vi "SubMatrixB.vi"(0 "Target Field, T":dbl=1.0 min=-4.0 max=4.0 step=0.1 format="%.4f", 2 "Sweep rate, T/min":dbl=0.1 min=0.0 max=1.0 step=0.01 format="%.4f", 3 "Custom Folder":string, 4 "Time Stamp":timestamp) -> ()   [LabVIEW 2015]
uses:
  <vilib>/Utility/file.llb/Write To Spreadsheet File (DBL).vi
panel:
  out "IndexB":i32
  out "PrevB":dbl
  out "Communication":string
  out "Comments":string[](array[string])
  out "ArrayBoolian":bool[][](array[boolean])
  out "Numeric 4":i32
  in  "Commutator":bool
  in  "Commute SorceMeter":enum32{"Radio Selection 1", "Radio Selection 2"}(radio)
  out "Numeric 3":i32
  in  "Channel 2 (Vnano3b)":bool
  in  "Channel 1 (Vnano3)":bool
  out "Numeric":i32
  in  "Capacitance (C) and Loss (L)":bool
  in  "Magnetic Field (B)":bool=TRUE
  in  "Current (Ik3)":bool
  in  "Voltage (Vk3)":bool
  in  "Current (Ik2)":bool
  in  "Voltage (Vk2)":bool
  in  "Channel 2 (Vnano2b)":bool
  in  "Channel 1 (Vnano2)":bool
  in  "Thermometer 1 (T1)":bool=TRUE
  in  "Channel 2 (Vnano1b)":bool
  in  "Channel 1 (Vnano1)":bool
  in  "Current (Ik1)":bool=TRUE
  in  "Voltage (Vk1)":bool=TRUE
  out "Numeric Current":dbl
  out "Delib Time delay":i32=500
  in  "points at each Vg":i32=1
  out "XY Graph":cluster{dbl[], dbl[]}(graph)={[1.0, 0.8, 0.6000000000000001, 0.4000000000000001, 0.20000000000000007, 5.551115123125783e-17, -0.19999999999999996, -0.39999999999999997, -0.6, -0.8, -1.0], [0.03352775, 0.056811, 0.03911575, 0.04330675, -0.02468015, 0.011641600000000002, 0.10151450000000001, 0.12386675000000001, 0.08288825000000001, -0.00186266, -0.038650000000000004]}
  in  "Time btw \npoints, sec":dbl=1.0 format="%.2f"
  out "Array 2":dbl[][](array[numeric])
  out "array for data":dbl[](array[numeric])
  out "Array":string[](array[string])
  in  "Addr 1 lock-in oop":bool=TRUE
  in  "Ring":u16(ring) caption="Y-axis:" items=["B0", "I", "R1", "R1oop", "Vk1", "Ik1", "T1", "B"]
  out "String":string
  out "Data file:":path
  in  "error in (no error)":errorcluster
  in  "Ring 3":u16(ring)=1 items=["1 kOhm", "10 kOhm", "100 kOhm", "1 Mohm", "10 mOhm"]
  in  "Ring 2":u16(ring)=4 items=["1 kOhm", "10 kOhm", "100 kOhm", "1 Mohm", "10 mOhm"]
  in  "Fixed Current mkA":dbl=1.0
  in  "Current is:":T1(radio)
  in  "Ressitance measurements?":bool=TRUE
  in  "Addr 5 lock-in oop":bool
  in  "Addr 4 lock-in oop":bool
  in  "Addr 3 lock-in oop":bool
  in  "Addr 2 lock-in oop":bool
  in  "Addr 5 lock-in":bool
  in  "Addr 4 lock-in":bool
  in  "Addr 3 lock-in":bool
  in  "Addr 2 lock-in":bool
  in  "Addr 1 lock-in":bool=TRUE
  # "Keithley 2400: address 12"
  # "0"
  # "SourceMeters"
  # "Nanovoltmeters"
  # "Temperature"
  # "Main"
  # "Magnetic Field"
  # "(not recommended, too slow)"
  # "Capacitance & Loss"
  # "(not recommended, too slow)"
  # "(not recommended, too slow)"
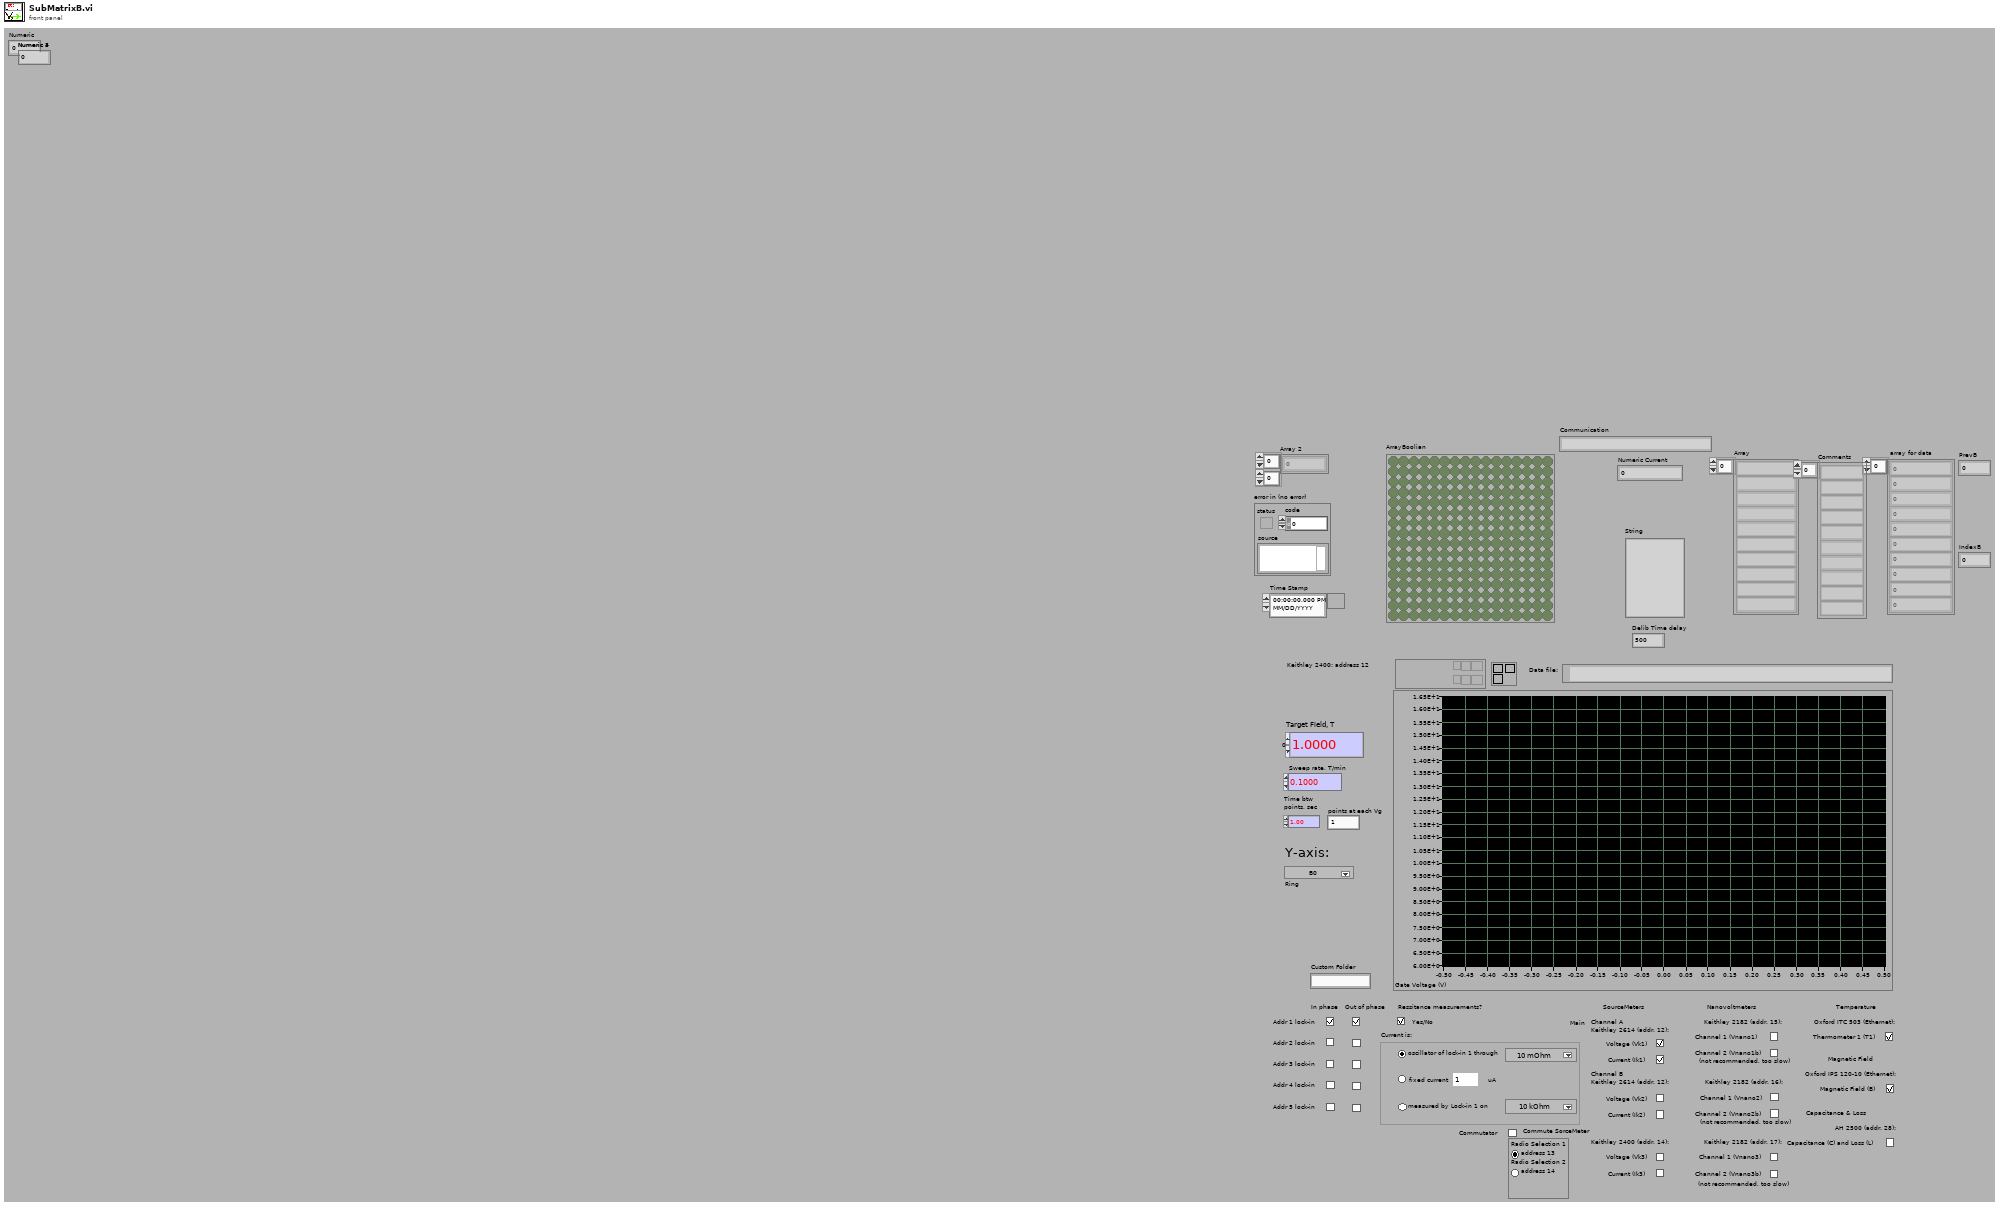
[diagram p1: front panel]
types:
  T1 = enum32{"Radio Selection 1", "Radio Selection 2", "Radio Selection 3"}
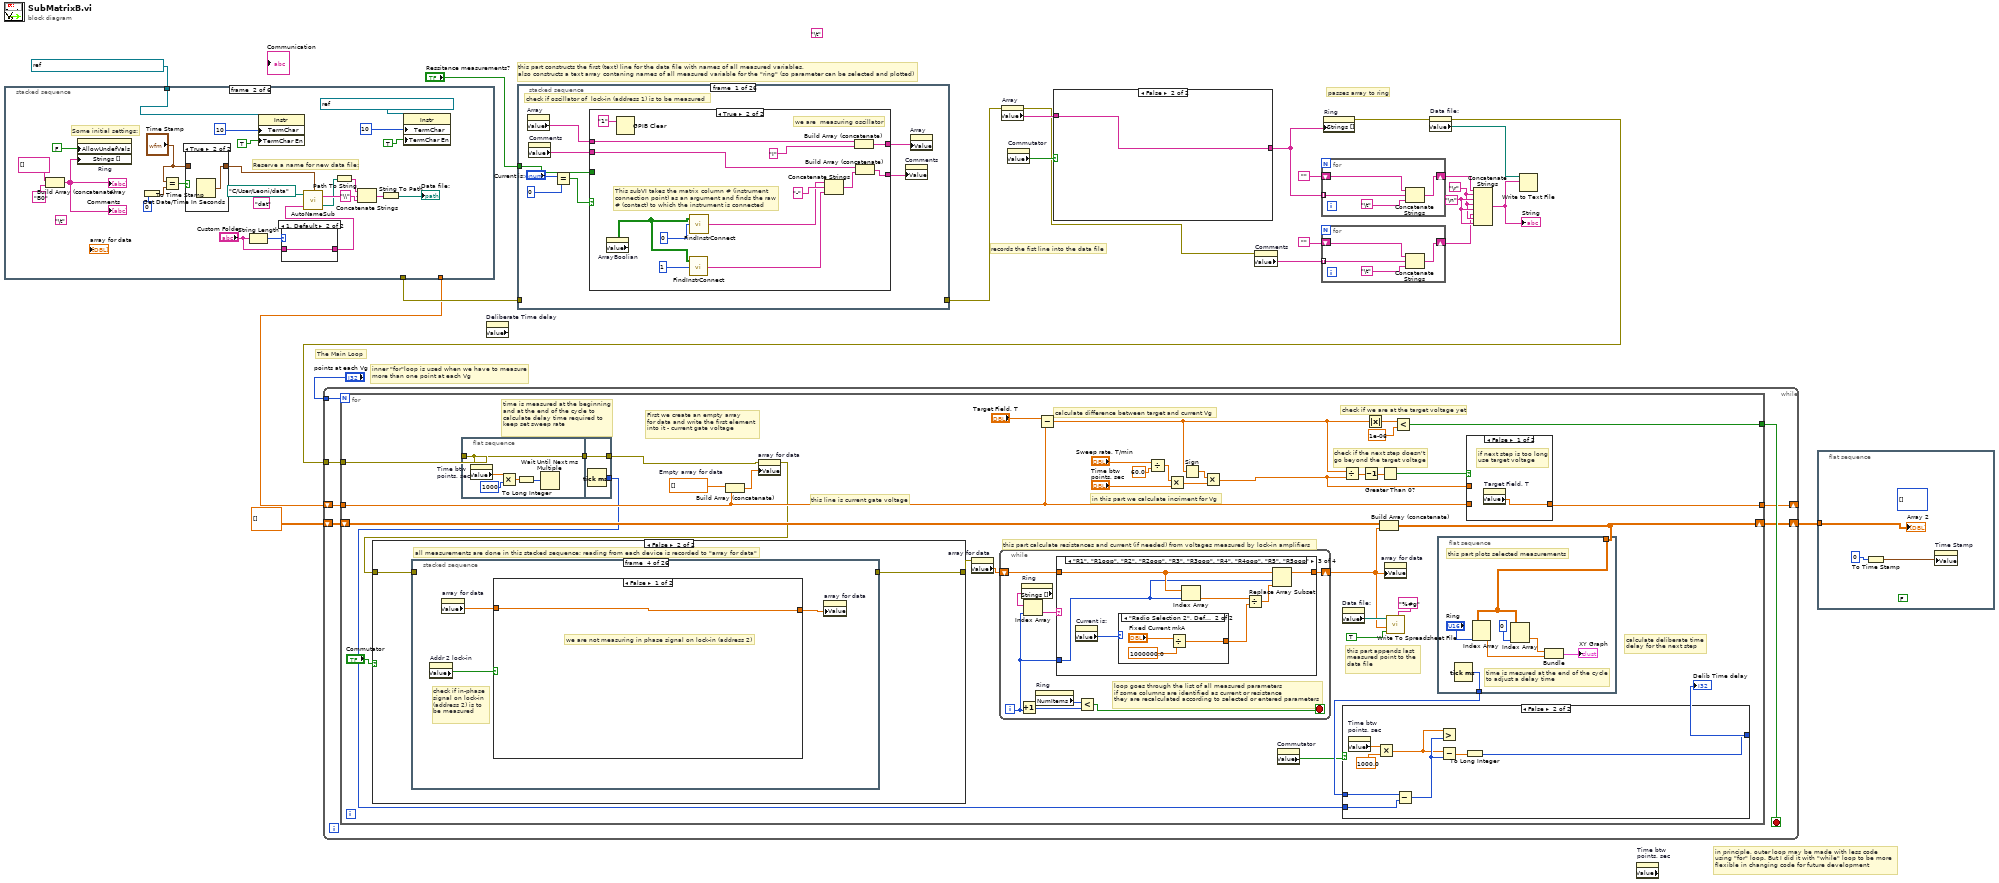
[diagram p0: block diagram]
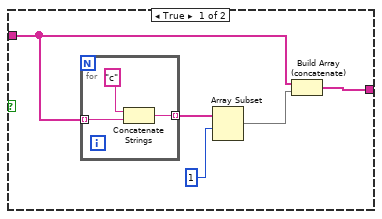
[diagram p2: hidden frame]
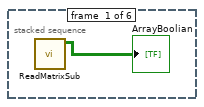
[diagram p3: hidden frame]
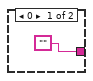
[diagram p5: hidden frame]
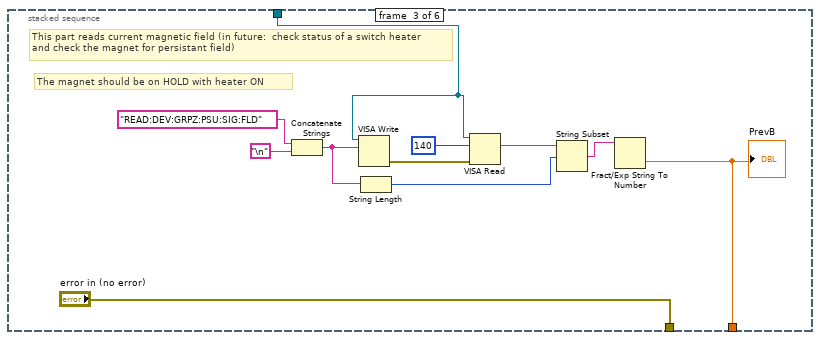
[diagram p6: hidden frame]
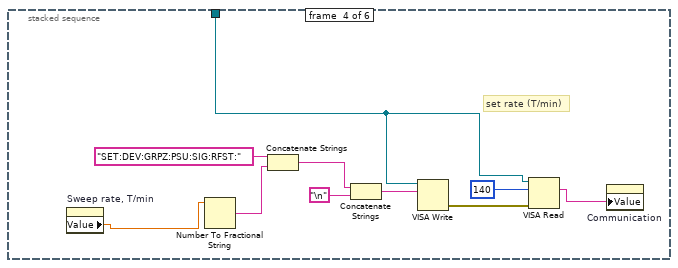
[diagram p7: hidden frame]
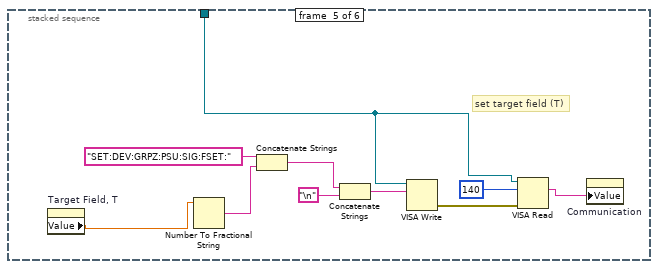
[diagram p8: hidden frame]
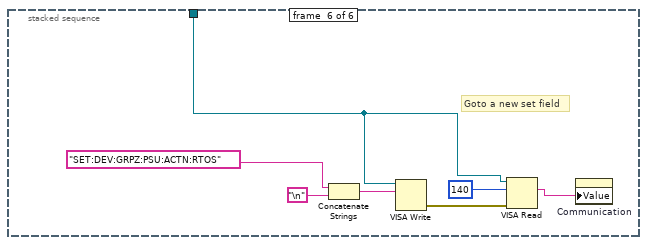
[diagram p9: hidden frame]
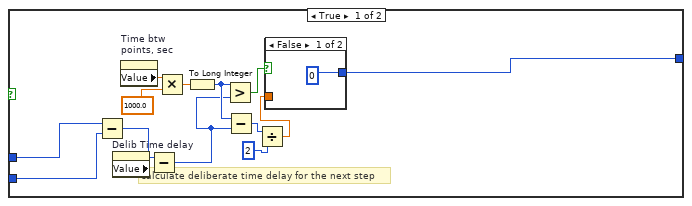
[diagram p10: hidden frame]
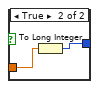
[diagram p11: hidden frame]
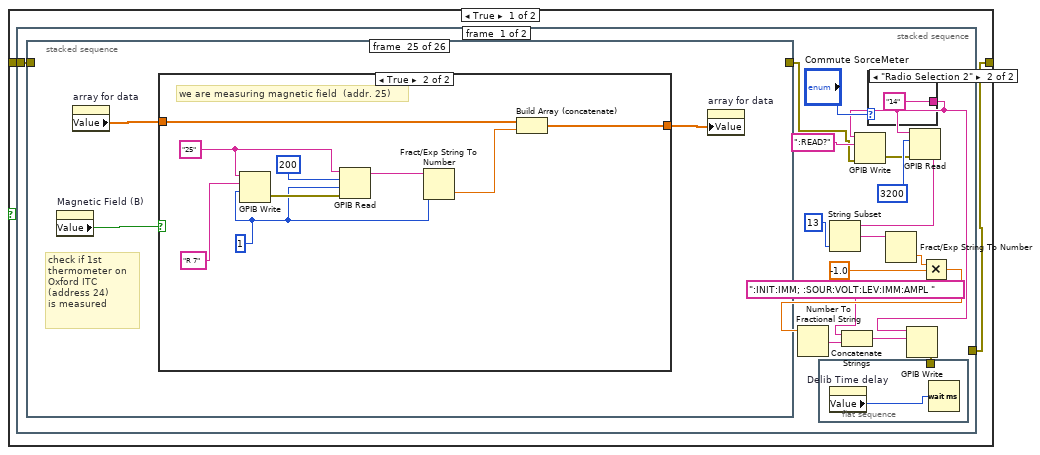
[diagram p12: hidden frame]
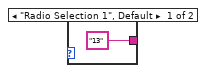
[diagram p13: hidden frame]
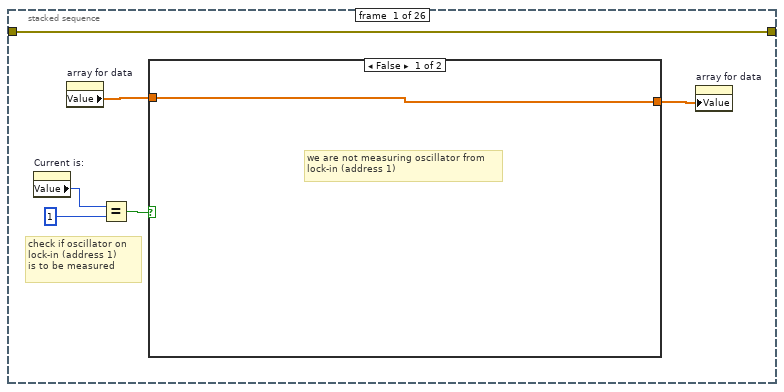
[diagram p14: hidden frame]
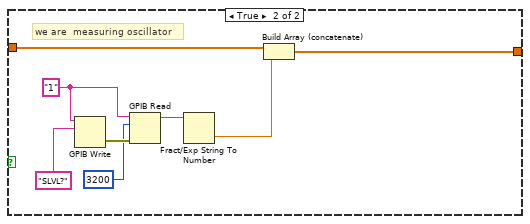
[diagram p15: hidden frame]
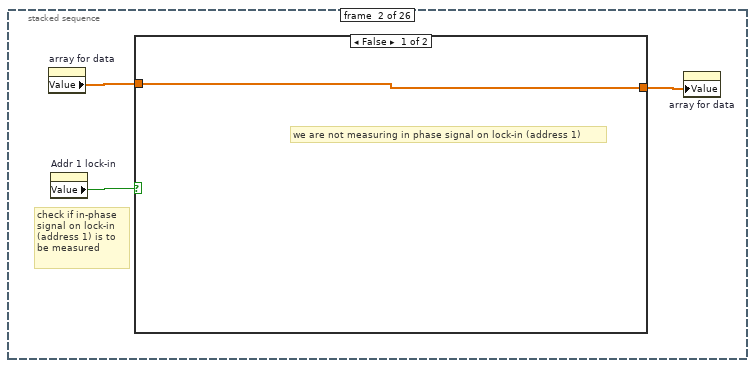
[diagram p16: hidden frame]
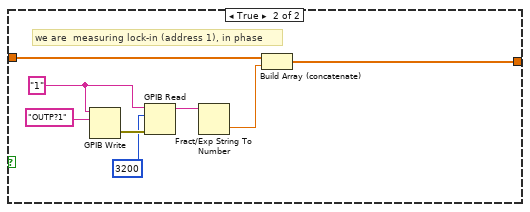
[diagram p17: hidden frame]
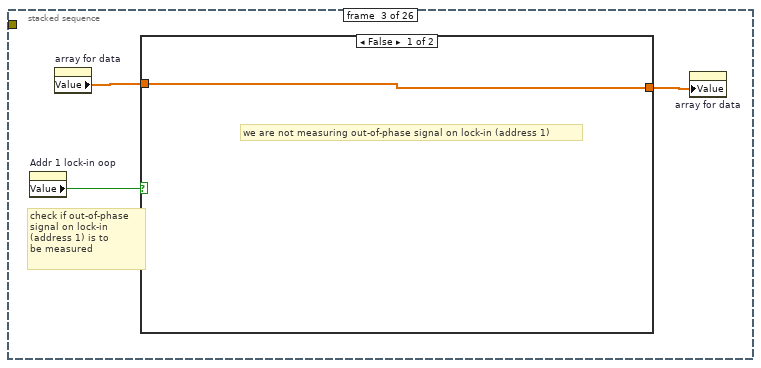
[diagram p18: hidden frame]
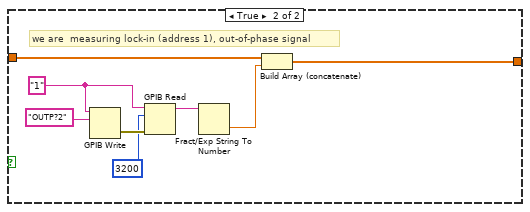
[diagram p19: hidden frame]
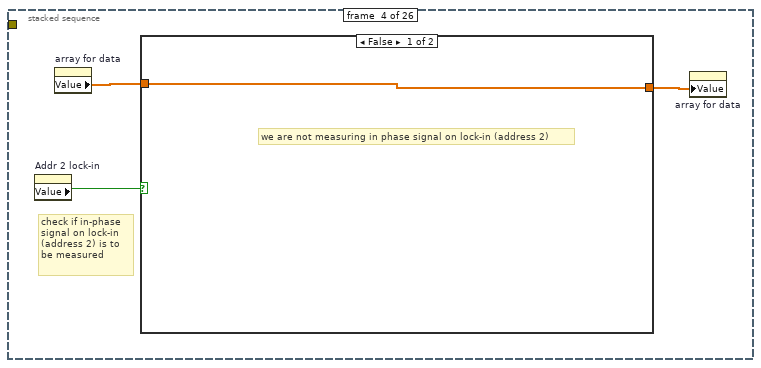
[diagram p20: hidden frame]
diagram:
  (unwired) "\t"
  w5 = "\r"
  w6 = "\n"
  # "passes array to ring"
  # "in principle, outer loop may be made with less code\nusing \"for\" loop. But I did it with \"while\" loop to be more \nflexible in changing code for future development"
  # "inner \"for\"loop is used when we have to measure\nmore than one point at each Vg"
  # "The Main Loop"
  # "records the fist line into the data file"
  # "this part constructs the first (text) line for the data file with names of all measured variables,\nalso constructs a text array contaning names of all measured variable for the \"ring\" (so parameter can be selected and plotted)"
  n1 = stacked-sequence {
    tunnel: [_ _ "error in (no error)" _ _ _] -> w23
    tunnel: refnum<visa-resource-name> "TCPIP0::192.168.128.3::7020::SOCKET" ("VISA resource name") -> [_ w30 w55 w66 w77 w87]
    tunnel: [_ _ w54 _ _ _] -> w1
    frame #0 {
      n2 = call "ReadMatrixSub.vi"() -> ("Array"=→"ArrayBoolian":bool[][])  [unwired: 9 in, 2 out]
    }
    frame #1 {
      (unwired) "dat"
      (unwired) "\t"
      # "Some initial settings:"
      # "Reserve a name for new data file:"
      n3 = Build Array (concatenate)(string[] [], "B0") -> (w31:string[])
      "Array" <- w31
      "Comments" <- w31
      n4 = property on="Ring" class="Ring (strict)"("AllowUndefVals"=FALSE, "Strings []"=w31) -> ()  [unwired: 2 in, 2 out]
      n5 = To Time Stamp(1:0) -> (0:w28:timestamp)
      n6 = Equal?(x="Time Stamp", y=w28) -> (x = y?=w29:bool)
      n7 = case shown="True" w29 {
        tunnel: "Time Stamp" -> [w50 _]
        tunnel: [w50 w51] -> w25
        frame False {
        }
        frame True {
          n8 = Get Date/Time In Seconds() -> (seconds since 1Jan1904=w51:timestamp)
        }
      }
      n9 = String Length(string="Custom Folder") -> (length=w40:i32)
      n10 = property class="Instr"(reference=w30, "TermChar"=10, "TermChar En"=TRUE) -> ()  [unwired: 1 in, 2 out]
      n11 = case shown="1, Default" w40 {
        tunnel: "Custom Folder" -> [_ w53]
        tunnel: ["" w53] -> w38
        frame 0 {
        }
        frame 1, Default {
        }
      }
      n12 = call "AutoNameSub.vi"("Time Stamp"=w25, "Custom Folder"=w38, "User Data Folder"=path "C:/User/Leoni/data") -> ("created path"=w48:path, "String"=w49:string)  [unwired: 1 in]
      n13 = Path To String(path=w48) -> (string=w43:string)
      n14 = Concatenate Strings(w43, "\\", w49) -> (w45:string)
      n15 = String To Path(string=w45) -> (path=→"Data file:":path)
      n16 = property class="Instr"(reference=refnum<visa-resource-name> "TCPIP0::192.168.128.2::7020::SOCKET" ("VISA resource name"), "TermChar"=10, "TermChar En"=TRUE) -> ()  [unwired: 1 in, 2 out]
    }
    frame #2 {
      # "The magnet should be on HOLD with heater ON"
      # "This part reads current magnetic field (in future:  check status of a switch heater\nand check the magnet for persistant field)"
      n17 = Concatenate Strings("READ:DEV:GRPZ:PSU:SIG:FLD" ("string"), "\n") -> (w59:string)
      n18 = VISA Write(VISA resource name=w55, write buffer=w59) -> (error out=w63:errorcluster)  [unwired: 1 in, 2 out]
      n19 = String Length(string=w59) -> (length=w57:i32)
      n20 = VISA Read(VISA resource name=w55, byte count=140, error in (no error)=w63) -> (read buffer=w58:string)  [unwired: 3 out]
      n21 = String Subset(string=w58, offset (0)=w57) -> (substring=w56:string)  [unwired: 1 in]
      n22 = Fract/Exp String To Number(string=w56) -> (number=w54:dbl)  [unwired: 3 in, 1 out]
      "PrevB" <- w54
    }
    frame #3 {
      # "set rate (T/min)"
      n23 = property on="Sweep rate, T/min" class="DigNum (strict)"() -> ("Value"=w67:dbl)  [unwired: 2 in, 2 out]
      n24 = Number To Fractional String(number=w67) -> (F-format string=w73:string)  [unwired: 3 in]
      n25 = Concatenate Strings("SET:DEV:GRPZ:PSU:SIG:RFST:" ("string"), w73) -> (w68:string)
      n26 = Concatenate Strings(w68, "\n") -> (w69:string)
      n27 = VISA Write(VISA resource name=w66, write buffer=w69) -> (error out=w72:errorcluster)  [unwired: 1 in, 2 out]
      n28 = VISA Read(VISA resource name=w66, byte count=140, error in (no error)=w72) -> (read buffer=w65:string)  [unwired: 3 out]
      n29 = property on="Communication" class="Str"("Value"=w65) -> ()  [unwired: 2 in, 2 out]
    }
    frame #4 {
      # "set target field (T)"
      n30 = property on="Target Field, T" class="DigNum (strict)"() -> ("Value"=w76:dbl)  [unwired: 2 in, 2 out]
      n31 = Number To Fractional String(number=w76) -> (F-format string=w83:string)  [unwired: 3 in]
      n32 = Concatenate Strings("SET:DEV:GRPZ:PSU:SIG:FSET:" ("string"), w83) -> (w78:string)
      n33 = Concatenate Strings(w78, "\n") -> (w79:string)
      n34 = VISA Write(VISA resource name=w77, write buffer=w79) -> (error out=w82:errorcluster)  [unwired: 1 in, 2 out]
      n35 = VISA Read(VISA resource name=w77, byte count=140, error in (no error)=w82) -> (read buffer=w75:string)  [unwired: 3 out]
      n36 = property on="Communication" class="Str"("Value"=w75) -> ()  [unwired: 2 in, 2 out]
    }
    frame #5 {
      # "Goto a new set field"
      n37 = Concatenate Strings("SET:DEV:GRPZ:PSU:ACTN:RTOS" ("string"), "\n") -> (w88:string)
      n38 = VISA Write(VISA resource name=w87, write buffer=w88) -> (error out=w91:errorcluster)  [unwired: 1 in, 2 out]
      n39 = VISA Read(VISA resource name=w87, byte count=140, error in (no error)=w91) -> (read buffer=w86:string)  [unwired: 3 out]
      n40 = property on="Communication" class="Str"("Value"=w86) -> ()  [unwired: 2 in, 2 out]
    }
  }
  n41 = property on="Deliberate Time delay" class="DigNum (strict)" props=["Value"]() -> ()  [unwired: 2 in, 3 out]
  n42 = stacked-sequence {
    tunnel: "Ressitance measurements?" -> [w99 w120 w147 w164 w184 w196 w208 w220 w232 w244 w256 _ _ _ _ _ _ _ _ _ _ _ _ _ _ _]
    tunnel: w23 -> [_ w119 _ _ _ _ _ _ _ _ _ _ _ _ _ _ _ _ _ _ _ _ _ _ _ _]
    tunnel: [_ w119 _ _ _ _ _ _ _ _ _ _ _ _ _ _ _ _ _ _ _ _ _ _ _ _] -> w20
    frame #0 {
      # "check if oscillator of  lock-in (address 1) is to be measured"
      n43 = property on="Array" class="Arr (strict)"() -> ("Value"=w95:string[])  [unwired: 2 in, 2 out]
      n44 = property on="Comments" class="Arr (strict)"() -> ("Value"=w92:string[])  [unwired: 2 in, 2 out]
      n45 = Equal?(x="Current is:", y=0) -> (x = y?=w97:bool)
      n46 = case shown="True" w97 {
        tunnel: w99 -> [_ _]
        tunnel: w95 -> [w101 w112]
        tunnel: [w101 w111] -> w94
        tunnel: [w100 w104] -> w93
        tunnel: w92 -> [w100 w103]
        frame False {
          # "we are not measuring oscillator from\nlock-in (address 1)"
        }
        frame True {
          # "This subVI takes the matrix column # (instrument\nconnection point) as an argument and finds the raw\n# (contact) to which the instrument is connected"
          # "we are  measuring oscillator"
          n47 = property on="ArrayBoolian" class="Arr (strict)"() -> ("Value"=w108:bool[][])  [unwired: 2 in, 2 out]
          n48 = GPIB Clear(3:"1") -> ()  [unwired: 1 in, 2 out]
          n49 = call "FindInstrConnect.vi"("Column #"=1, "ArrayBoolian"=w108) -> ("String"=w109:string)  [unwired: 1 in, 2 out]
          n50 = call "FindInstrConnect.vi"("Column #"=0, "ArrayBoolian"=w108) -> ("String"=w106:string)  [unwired: 1 in, 2 out]
          n51 = Concatenate Strings(w106, "-", w109) -> (w102:string)
          n52 = Build Array (concatenate)(w112, "I") -> (w111:string[])
          n53 = Build Array (concatenate)(w103, w102) -> (w104:string[])
        }
      }
      n54 = property on="Comments" class="Arr (strict)"("Value"=w93) -> ()  [unwired: 2 in, 2 out]
      n55 = property on="Array" class="Arr (strict)"("Value"=w94) -> ()  [unwired: 2 in, 2 out]
    }
    frame #1 {
      # "check if lock-in (address 1) is to be measured"
      n56 = property on="Array" class="Arr (strict)"() -> ("Value"=w118:string[])  [unwired: 2 in, 2 out]
      n57 = property on="Comments" class="Arr (strict)"() -> ("Value"=w116:string[])  [unwired: 2 in, 2 out]
      n58 = case shown="True" "Addr 1 lock-in" {
        tunnel: w120 -> [_ w136]
        tunnel: w118 -> [w123 w134]
        tunnel: [w123 w135] -> w117
        tunnel: w116 -> [w122 w125]
        tunnel: [w122 w126] -> w115
        frame False {
          # "we are not measuring in phase signal from\nlock-in (address 1)"
        }
        frame True {
          # "are we measuring resistance?"
          n59 = case shown="True" w136 {
            tunnel: ["V1" w138] -> w127
            frame False {
              # "no, we are not measuring resistanse;\nall lock-ins are measuring voltage"
            }
            frame True {
              # "are we measuring current as well?"
              n60 = property on="Current is:" class="RadioBtnsControl (strict)"() -> ("Value"=w140:T1)  [unwired: 2 in, 2 out]
              n61 = Equal?(x=w140, y=2) -> (x = y?=w141:bool)
              n62 = case shown="True" w141 {
                tunnel: ["R1" "I"] -> w138
                frame False {
                  # "no, we are not \nmeasuring current\nby lock-in \n(address 1); \nso this lock-in is \nmeasuring resistance"
                }
                frame True {
                  # "yes, we are measuring \ncurrent by lock-in \n(address 1) as \nvoltage drop on \nknown resistance"
                }
              }
            }
          }
          n63 = property on="ArrayBoolian" class="Arr (strict)"() -> ("Value"=w128:bool[][])  [unwired: 2 in, 2 out]
          n64 = call "FindInstrConnect.vi"("Column #"=3, "ArrayBoolian"=w128) -> ("String"=w131:string)  [unwired: 1 in, 2 out]
          n65 = call "FindInstrConnect.vi"("Column #"=2, "ArrayBoolian"=w128) -> ("String"=w129:string)  [unwired: 1 in, 2 out]
          n66 = Concatenate Strings(w129, "-", w131) -> (w124:string)
          n67 = Build Array (concatenate)(w134, w127) -> (w135:string[])
          n68 = Build Array (concatenate)(w125, w124) -> (w126:string[])
        }
      }
      n69 = property on="Array" class="Arr (strict)"("Value"=w117) -> ()  [unwired: 2 in, 2 out]
      n70 = property on="Comments" class="Arr (strict)"("Value"=w115) -> ()  [unwired: 2 in, 2 out]
    }
    frame #2 {
      # "check if out-of-phase signal on  lock-in (address 1) is to be measured"
      n71 = property on="Array" class="Arr (strict)"() -> ("Value"=w146:string[])  [unwired: 2 in, 2 out]
      n72 = case shown="True" "Addr 1 lock-in oop" {
        tunnel: w147 -> [_ w153]
        tunnel: w146 -> [w148 w150]
        tunnel: [w148 w151] -> w145
        frame False {
          # "we are not measuring iout-of-phase signal from\nlock-in (address 1)"
        }
        frame True {
          # "are we measuring resistance?"
          n73 = GPIB Clear(3:"1") -> ()  [unwired: 1 in, 2 out]
          n74 = case shown="True" w153 {
            tunnel: ["V1oop" w155] -> w149
            frame False {
              # "no, we are not measuring resistance;\nall lock-ins are measuring voltage"
            }
            frame True {
              # "are we measuring out-of-phase current as well?"
              n75 = property on="Current is:" class="RadioBtnsControl (strict)"() -> ("Value"=w157:T1)  [unwired: 2 in, 2 out]
              n76 = Equal?(x=w157, y=2) -> (x = y?=w158:bool)
              n77 = case shown="False" w158 {
                tunnel: ["R1oop" "Ioop"] -> w155
                frame False {
                  # "no, we are not \nmeasuring current\nby lock-in \n(address 1); so this \nlock-in is measuring\nout-of-phase resistance"
                }
                frame True {
                  # "yes, we are measuring \nout-of phase current \nby lock-in (address 1) \nas voltage drop on \nknown resistance"
                }
              }
            }
          }
          n78 = Build Array (concatenate)(w150, w149) -> (w151:string[])
        }
      }
      n79 = property on="Array" class="Arr (strict)"("Value"=w145) -> ()  [unwired: 2 in, 2 out]
    }
    frame #3 {
      # "check if in-phase signal on  lock-in (address 2) is to be measured"
      n80 = property on="Array" class="Arr (strict)"() -> ("Value"=w163:string[])  [unwired: 2 in, 2 out]
      n81 = case shown="False" "Addr 2 lock-in" {
        tunnel: w164 -> [_ w178]
        tunnel: w163 -> [w165 w175]
        tunnel: [w165 w176] -> w162
        frame False {
          # "we are not measuring in-phase signal from\nlock-in (address 2)"
        }
        frame True {
          (unwired) "\t"
          # "are we measuring resistance?"
          n82 = GPIB Clear(3:"2") -> ()  [unwired: 1 in, 2 out]
          n83 = case shown="False" w178 {
            tunnel: ["R2 (" "V2 ("] -> w167
            frame True {
              # "we are measuring \nresistance by lock-in \n(address 2)"
            }
            frame False, Default {
              # "no, we are not \nmeasuring resistance;\nall lock-ins are \nmeasuring voltage"
            }
          }
          n84 = property on="ArrayBoolian" class="Arr (strict)"() -> ("Value"=w166:bool[][])  [unwired: 2 in, 2 out]
          n85 = call "FindInstrConnect.vi"("Column #"=5, "ArrayBoolian"=w166) -> ("String"=w171:string)  [unwired: 1 in, 2 out]
          n86 = call "FindInstrConnect.vi"("Column #"=4, "ArrayBoolian"=w166) -> ("String"=w169:string)  [unwired: 1 in, 2 out]
          n87 = Concatenate Strings(w167, w169, "-", w171, ")") -> (w168:string)
          n88 = Build Array (concatenate)(w175, w168) -> (w176:string[])
        }
      }
      n89 = property on="Array" class="Arr (strict)"("Value"=w162) -> ()  [unwired: 2 in, 2 out]
    }
    frame #4 {
      # "check if out-of-phase signal on  lock-in (address 2) is to be measured"
      n90 = property on="Array" class="Arr (strict)"() -> ("Value"=w183:string[])  [unwired: 2 in, 2 out]
      n91 = case shown="False" "Addr 2 lock-in oop" {
        tunnel: w184 -> [_ w190]
        tunnel: w183 -> [w185 w187]
        tunnel: [w185 w188] -> w182
        frame False {
          # "we are not measuring out-of-phase signal from\nlock-in (address 2)"
        }
        frame True {
          (unwired) "\t"
          # "are we measuring resistance?"
          n92 = GPIB Clear(3:"2") -> ()  [unwired: 1 in, 2 out]
          n93 = case shown="True" w190 {
            tunnel: ["R2oop" "V2oop"] -> w186
            frame True {
              # "we are measuring out-of-phase resistance by lock-in (address 2)\n(address 2)"
            }
            frame False, Default {
              # "no, we are not measuring resistance;\nall lock-ins are measuring voltage"
            }
          }
          n94 = Build Array (concatenate)(w187, w186) -> (w188:string[])
        }
      }
      n95 = property on="Array" class="Arr (strict)"("Value"=w182) -> ()  [unwired: 2 in, 2 out]
    }
    frame #5 {
      # "check if in-phase signal on  lock-in (address 3) is to be measured"
      n96 = property on="Array" class="Arr (strict)"() -> ("Value"=w195:string[])  [unwired: 2 in, 2 out]
      n97 = case shown="False" "Addr 3 lock-in" {
        tunnel: w196 -> [_ w202]
        tunnel: w195 -> [w197 w199]
        tunnel: [w197 w200] -> w194
        frame False {
          # "we are not measuring in-phase signal from\nlock-in (address 3)"
        }
        frame True {
          (unwired) "\t"
          # "are we measuring resistance?"
          n98 = GPIB Clear(3:"3") -> ()  [unwired: 1 in, 2 out]
          n99 = case shown="True" w202 {
            tunnel: ["R3" "V3"] -> w198
            frame True {
              # "we are measuring \nresistance by lock-in \n(address 3)"
            }
            frame False, Default {
              # "no, we are not measuring resistance;\nall lock-ins are measuring voltage"
            }
          }
          n100 = Build Array (concatenate)(w199, w198) -> (w200:string[])
        }
      }
      n101 = property on="Array" class="Arr (strict)"("Value"=w194) -> ()  [unwired: 2 in, 2 out]
    }
    frame #6 {
      # "check if out-of-phase signal on  lock-in (address 3) is to be measured"
      n102 = property on="Array" class="Arr (strict)"() -> ("Value"=w207:string[])  [unwired: 2 in, 2 out]
      n103 = case shown="False" "Addr 3 lock-in oop" {
        tunnel: w208 -> [_ w214]
        tunnel: w207 -> [w209 w211]
        tunnel: [w209 w212] -> w206
        frame False {
          # "we are not measuring out-of-phase signal from\nlock-in (address 3)"
        }
        frame True {
          (unwired) "\t"
          # "are we measuring resistance?"
          n104 = GPIB Clear(3:"3") -> ()  [unwired: 1 in, 2 out]
          n105 = case shown="True" w214 {
            tunnel: ["R3oop" "V3oop"] -> w210
            frame True {
              # "we are measuring out-of-phase resistance by lock-in (address 3)\n(address 2)"
            }
            frame False, Default {
              # "no, we are not measuring resistance;\nall lock-ins are measuring voltage"
            }
          }
          n106 = Build Array (concatenate)(w211, w210) -> (w212:string[])
        }
      }
      n107 = property on="Array" class="Arr (strict)"("Value"=w206) -> ()  [unwired: 2 in, 2 out]
    }
    frame #7 {
      # "check if in-phase signal on  lock-in (address 4) is to be measured"
      n108 = property on="Array" class="Arr (strict)"() -> ("Value"=w219:string[])  [unwired: 2 in, 2 out]
      n109 = case shown="False" "Addr 4 lock-in" {
        tunnel: w220 -> [_ w226]
        tunnel: w219 -> [w221 w223]
        tunnel: [w221 w224] -> w218
        frame False {
          # "we are not measuring in-phase signal from\nlock-in (address 4)"
        }
        frame True {
          (unwired) "\t"
          # "are we measuring resistance?"
          n110 = GPIB Clear(3:"4") -> ()  [unwired: 1 in, 2 out]
          n111 = case shown="True" w226 {
            tunnel: ["R4" "V4"] -> w222
            frame True {
              # "we are measuring \nresistance by lock-in \n(address 4)"
            }
            frame False, Default {
              # "no, we are not measuring resistance;\nall lock-ins are measuring voltage"
            }
          }
          n112 = Build Array (concatenate)(w223, w222) -> (w224:string[])
        }
      }
      n113 = property on="Array" class="Arr (strict)"("Value"=w218) -> ()  [unwired: 2 in, 2 out]
    }
    frame #8 {
      # "check if out-of-phase signal on  lock-in (address 4) is to be measured"
      n114 = property on="Array" class="Arr (strict)"() -> ("Value"=w231:string[])  [unwired: 2 in, 2 out]
      n115 = case shown="False" "Addr 4 lock-in oop" {
        tunnel: w232 -> [_ w238]
        tunnel: w231 -> [w233 w235]
        tunnel: [w233 w236] -> w230
        frame False {
          # "we are not measuring out-of-phase signal from\nlock-in (address 4)"
        }
        frame True {
          (unwired) "\t"
          # "are we measuring resistance?"
          n116 = GPIB Clear(3:"4") -> ()  [unwired: 1 in, 2 out]
          n117 = case shown="True" w238 {
            tunnel: ["R4oop" "V4oop"] -> w234
            frame True {
              # "we are measuring out-of-phase resistance by lock-in (address 4)\n(address 2)"
            }
            frame False, Default {
              # "no, we are not measuring resistance;\nall lock-ins are measuring voltage"
            }
          }
          n118 = Build Array (concatenate)(w235, w234) -> (w236:string[])
        }
      }
      n119 = property on="Array" class="Arr (strict)"("Value"=w230) -> ()  [unwired: 2 in, 2 out]
    }
    frame #9 {
      # "check if in-phase signal on  lock-in (address 5) is to be measured"
      n120 = property on="Array" class="Arr (strict)"() -> ("Value"=w243:string[])  [unwired: 2 in, 2 out]
      n121 = case shown="False" "Addr 5 lock-in" {
        tunnel: w244 -> [_ w250]
        tunnel: w243 -> [w245 w247]
        tunnel: [w245 w248] -> w242
        frame False {
          # "we are not measuring in-phase signal from\nlock-in (address 5)"
        }
        frame True {
          (unwired) "\t"
          # "are we measuring resistance?"
          n122 = GPIB Clear(3:"5") -> ()  [unwired: 1 in, 2 out]
          n123 = case shown="True" w250 {
            tunnel: ["R5" "V5"] -> w246
            frame True {
              # "we are measuring \nresistance by lock-in \n(address 5)"
            }
            frame False, Default {
              # "no, we are not measuring resistance;\nall lock-ins are measuring voltage"
            }
          }
          n124 = Build Array (concatenate)(w247, w246) -> (w248:string[])
        }
      }
      n125 = property on="Array" class="Arr (strict)"("Value"=w242) -> ()  [unwired: 2 in, 2 out]
    }
    frame #10 {
      # "check if out-of-phase signal on  lock-in (address 5) is to be measured"
      n126 = property on="Array" class="Arr (strict)"() -> ("Value"=w255:string[])  [unwired: 2 in, 2 out]
      n127 = case shown="False" "Addr 5 lock-in oop" {
        tunnel: w256 -> [_ w262]
        tunnel: w255 -> [w257 w259]
        tunnel: [w257 w260] -> w254
        frame False {
          # "we are not measuring out-of-phase signal from\nlock-in (address 5)"
        }
        frame True {
          (unwired) "\t"
          # "are we measuring resistance?"
          n128 = GPIB Clear(3:"5") -> ()  [unwired: 1 in, 2 out]
          n129 = case shown="True" w262 {
            tunnel: ["R5oop" "V5oop"] -> w258
            frame True {
              # "we are measuring out-of-phase resistance by lock-in (address 5)\n(address 2)"
            }
            frame False, Default {
              # "no, we are not measuring resistance;\nall lock-ins are measuring voltage"
            }
          }
          n130 = Build Array (concatenate)(w259, w258) -> (w260:string[])
        }
      }
      n131 = property on="Array" class="Arr (strict)"("Value"=w254) -> ()  [unwired: 2 in, 2 out]
    }
    frame #11 {
      # "check if voltage on main Keithley 2400 (addr. 12) is measured"
      n132 = property on="Array" class="Arr (strict)"() -> ("Value"=w267:string[])  [unwired: 2 in, 2 out]
      n133 = case shown="False" "Voltage (Vk1)" {
        tunnel: w267 -> [w268 w270]
        tunnel: [w268 w271] -> w266
        frame False {
          # "no , we aren't measuring voltage \non main Keithley 2400 (addr. 12)"
        }
        frame True {
          (unwired) "\t"
          # "yes , we are measuring voltage \non main Keithley 2400 (addr. 12)"
          n134 = GPIB Clear(3:"12") -> ()  [unwired: 1 in, 2 out]
          n135 = Build Array (concatenate)(w270, "Vk1") -> (w271:string[])
        }
      }
      n136 = property on="Array" class="Arr (strict)"("Value"=w266) -> ()  [unwired: 2 in, 2 out]
    }
    frame #12 {
      # "check if current on main Keithley 2400 (addr. 12) is measured"
      n137 = property on="Array" class="Arr (strict)"() -> ("Value"=w275:string[])  [unwired: 2 in, 2 out]
      n138 = case shown="True" "Current (Ik1)" {
        tunnel: w275 -> [w276 w278]
        tunnel: [w276 w279] -> w274
        frame False {
          # "no , we aren't measuring current\non main Keithley 2400 (addr. 12)"
        }
        frame True {
          (unwired) "\t"
          # "yes , we are measuring current \non main Keithley 2400 (addr. 12)"
          n139 = GPIB Clear(3:"12") -> ()  [unwired: 1 in, 2 out]
          n140 = Build Array (concatenate)(w278, "Ik1") -> (w279:string[])
        }
      }
      n141 = property on="Array" class="Arr (strict)"("Value"=w274) -> ()  [unwired: 2 in, 2 out]
    }
    frame #13 {
      # "check if voltage on additional Keithley 2400 (addr. 13) is measured"
      n142 = property on="Array" class="Arr (strict)"() -> ("Value"=w283:string[])  [unwired: 2 in, 2 out]
      n143 = case shown="False" "Voltage (Vk2)" {
        tunnel: w283 -> [w284 w286]
        tunnel: [w284 w287] -> w282
        frame False {
          # "no , we aren't measuring voltage \non Keithley 2400 (addr. 13)"
        }
        frame True {
          (unwired) "\t"
          # "yes , we are measuring voltage \non Keithley 2400 (addr. 13)"
          n144 = GPIB Clear(3:"13") -> ()  [unwired: 1 in, 2 out]
          n145 = Build Array (concatenate)(w286, "Vk2") -> (w287:string[])
        }
      }
      n146 = property on="Array" class="Arr (strict)"("Value"=w282) -> ()  [unwired: 2 in, 2 out]
    }
    frame #14 {
      # "check if current on additional Keithley 2400 (addr. 13) is measured"
      n147 = property on="Array" class="Arr (strict)"() -> ("Value"=w291:string[])  [unwired: 2 in, 2 out]
      n148 = case shown="False" "Current (Ik2)" {
        tunnel: w291 -> [w292 w294]
        tunnel: [w292 w295] -> w290
        frame False {
          # "no , we aren't measuring current\non Keithley 2400 (addr. 13)"
        }
        frame True {
          (unwired) "\t"
          # "yes , we are measuring current \non Keithley 2400 (addr. 13)"
          n149 = GPIB Clear(3:"13") -> ()  [unwired: 1 in, 2 out]
          n150 = Build Array (concatenate)(w294, "Ik2") -> (w295:string[])
        }
      }
      n151 = property on="Array" class="Arr (strict)"("Value"=w290) -> ()  [unwired: 2 in, 2 out]
    }
    frame #15 {
      # "check if voltage on additional Keithley 2400 (addr. 14) is measured"
      n152 = property on="Array" class="Arr (strict)"() -> ("Value"=w299:string[])  [unwired: 2 in, 2 out]
      n153 = case shown="False" "Voltage (Vk3)" {
        tunnel: w299 -> [w300 w302]
        tunnel: [w300 w303] -> w298
        frame False {
          # "no , we aren't measuring voltage \non Keithley 2400 (addr. 14)"
        }
        frame True {
          (unwired) "\t"
          # "yes , we are measuring voltage \non Keithley 2400 (addr. 14)"
          n154 = GPIB Clear(3:"14") -> ()  [unwired: 1 in, 2 out]
          n155 = Build Array (concatenate)(w302, "Vk3") -> (w303:string[])
        }
      }
      n156 = property on="Array" class="Arr (strict)"("Value"=w298) -> ()  [unwired: 2 in, 2 out]
    }
    frame #16 {
      # "check if current on additional Keithley 2400 (addr. 14) is measured"
      n157 = property on="Array" class="Arr (strict)"() -> ("Value"=w307:string[])  [unwired: 2 in, 2 out]
      n158 = case shown="False" "Current (Ik3)" {
        tunnel: w307 -> [w308 w310]
        tunnel: [w308 w311] -> w306
        frame False {
          # "no , we aren't measuring current\non Keithley 2400 (addr. 14)"
        }
        frame True {
          (unwired) "\t"
          # "yes , we are measuring current \non Keithley 2400 (addr. 14)"
          n159 = GPIB Clear(3:"14") -> ()  [unwired: 1 in, 2 out]
          n160 = Build Array (concatenate)(w310, "Ik3") -> (w311:string[])
        }
      }
      n161 = property on="Array" class="Arr (strict)"("Value"=w306) -> ()  [unwired: 2 in, 2 out]
    }
    frame #17 {
      # "check if 1st channel of nanovoltmeter Keithley 2182 (addr. 15) is measured"
      n162 = property on="Array" class="Arr (strict)"() -> ("Value"=w315:string[])  [unwired: 2 in, 2 out]
      n163 = case shown="False" "Channel 1 (Vnano1)" {
        tunnel: w315 -> [w316 w319]
        tunnel: [w316 w320] -> w314
        frame False {
          # "no , we are not measuring 1st channel\non Keithley 2182 (addr. 15)"
        }
        frame True {
          (unwired) "\t"
          # "yes , we are measuring 1st channel\non Keithley 2182 (addr. 15)"
          n164 = GPIB Clear(3:"15") -> ()  [unwired: 1 in, 2 out]
          n165 = Build Array (concatenate)(w319, "Vnano1") -> (w320:string[])
        }
      }
      n166 = property on="Array" class="Arr (strict)"("Value"=w314) -> ()  [unwired: 2 in, 2 out]
    }
    frame #18 {
      # "check if 2nd channel of nanovoltmeter Keithley 2182 (addr. 15) is measured"
      n167 = property on="Array" class="Arr (strict)"() -> ("Value"=w323:string[])  [unwired: 2 in, 2 out]
      n168 = case shown="False" "Channel 2 (Vnano1b)" {
        tunnel: w323 -> [w324 w326]
        tunnel: [w324 w327] -> w322
        frame False {
          # "no , we are not measuring 2nd channel\non Keithley 2182 (addr. 15)"
        }
        frame True {
          (unwired) "\t"
          # "yes , we are measuring 2nd channel\non Keithley 2182 (addr. 15)"
          n169 = GPIB Clear(3:"15") -> ()  [unwired: 1 in, 2 out]
          n170 = Build Array (concatenate)(w326, "Vnano1b") -> (w327:string[])
        }
      }
      n171 = property on="Array" class="Arr (strict)"("Value"=w322) -> ()  [unwired: 2 in, 2 out]
    }
    frame #19 {
      # "check if 1st channel of nanovoltmeter Keithley 2182 (addr. 16) is measured"
      n172 = property on="Array" class="Arr (strict)"() -> ("Value"=w331:string[])  [unwired: 2 in, 2 out]
      n173 = case shown="False" "Channel 1 (Vnano2)" {
        tunnel: w331 -> [w332 w335]
        tunnel: [w332 w336] -> w330
        frame False {
          # "no , we are not measuring 1st channel\non Keithley 2182 (addr. 16)"
        }
        frame True {
          (unwired) "\t"
          # "yes , we are measuring 1st channel\non Keithley 2182 (addr. 16)"
          n174 = GPIB Clear(3:"16") -> ()  [unwired: 1 in, 2 out]
          n175 = Build Array (concatenate)(w335, "Vnano2") -> (w336:string[])
        }
      }
      n176 = property on="Array" class="Arr (strict)"("Value"=w330) -> ()  [unwired: 2 in, 2 out]
    }
    frame #20 {
      # "check if 2nd channel of nanovoltmeter Keithley 2182 (addr. 16) is measured"
      n177 = property on="Array" class="Arr (strict)"() -> ("Value"=w339:string[])  [unwired: 2 in, 2 out]
      n178 = case shown="False" "Channel 2 (Vnano2b)" {
        tunnel: w339 -> [w340 w342]
        tunnel: [w340 w343] -> w338
        frame False {
          # "no , we are not measuring 2nd channel\non Keithley 2182 (addr. 16)"
        }
        frame True {
          (unwired) "\t"
          # "yes , we are measuring 2nd channel\non Keithley 2182 (addr. 16)"
          n179 = GPIB Clear(3:"16") -> ()  [unwired: 1 in, 2 out]
          n180 = Build Array (concatenate)(w342, "Vnano2b") -> (w343:string[])
        }
      }
      n181 = property on="Array" class="Arr (strict)"("Value"=w338) -> ()  [unwired: 2 in, 2 out]
    }
    frame #21 {
      # "check if 1st channel of nanovoltmeter Keithley 2182 (addr. 17) is measured"
      n182 = property on="Array" class="Arr (strict)"() -> ("Value"=w347:string[])  [unwired: 2 in, 2 out]
      n183 = case shown="False" "Channel 1 (Vnano3)" {
        tunnel: w347 -> [w348 w350]
        tunnel: [w348 w351] -> w346
        frame False {
          # "no , we are not measuring 1st channel\non Keithley 2182 (addr. 17)"
        }
        frame True {
          (unwired) "\t"
          # "yes , we are measuring 1st channel\non Keithley 2182 (addr. 17)"
          n184 = GPIB Clear(3:"17") -> ()  [unwired: 1 in, 2 out]
          n185 = Build Array (concatenate)(w350, "Vnano3") -> (w351:string[])
        }
      }
      n186 = property on="Array" class="Arr (strict)"("Value"=w346) -> ()  [unwired: 2 in, 2 out]
    }
    frame #22 {
      # "check if 2nd channel of nanovoltmeter Keithley 2182 (addr. 16) is measured"
      n187 = property on="Array" class="Arr (strict)"() -> ("Value"=w355:string[])  [unwired: 2 in, 2 out]
      n188 = case shown="False" "Channel 2 (Vnano3b)" {
        tunnel: w355 -> [w356 w358]
        tunnel: [w356 w359] -> w354
        frame False {
          # "no , we are not measuring 2nd channel\non Keithley 2182 (addr. 17)"
        }
        frame True {
          (unwired) "\t"
          # "yes , we are measuring 2nd channel\non Keithley 2182 (addr. 17)"
          n189 = GPIB Clear(3:"17") -> ()  [unwired: 1 in, 2 out]
          n190 = Build Array (concatenate)(w358, "Vnano3b") -> (w359:string[])
        }
      }
      n191 = property on="Array" class="Arr (strict)"("Value"=w354) -> ()  [unwired: 2 in, 2 out]
    }
    frame #23 {
      # "check if 1st thermometer on Oxford ITC (address 24) is measured"
      n192 = property on="Array" class="Arr (strict)"() -> ("Value"=w363:string[])  [unwired: 2 in, 2 out]
      n193 = case shown="True" "Thermometer 1 (T1)" {
        tunnel: w363 -> [w364 w366]
        tunnel: [w364 w367] -> w362
        frame False {
          # "no, we are not measuring temperature\non thermometer 1 (addr. 24)"
        }
        frame True {
          (unwired) "\t"
          # "yes, we are measuring temperature,\nthermometer 1 (addr. 24)"
          n194 = GPIB Clear(3:"24") -> ()  [unwired: 1 in, 2 out]
          n195 = Build Array (concatenate)(w366, "T1") -> (w367:string[])
        }
      }
      n196 = property on="Array" class="Arr (strict)"("Value"=w362) -> ()  [unwired: 2 in, 2 out]
    }
    frame #24 {
      # "check if magnetic field from Oxford IPS 120 (address 25) is measured"
      n197 = property on="Array" class="Arr (strict)"() -> ("Value"=w371:string[])  [unwired: 2 in, 2 out]
      n198 = case shown="True" "Magnetic Field (B)" {
        tunnel: w371 -> [w372 w373]
        tunnel: [w372 w376] -> w370
        frame False {
          # "no, we are not measuring magnetic field  (addr. 25)"
        }
        frame True {
          (unwired) "\t"
          # "yes, we are measuring magnetic field  (addr. 25)"
          n199 = GPIB Clear(3:"25") -> ()  [unwired: 1 in, 2 out]
          n200 = Array Size(array=w373) -> (size(s)=→"IndexB":i32)
          n201 = Build Array (concatenate)(w373, "B") -> (w376:string[])
        }
      }
      n202 = property on="Array" class="Arr (strict)"("Value"=w370) -> ()  [unwired: 2 in, 2 out]
    }
    frame #25 {
      # "check if capacitance and loss from AH 2500 (address 28) are measured"
      n203 = property on="Array" class="Arr (strict)"() -> ("Value"=w380:string[])  [unwired: 2 in, 2 out]
      n204 = case shown="False" "Capacitance (C) and Loss (L)" {
        tunnel: w380 -> [w381 w383]
        tunnel: [w381 w386] -> w379
        frame False {
          # "no, we are not measuring capacitance  (addr. 28)"
        }
        frame True {
          (unwired) "\t"
          (unwired) "\t"
          # "yes, we are measuring capacitance and loss  (addr. 28)"
          n205 = GPIB Clear(3:"28") -> ()  [unwired: 1 in, 2 out]
          n206 = Build Array (concatenate)(w383, "C") -> (w382:string[])
          n207 = Build Array (concatenate)(w382, "L") -> (w386:string[])
        }
      }
      n208 = property on="Array" class="Arr (strict)"("Value"=w379) -> ()  [unwired: 2 in, 2 out]
    }
  }
  n209 = property on="Array" class="Arr (strict)"(error in=w20) -> (error out=w3:errorcluster, "Value"=w14:string[])  [unwired: 1 in, 1 out]
  n210 = property on="Commutator" class="Bool (strict)"() -> ("Value"=w13:bool)  [unwired: 2 in, 2 out]
  n211 = case shown="False" w13 {
    tunnel: w14 -> [w389 w396]
    tunnel: [w388 w396] -> w11
    frame True {
      n212 = for {
        tunnel: [w395] -> w392 mode=indexing
        tunnel: w389 -> [w393] mode=indexing
        n213 = Concatenate Strings("c", w393) -> (w395:string)
      }
      n214 = Array Subset(array=w392, index=1) -> (w390:string[])  [unwired: 1 in]
      n215 = Build Array (concatenate)(w389, w390) -> (w388:string[])
    }
    frame False {
    }
  }
  n216 = property on="Comments" class="Arr (strict)"(error in=w3) -> ("Value"=w7:string[])  [unwired: 1 in, 2 out]
  n217 = for {
    tunnel: w11 -> [w399] mode=indexing
    shift-right: [w397] -> w9
    shift-left: "" -> [w398]
    n218 = Concatenate Strings(w398, w399, "\t") -> (w397:string)
  }
  n219 = for {
    tunnel: w7 -> [w403] mode=indexing
    shift-right: [w401] -> w4
    shift-left: "" -> [w402]
    n220 = Concatenate Strings(w402, w403, "\t") -> (w401:string)
  }
  n221 = property on="Ring" class="Ring (strict)"("Strings []"=w11) -> (error out=w12:errorcluster)  [unwired: 2 in, 1 out]
  n222 = property on="Data file:" class="Path"(error in=w12) -> (error out=w17:errorcluster, "Value"=w19:path)  [unwired: 1 in, 1 out]
  n223 = while {
    tunnel: w17 -> [w411]
    shift-right: [w408] -> w16
    shift-left: dbl[][] [] -> [w410]
    shift-right: [w405] -> _
    shift-left: w1 -> [w407]
    tunnel: "points at each Vg" -> [w406]
    stop <- w409 stop-if-true
    n224 = for {
      N: w406 -> [_]
      tunnel: w411 -> [w419]
      tunnel: [w433] -> w409
      shift-right: [w420] -> w408
      shift-left: w410 -> [w446]
      tunnel: w407 -> [w431]
      tunnel: [w438] -> w405
      w432 = dbl[] []  # Empty array for data
      # "calculate deliberate time \ndelay for the next step"
      # "this part appends last\nmeasured point to the \ndata file"
      # "this line is current gate voltage"
      # "First we create an empty array \nfor data and write the first element \ninto it - current gate voltage"
      # "time is measured at the beginning\nand at the end of the cycle to\ncalculate delay time required to\nkeep set sweep rate"
      # "this part calculate resistances and current (if needed) from voltages measured by lock-in amplifiers"
      # "check if the next step doesn't\ngo beyond the target voltage"
      # "calculate difference between target and current Vg"
      # "check if we are at the target voltage yet"
      # "in this part we calculate incriment for Vg"
      n225 = flat-sequence {
        tunnel: w419 -> [w1623]
        tunnel: [w1623] -> w417
        tunnel: [w1625] -> w418
        tunnel: w417 -> [w1625]
        tunnel: [w1624] -> w416
        frame #0 {
          n226 = property on="Time btw \npoints, sec" class="DigNum (strict)"(error in=w1623) -> ("Value"=w1622:dbl)  [unwired: 1 in, 2 out]
          n227 = Multiply(x=w1622, y=1000) -> (x*y=w1620:dbl)
          n228 = To Long Integer(number=w1620) -> (32bit integer=w1619:i32)
          n229 = Wait Until Next ms Multiple(millisecond multiple=w1619) -> ()  [unwired: 1 out]
        }
        frame #1 {
          n230 = Tick Count (ms)() -> (millisecond timer value=w1624:u32)
        }
      }
      n231 = Build Array (concatenate)(w432, w431) -> (w430:dbl[])
      n232 = property on="array for data" class="Arr (strict)"(error in=w418, "Value"=w430) -> (error out=w429:errorcluster)  [unwired: 1 in, 1 out]
      n233 = case shown="False" "Commutator" {
        tunnel: [w473 w1253] -> w447
        tunnel: w429 -> [w474 w1252]
        frame True {
          n234 = stacked-sequence {
            tunnel: w474 -> [w491 w880]
            tunnel: [_ w865] -> w473
            frame #0 {
              n235 = stacked-sequence {
                tunnel: w491 -> [w495 _ _ _ _ _ _ _ _ _ _ _ _ _ _ _ _ _ _ _ _ _ _ _ _ _]
                tunnel: [w495 _ _ _ _ _ _ _ _ _ _ _ _ _ _ _ _ _ _ _ _ _ _ _ _ _] -> w475
                frame #0 {
                  # "check if oscillator on \nlock-in (address 1)\nis to be measured"
                  n236 = property on="Current is:" class="RadioBtnsControl (strict)"() -> ("Value"=w498:T1)  [unwired: 2 in, 2 out]
                  n237 = property on="array for data" class="Arr (strict)"() -> ("Value"=w497:dbl[])  [unwired: 2 in, 2 out]
                  n238 = Equal?(x=w498, y=1) -> (x = y?=w499:bool)
                  n239 = case shown="False" w499 {
                    tunnel: w497 -> [w501 w509]
                    tunnel: [w501 w508] -> w496
                    frame False {
                      # "we are not measuring oscillator from\nlock-in (address 1)"
                    }
                    frame True {
                      w505 = "1"
                      # "we are  measuring oscillator"
                      n240 = GPIB Write(0:w505, 1:"SLVL?") -> (6:w506:errorcluster)  [unwired: 3 in, 1 out]
                      n241 = GPIB Read(0:w505, 1:3200, 3:w506) -> (5:w503:string)  [unwired: 2 in, 2 out]
                      n242 = Fract/Exp String To Number(string=w503) -> (number=w502:dbl)  [unwired: 3 in, 1 out]
                      n243 = Build Array (concatenate)(w509, w502) -> (w508:dbl[])
                    }
                  }
                  n244 = property on="array for data" class="Arr (strict)"("Value"=w496) -> ()  [unwired: 2 in, 2 out]
                }
                frame #1 {
                  # "check if in-phase\nsignal on lock-in \n(address 1) is to\nbe measured"
                  n245 = property on="array for data" class="Arr (strict)"() -> ("Value"=w512:dbl[])  [unwired: 2 in, 2 out]
                  n246 = property on="Addr 1 lock-in" class="Bool (strict)"() -> ("Value"=w510:bool)  [unwired: 2 in, 2 out]
                  n247 = case shown="False" w510 {
                    tunnel: w512 -> [w513 w521]
                    tunnel: [w513 w520] -> w511
                    frame False {
                      # "we are not measuring in phase signal on lock-in (address 1)"
                    }
                    frame True {
                      w518 = "1"
                      # "we are  measuring lock-in (address 1), in phase"
                      n248 = GPIB Write(0:w518, 1:"OUTP?1") -> (6:w519:errorcluster)  [unwired: 3 in, 1 out]
                      n249 = GPIB Read(0:w518, 1:3200, 3:w519) -> (5:w516:string)  [unwired: 2 in, 2 out]
                      n250 = Fract/Exp String To Number(string=w516) -> (number=w515:dbl)  [unwired: 3 in, 1 out]
                      n251 = Build Array (concatenate)(w521, w515) -> (w520:dbl[])
                    }
                  }
                  n252 = property on="array for data" class="Arr (strict)"("Value"=w511) -> ()  [unwired: 2 in, 2 out]
                }
                frame #2 {
                  # "check if out-of-phase\nsignal on lock-in \n(address 1) is to\nbe measured"
                  n253 = property on="Addr 1 lock-in oop" class="Bool (strict)"() -> ("Value"=w522:bool)  [unwired: 2 in, 2 out]
                  n254 = property on="array for data" class="Arr (strict)"() -> ("Value"=w524:dbl[])  [unwired: 2 in, 2 out]
                  n255 = case shown="False" w522 {
                    tunnel: w524 -> [w525 w533]
                    tunnel: [w525 w532] -> w523
                    frame False {
                      # "we are not measuring out-of-phase signal on lock-in (address 1)"
                    }
                    frame True {
                      w530 = "1"
                      # "we are  measuring lock-in (address 1), out-of-phase signal"
                      n256 = GPIB Write(0:w530, 1:"OUTP?2") -> (6:w531:errorcluster)  [unwired: 3 in, 1 out]
                      n257 = GPIB Read(0:w530, 1:3200, 3:w531) -> (5:w528:string)  [unwired: 2 in, 2 out]
                      n258 = Fract/Exp String To Number(string=w528) -> (number=w527:dbl)  [unwired: 3 in, 1 out]
                      n259 = Build Array (concatenate)(w533, w527) -> (w532:dbl[])
                    }
                  }
                  n260 = property on="array for data" class="Arr (strict)"("Value"=w523) -> ()  [unwired: 2 in, 2 out]
                }
                frame #3 {
                  # "check if in-phase\nsignal on lock-in \n(address 2) is to\nbe measured"
                  n261 = property on="Addr 2 lock-in" class="Bool (strict)"() -> ("Value"=w534:bool)  [unwired: 2 in, 2 out]
                  n262 = property on="array for data" class="Arr (strict)"() -> ("Value"=w536:dbl[])  [unwired: 2 in, 2 out]
                  n263 = case shown="False" w534 {
                    tunnel: w536 -> [w537 w545]
                    tunnel: [w537 w544] -> w535
                    frame False {
                      # "we are not measuring in phase signal on lock-in (address 2)"
                    }
                    frame True {
                      w542 = "2"
                      # "we are  measuring lock-in (address 2), in phase"
                      n264 = GPIB Write(0:w542, 1:"OUTP?1") -> (6:w543:errorcluster)  [unwired: 3 in, 1 out]
                      n265 = GPIB Read(0:w542, 1:3200, 3:w543) -> (5:w540:string)  [unwired: 2 in, 2 out]
                      n266 = Fract/Exp String To Number(string=w540) -> (number=w539:dbl)  [unwired: 3 in, 1 out]
                      n267 = Build Array (concatenate)(w545, w539) -> (w544:dbl[])
                    }
                  }
                  n268 = property on="array for data" class="Arr (strict)"("Value"=w535) -> ()  [unwired: 2 in, 2 out]
                }
                frame #4 {
                  # "check if out-of-phase\nsignal on lock-in \n(address 2) is to\nbe measured"
                  n269 = property on="Addr 2 lock-in oop" class="Bool (strict)"() -> ("Value"=w546:bool)  [unwired: 2 in, 2 out]
                  n270 = property on="array for data" class="Arr (strict)"() -> ("Value"=w548:dbl[])  [unwired: 2 in, 2 out]
                  n271 = case shown="False" w546 {
                    tunnel: w548 -> [w549 w557]
                    tunnel: [w549 w556] -> w547
                    tunnel: w546 -> [_ _]
                    frame False {
                      # "we are not measuring out-of-phase signal on lock-in (address 2)"
                    }
                    frame True {
                      w554 = "2"
                      # "we are  measuring lock-in (address 2), out-of-phase"
                      n272 = GPIB Write(0:w554, 1:"OUTP?2") -> (6:w555:errorcluster)  [unwired: 3 in, 1 out]
                      n273 = GPIB Read(0:w554, 1:3200, 3:w555) -> (5:w552:string)  [unwired: 2 in, 2 out]
                      n274 = Fract/Exp String To Number(string=w552) -> (number=w551:dbl)  [unwired: 3 in, 1 out]
                      n275 = Build Array (concatenate)(w557, w551) -> (w556:dbl[])
                    }
                  }
                  n276 = property on="array for data" class="Arr (strict)"("Value"=w547) -> ()  [unwired: 2 in, 2 out]
                }
                frame #5 {
                  # "check if in-phase\nsignal on lock-in \n(address 3) is to\nbe measured"
                  n277 = property on="Addr 3 lock-in" class="Bool (strict)"() -> ("Value"=w558:bool)  [unwired: 2 in, 2 out]
                  n278 = property on="array for data" class="Arr (strict)"() -> ("Value"=w560:dbl[])  [unwired: 2 in, 2 out]
                  n279 = case shown="False" w558 {
                    tunnel: w560 -> [w561 w569]
                    tunnel: [w561 w568] -> w559
                    frame False {
                      # "we are not measuring in phase signal on lock-in (address 3)"
                    }
                    frame True {
                      w566 = "3"
                      # "we are  measuring lock-in (address 3), in phase"
                      n280 = GPIB Write(0:w566, 1:"OUTP?1") -> (6:w567:errorcluster)  [unwired: 3 in, 1 out]
                      n281 = GPIB Read(0:w566, 1:3200, 3:w567) -> (5:w564:string)  [unwired: 2 in, 2 out]
                      n282 = Fract/Exp String To Number(string=w564) -> (number=w563:dbl)  [unwired: 3 in, 1 out]
                      n283 = Build Array (concatenate)(w569, w563) -> (w568:dbl[])
                    }
                  }
                  n284 = property on="array for data" class="Arr (strict)"("Value"=w559) -> ()  [unwired: 2 in, 2 out]
                }
                frame #6 {
                  # "check if out-of-phase\nsignal on lock-in \n(address 3) is to\nbe measured"
                  n285 = property on="Addr 3 lock-in oop" class="Bool (strict)"() -> ("Value"=w570:bool)  [unwired: 2 in, 2 out]
                  n286 = property on="array for data" class="Arr (strict)"() -> ("Value"=w572:dbl[])  [unwired: 2 in, 2 out]
                  n287 = case shown="False" w570 {
                    tunnel: w572 -> [w573 w581]
                    tunnel: [w573 w580] -> w571
                    frame False {
                      # "we are not measuring out-of-phase signal on lock-in (address 3)"
                    }
                    frame True {
                      w578 = "3"
                      # "we are  measuring lock-in (address 3), out-of-phase"
                      n288 = GPIB Write(0:w578, 1:"OUTP?2") -> (6:w579:errorcluster)  [unwired: 3 in, 1 out]
                      n289 = GPIB Read(0:w578, 1:3200, 3:w579) -> (5:w576:string)  [unwired: 2 in, 2 out]
                      n290 = Fract/Exp String To Number(string=w576) -> (number=w575:dbl)  [unwired: 3 in, 1 out]
                      n291 = Build Array (concatenate)(w581, w575) -> (w580:dbl[])
                    }
                  }
                  n292 = property on="array for data" class="Arr (strict)"("Value"=w571) -> ()  [unwired: 2 in, 2 out]
                }
                frame #7 {
                  # "check if in-phase\nsignal on lock-in \n(address 4) is to\nbe measured"
                  n293 = property on="Addr 4 lock-in" class="Bool (strict)"() -> ("Value"=w582:bool)  [unwired: 2 in, 2 out]
                  n294 = property on="array for data" class="Arr (strict)"() -> ("Value"=w584:dbl[])  [unwired: 2 in, 2 out]
                  n295 = case shown="False" w582 {
                    tunnel: w584 -> [w585 w593]
                    tunnel: [w585 w592] -> w583
                    frame False {
                      # "we are not measuring in phase signal on lock-in (address 4)"
                    }
                    frame True {
                      w590 = "4"
                      # "we are  measuring lock-in (address 4), in phase"
                      n296 = GPIB Write(0:w590, 1:"OUTP?1") -> (6:w591:errorcluster)  [unwired: 3 in, 1 out]
                      n297 = GPIB Read(0:w590, 1:3200, 3:w591) -> (5:w588:string)  [unwired: 2 in, 2 out]
                      n298 = Fract/Exp String To Number(string=w588) -> (number=w587:dbl)  [unwired: 3 in, 1 out]
                      n299 = Build Array (concatenate)(w593, w587) -> (w592:dbl[])
                    }
                  }
                  n300 = property on="array for data" class="Arr (strict)"("Value"=w583) -> ()  [unwired: 2 in, 2 out]
                }
                frame #8 {
                  # "check if out-of-phase\nsignal on lock-in \n(address 4) is to\nbe measured"
                  n301 = property on="Addr 4 lock-in oop" class="Bool (strict)"() -> ("Value"=w594:bool)  [unwired: 2 in, 2 out]
                  n302 = property on="array for data" class="Arr (strict)"() -> ("Value"=w596:dbl[])  [unwired: 2 in, 2 out]
                  n303 = case shown="False" w594 {
                    tunnel: w596 -> [w597 w605]
                    tunnel: [w597 w604] -> w595
                    frame False {
                      # "we are not measuring out-of-phase signal on lock-in (address 4)"
                    }
                    frame True {
                      w602 = "4"
                      # "we are  measuring lock-in (address 4), out-of-phase"
                      n304 = GPIB Write(0:w602, 1:"OUTP?2") -> (6:w603:errorcluster)  [unwired: 3 in, 1 out]
                      n305 = GPIB Read(0:w602, 1:3200, 3:w603) -> (5:w600:string)  [unwired: 2 in, 2 out]
                      n306 = Fract/Exp String To Number(string=w600) -> (number=w599:dbl)  [unwired: 3 in, 1 out]
                      n307 = Build Array (concatenate)(w605, w599) -> (w604:dbl[])
                    }
                  }
                  n308 = property on="array for data" class="Arr (strict)"("Value"=w595) -> ()  [unwired: 2 in, 2 out]
                }
                frame #9 {
                  # "check if in-phase\nsignal on lock-in \n(address 5) is to\nbe measured"
                  n309 = property on="Addr 5 lock-in" class="Bool (strict)"() -> ("Value"=w606:bool)  [unwired: 2 in, 2 out]
                  n310 = property on="array for data" class="Arr (strict)"() -> ("Value"=w608:dbl[])  [unwired: 2 in, 2 out]
                  n311 = case shown="False" w606 {
                    tunnel: w608 -> [w609 w617]
                    tunnel: [w609 w616] -> w607
                    frame False {
                      # "we are not measuring in phase signal on lock-in (address 5)"
                    }
                    frame True {
                      w614 = "5"
                      # "we are  measuring lock-in (address 5), in phase"
                      n312 = GPIB Write(0:w614, 1:"OUTP?1") -> (6:w615:errorcluster)  [unwired: 3 in, 1 out]
                      n313 = GPIB Read(0:w614, 1:3200, 3:w615) -> (5:w612:string)  [unwired: 2 in, 2 out]
                      n314 = Fract/Exp String To Number(string=w612) -> (number=w611:dbl)  [unwired: 3 in, 1 out]
                      n315 = Build Array (concatenate)(w617, w611) -> (w616:dbl[])
                    }
                  }
                  n316 = property on="array for data" class="Arr (strict)"("Value"=w607) -> ()  [unwired: 2 in, 2 out]
                }
                frame #10 {
                  # "check if out-of-phase\nsignal on lock-in \n(address 5) is to\nbe measured"
                  n317 = property on="Addr 5 lock-in oop" class="Bool (strict)"() -> ("Value"=w618:bool)  [unwired: 2 in, 2 out]
                  n318 = property on="array for data" class="Arr (strict)"() -> ("Value"=w620:dbl[])  [unwired: 2 in, 2 out]
                  n319 = case shown="False" w618 {
                    tunnel: w620 -> [w621 w629]
                    tunnel: [w621 w628] -> w619
                    frame False {
                      # "we are not measuring out-of-phase signal on lock-in (address 5)"
                    }
                    frame True {
                      w626 = "5"
                      # "we are  measuring lock-in (address 5), out-of-phase"
                      n320 = GPIB Write(0:w626, 1:"OUTP?2") -> (6:w627:errorcluster)  [unwired: 3 in, 1 out]
                      n321 = GPIB Read(0:w626, 1:3200, 3:w627) -> (5:w624:string)  [unwired: 2 in, 2 out]
                      n322 = Fract/Exp String To Number(string=w624) -> (number=w623:dbl)  [unwired: 3 in, 1 out]
                      n323 = Build Array (concatenate)(w629, w623) -> (w628:dbl[])
                    }
                  }
                  n324 = property on="array for data" class="Arr (strict)"("Value"=w619) -> ()  [unwired: 2 in, 2 out]
                }
                frame #11 {
                  # "check if voltage on \nmain Keithley 2400 \n(addr. 12) is to\nbe measured"
                  n325 = property on="Voltage (Vk1)" class="Bool (strict)"() -> ("Value"=w630:bool)  [unwired: 2 in, 2 out]
                  n326 = property on="array for data" class="Arr (strict)"() -> ("Value"=w632:dbl[])  [unwired: 2 in, 2 out]
                  n327 = case shown="False" w630 {
                    tunnel: w632 -> [w633 w643]
                    tunnel: [w633 w642] -> w631
                    frame False {
                      # "we aren't measuring voltage \non main Keithley 2400 (addr. 12)"
                    }
                    frame True {
                      w640 = "12"
                      # "we are measuring voltage \non main Keithley 2400 (addr. 12)"
                      n328 = GPIB Write(0:w640, 1:":READ?") -> (6:w641:errorcluster)  [unwired: 3 in, 1 out]
                      n329 = GPIB Read(0:w640, 1:3200, 3:w641) -> (5:w636:string)  [unwired: 2 in, 2 out]
                      n330 = String Subset(string=w636, length (rest)=13) -> (substring=w635:string)  [unwired: 1 in]
                      n331 = Fract/Exp String To Number(string=w635) -> (number=w638:dbl)  [unwired: 3 in, 1 out]
                      n332 = Build Array (concatenate)(w643, w638) -> (w642:dbl[])
                    }
                  }
                  n333 = property on="array for data" class="Arr (strict)"("Value"=w631) -> ()  [unwired: 2 in, 2 out]
                }
                frame #12 {
                  # "check if  current on \nmain Keithley 2400 \n(addr. 12) is to\nbe measured"
                  n334 = property on="Current (Ik1)" class="Bool (strict)"() -> ("Value"=w644:bool)  [unwired: 2 in, 2 out]
                  n335 = property on="array for data" class="Arr (strict)"() -> ("Value"=w646:dbl[])  [unwired: 2 in, 2 out]
                  n336 = case shown="True" w644 {
                    tunnel: w646 -> [w647 w658]
                    tunnel: [w647 w657] -> w645
                    frame False {
                      # "we aren't measuring current \non main Keithley 2400 (addr. 12)"
                    }
                    frame True {
                      w655 = "12"
                      # "we are measuring current\non main Keithley 2400 (addr. 12)"
                      n337 = GPIB Write(0:w655, 1:":READ?") -> (6:w656:errorcluster)  [unwired: 3 in, 1 out]
                      n338 = GPIB Read(0:w655, 1:3200, 3:w656) -> (5:w651:string)  [unwired: 2 in, 2 out]
                      n339 = String Subset(string=w651, offset (0)=14, length (rest)=13) -> (substring=w650:string)
                      n340 = Fract/Exp String To Number(string=w650) -> (number=w653:dbl)  [unwired: 3 in, 1 out]
                      n341 = Build Array (concatenate)(w658, w653) -> (w657:dbl[])
                    }
                  }
                  n342 = property on="array for data" class="Arr (strict)"("Value"=w645) -> ()  [unwired: 2 in, 2 out]
                }
                frame #13 {
                  # "check if voltage on \nadd. Keithley 2400 \n(addr. 13) is to\nbe measured"
                  n343 = property on="Voltage (Vk2)" class="Bool (strict)"() -> ("Value"=w659:bool)  [unwired: 2 in, 2 out]
                  n344 = property on="array for data" class="Arr (strict)"() -> ("Value"=w661:dbl[])  [unwired: 2 in, 2 out]
                  n345 = case shown="True" w659 {
                    tunnel: w661 -> [w662 w672]
                    tunnel: [w662 w671] -> w660
                    frame False {
                      # "we aren't measuring voltage \non additional Keithley 2400 (addr. 13)"
                    }
                    frame True {
                      w669 = "13"
                      # "we are measuring voltage \non additional Keithley 2400 (addr. 13)"
                      n346 = GPIB Write(0:w669, 1:":READ?") -> (6:w670:errorcluster)  [unwired: 3 in, 1 out]
                      n347 = GPIB Read(0:w669, 1:3200, 3:w670) -> (5:w665:string)  [unwired: 2 in, 2 out]
                      n348 = String Subset(string=w665, length (rest)=13) -> (substring=w664:string)  [unwired: 1 in]
                      n349 = Fract/Exp String To Number(string=w664) -> (number=w667:dbl)  [unwired: 3 in, 1 out]
                      n350 = Build Array (concatenate)(w672, w667) -> (w671:dbl[])
                    }
                  }
                  n351 = property on="array for data" class="Arr (strict)"("Value"=w660) -> ()  [unwired: 2 in, 2 out]
                }
                frame #14 {
                  # "check if  current on \nadd. Keithley 2400 \n(addr. 13) is to\nbe measured"
                  n352 = property on="Current (Ik2)" class="Bool (strict)"() -> ("Value"=w673:bool)  [unwired: 2 in, 2 out]
                  n353 = property on="array for data" class="Arr (strict)"() -> ("Value"=w675:dbl[])  [unwired: 2 in, 2 out]
                  n354 = case shown="True" w673 {
                    tunnel: w675 -> [w676 w687]
                    tunnel: [w676 w686] -> w674
                    frame False {
                      # "we aren't measuring current \non additional Keithley 2400 (addr. 13)"
                    }
                    frame True {
                      w684 = "13"
                      # "we are measuring current\non additional Keithley 2400 (addr. 13)"
                      n355 = GPIB Write(0:w684, 1:":READ?") -> (6:w685:errorcluster)  [unwired: 3 in, 1 out]
                      n356 = GPIB Read(0:w684, 1:3200, 3:w685) -> (5:w680:string)  [unwired: 2 in, 2 out]
                      n357 = String Subset(string=w680, offset (0)=14, length (rest)=13) -> (substring=w679:string)
                      n358 = Fract/Exp String To Number(string=w679) -> (number=w682:dbl)  [unwired: 3 in, 1 out]
                      n359 = Build Array (concatenate)(w687, w682) -> (w686:dbl[])
                    }
                  }
                  n360 = property on="array for data" class="Arr (strict)"("Value"=w674) -> ()  [unwired: 2 in, 2 out]
                }
                frame #15 {
                  # "check if voltage on \nadd. Keithley 2400 \n(addr. 14) is to\nbe measured"
                  n361 = property on="Voltage (Vk3)" class="Bool (strict)"() -> ("Value"=w688:bool)  [unwired: 2 in, 2 out]
                  n362 = property on="array for data" class="Arr (strict)"() -> ("Value"=w690:dbl[])  [unwired: 2 in, 2 out]
                  n363 = case shown="True" w688 {
                    tunnel: w690 -> [w691 w701]
                    tunnel: [w691 w700] -> w689
                    frame False {
                      # "we aren't measuring voltage \non additional Keithley 2400 (addr. 14)"
                    }
                    frame True {
                      w698 = "14"
                      # "we are measuring voltage \non additional Keithley 2400 (addr. 14)"
                      n364 = GPIB Write(0:w698, 1:":READ?") -> (6:w699:errorcluster)  [unwired: 3 in, 1 out]
                      n365 = GPIB Read(0:w698, 1:3200, 3:w699) -> (5:w694:string)  [unwired: 2 in, 2 out]
                      n366 = String Subset(string=w694, length (rest)=13) -> (substring=w693:string)  [unwired: 1 in]
                      n367 = Fract/Exp String To Number(string=w693) -> (number=w696:dbl)  [unwired: 3 in, 1 out]
                      n368 = Build Array (concatenate)(w701, w696) -> (w700:dbl[])
                    }
                  }
                  n369 = property on="array for data" class="Arr (strict)"("Value"=w689) -> ()  [unwired: 2 in, 2 out]
                }
                frame #16 {
                  # "check if  current on \nadd. Keithley 2400 \n(addr. 14) is to\nbe measured"
                  n370 = property on="Current (Ik3)" class="Bool (strict)"() -> ("Value"=w702:bool)  [unwired: 2 in, 2 out]
                  n371 = property on="array for data" class="Arr (strict)"() -> ("Value"=w704:dbl[])  [unwired: 2 in, 2 out]
                  n372 = case shown="True" w702 {
                    tunnel: w704 -> [w705 w716]
                    tunnel: [w705 w715] -> w703
                    frame False {
                      # "we aren't measuring current \non additional Keithley 2400 (addr. 14)"
                    }
                    frame True {
                      w713 = "14"
                      # "we are measuring current\non additional Keithley 2400 (addr. 14)"
                      n373 = GPIB Write(0:w713, 1:":READ?") -> (6:w714:errorcluster)  [unwired: 3 in, 1 out]
                      n374 = GPIB Read(0:w713, 1:3200, 3:w714) -> (5:w709:string)  [unwired: 2 in, 2 out]
                      n375 = String Subset(string=w709, offset (0)=14, length (rest)=13) -> (substring=w708:string)
                      n376 = Fract/Exp String To Number(string=w708) -> (number=w711:dbl)  [unwired: 3 in, 1 out]
                      n377 = Build Array (concatenate)(w716, w711) -> (w715:dbl[])
                    }
                  }
                  n378 = property on="array for data" class="Arr (strict)"("Value"=w703) -> ()  [unwired: 2 in, 2 out]
                }
                frame #17 {
                  # "check if 1st channel\non Keithley 2182 \n(addr. 15) is to\nbe measured"
                  n379 = property on="Channel 1 (Vnano1)" class="Bool (strict)"() -> ("Value"=w717:bool)  [unwired: 2 in, 2 out]
                  n380 = property on="array for data" class="Arr (strict)"() -> ("Value"=w719:dbl[])  [unwired: 2 in, 2 out]
                  n381 = case shown="True" w717 {
                    tunnel: w719 -> [w720 w728]
                    tunnel: [w720 w727] -> w718
                    frame False {
                      # "we are not measuring 1st channel\non Keithley 2182 (addr. 15)"
                    }
                    frame True {
                      w725 = "15"
                      # "we are measuring 1st channel\non Keithley 2182 (addr. 15)"
                      n382 = GPIB Write(0:w725, 1:":SENSe:DATA:FRES?") -> (6:w726:errorcluster)  [unwired: 3 in, 1 out]
                      n383 = GPIB Read(0:w725, 1:200, 3:w726) -> (5:w721:string)  [unwired: 2 in, 2 out]
                      n384 = Fract/Exp String To Number(string=w721) -> (number=w723:dbl)  [unwired: 3 in, 1 out]
                      n385 = Build Array (concatenate)(w728, w723) -> (w727:dbl[])
                    }
                  }
                  n386 = property on="array for data" class="Arr (strict)"("Value"=w718) -> ()  [unwired: 2 in, 2 out]
                }
                frame #18 {
                  # "check if 2nd channel\non Keithley 2182 \n(addr. 15) is to\nbe measured"
                  n387 = property on="Channel 2 (Vnano1b)" class="Bool (strict)"() -> ("Value"=w729:bool)  [unwired: 2 in, 2 out]
                  n388 = property on="array for data" class="Arr (strict)"() -> ("Value"=w731:dbl[])  [unwired: 2 in, 2 out]
                  n389 = case shown="False" w729 {
                    tunnel: w731 -> [w732 w744]
                    tunnel: [w732 w743] -> w730
                    frame False {
                      # "we are not measuring 1st channel\non Keithley 2182 (addr. 15)"
                    }
                    frame True {
                      w735 = "15"
                      # "switching to channel 2 and then\nback to channel 1"
                      # "we are measuring 2nd channel\non Keithley 2182 (addr. 15)"
                      n390 = GPIB Write(0:w735, 1:":SENSe:CHAN 2") -> (6:w736:errorcluster)  [unwired: 3 in, 1 out]
                      n391 = GPIB Write(0:w735, 1:":SENSe:DATA:FRES?", 3:w736) -> (6:w742:errorcluster)  [unwired: 2 in, 1 out]
                      n392 = GPIB Read(0:w735, 1:200, 3:w742) -> (5:w738:string, 7:w734:errorcluster)  [unwired: 2 in, 1 out]
                      n393 = GPIB Write(0:w735, 1:":SENSe:CHAN 1", 3:w734) -> ()  [unwired: 2 in, 2 out]
                      n394 = Fract/Exp String To Number(string=w738) -> (number=w740:dbl)  [unwired: 3 in, 1 out]
                      n395 = Build Array (concatenate)(w744, w740) -> (w743:dbl[])
                    }
                  }
                  n396 = property on="array for data" class="Arr (strict)"("Value"=w730) -> ()  [unwired: 2 in, 2 out]
                }
                frame #19 {
                  # "check if 1st channel\non Keithley 2182 \n(addr. 16) is to\nbe measured"
                  n397 = property on="Channel 1 (Vnano2)" class="Bool (strict)"() -> ("Value"=w745:bool)  [unwired: 2 in, 2 out]
                  n398 = property on="array for data" class="Arr (strict)"() -> ("Value"=w747:dbl[])  [unwired: 2 in, 2 out]
                  n399 = case shown="True" w745 {
                    tunnel: w747 -> [w748 w756]
                    tunnel: [w748 w755] -> w746
                    frame False {
                      # "we are not measuring 1st channel\non Keithley 2182 (addr. 16)"
                    }
                    frame True {
                      w753 = "16"
                      # "we are measuring 1st channel\non Keithley 2182 (addr. 16)"
                      n400 = GPIB Write(0:w753, 1:":SENSe:DATA:FRES?") -> (6:w754:errorcluster)  [unwired: 3 in, 1 out]
                      n401 = GPIB Read(0:w753, 1:200, 3:w754) -> (5:w749:string)  [unwired: 2 in, 2 out]
                      n402 = Fract/Exp String To Number(string=w749) -> (number=w751:dbl)  [unwired: 3 in, 1 out]
                      n403 = Build Array (concatenate)(w756, w751) -> (w755:dbl[])
                    }
                  }
                  n404 = property on="array for data" class="Arr (strict)"("Value"=w746) -> ()  [unwired: 2 in, 2 out]
                }
                frame #20 {
                  # "check if 2nd channel\non Keithley 2182 \n(addr. 16) is to\nbe measured"
                  n405 = property on="Channel 2 (Vnano2b)" class="Bool (strict)"() -> ("Value"=w757:bool)  [unwired: 2 in, 2 out]
                  n406 = property on="array for data" class="Arr (strict)"() -> ("Value"=w759:dbl[])  [unwired: 2 in, 2 out]
                  n407 = case shown="False" w757 {
                    tunnel: w759 -> [w760 w772]
                    tunnel: [w760 w771] -> w758
                    frame False {
                      # "we are not measuring 1st channel\non Keithley 2182 (addr. 16)"
                    }
                    frame True {
                      w763 = "16"
                      # "switching to channel 2 and then\nback to channel 1"
                      # "we are measuring 2nd channel\non Keithley 2182 (addr. 16)"
                      n408 = GPIB Write(0:w763, 1:":SENSe:CHAN 2") -> (6:w764:errorcluster)  [unwired: 3 in, 1 out]
                      n409 = GPIB Write(0:w763, 1:":SENSe:DATA:FRES?", 3:w764) -> (6:w770:errorcluster)  [unwired: 2 in, 1 out]
                      n410 = GPIB Read(0:w763, 1:200, 3:w770) -> (5:w766:string, 7:w762:errorcluster)  [unwired: 2 in, 1 out]
                      n411 = GPIB Write(0:w763, 1:":SENSe:CHAN 1", 3:w762) -> ()  [unwired: 2 in, 2 out]
                      n412 = Fract/Exp String To Number(string=w766) -> (number=w768:dbl)  [unwired: 3 in, 1 out]
                      n413 = Build Array (concatenate)(w772, w768) -> (w771:dbl[])
                    }
                  }
                  n414 = property on="array for data" class="Arr (strict)"("Value"=w758) -> ()  [unwired: 2 in, 2 out]
                }
                frame #21 {
                  # "check if 1st channel\non Keithley 2182 \n(addr. 17) is to\nbe measured"
                  n415 = property on="Channel 1 (Vnano3)" class="Bool (strict)"() -> ("Value"=w773:bool)  [unwired: 2 in, 2 out]
                  n416 = property on="array for data" class="Arr (strict)"() -> ("Value"=w775:dbl[])  [unwired: 2 in, 2 out]
                  n417 = case shown="True" w773 {
                    tunnel: w775 -> [w776 w784]
                    tunnel: [w776 w783] -> w774
                    frame False {
                      # "we are not measuring 1st channel\non Keithley 2182 (addr. 17)"
                    }
                    frame True {
                      w781 = "17"
                      # "we are measuring 1st channel\non Keithley 2182 (addr. 17)"
                      n418 = GPIB Write(0:w781, 1:":SENSe:DATA:FRES?") -> (6:w782:errorcluster)  [unwired: 3 in, 1 out]
                      n419 = GPIB Read(0:w781, 1:200, 3:w782) -> (5:w777:string)  [unwired: 2 in, 2 out]
                      n420 = Fract/Exp String To Number(string=w777) -> (number=w779:dbl)  [unwired: 3 in, 1 out]
                      n421 = Build Array (concatenate)(w784, w779) -> (w783:dbl[])
                    }
                  }
                  n422 = property on="array for data" class="Arr (strict)"("Value"=w774) -> ()  [unwired: 2 in, 2 out]
                }
                frame #22 {
                  # "check if 2nd channel\non Keithley 2182 \n(addr. 17) is to\nbe measured"
                  n423 = property on="Channel 2 (Vnano3b)" class="Bool (strict)"() -> ("Value"=w785:bool)  [unwired: 2 in, 2 out]
                  n424 = property on="array for data" class="Arr (strict)"() -> ("Value"=w787:dbl[])  [unwired: 2 in, 2 out]
                  n425 = case shown="False" w785 {
                    tunnel: w787 -> [w788 w800]
                    tunnel: [w788 w799] -> w786
                    frame False {
                      # "we are not measuring 1st channel\non Keithley 2182 (addr. 17)"
                    }
                    frame True {
                      w791 = "17"
                      # "switching to channel 2 and then\nback to channel 1"
                      # "we are measuring 2nd channel\non Keithley 2182 (addr. 17)"
                      n426 = GPIB Write(0:w791, 1:":SENSe:CHAN 2") -> (6:w792:errorcluster)  [unwired: 3 in, 1 out]
                      n427 = GPIB Write(0:w791, 1:":SENSe:DATA:FRES?", 3:w792) -> (6:w798:errorcluster)  [unwired: 2 in, 1 out]
                      n428 = GPIB Read(0:w791, 1:200, 3:w798) -> (5:w794:string, 7:w790:errorcluster)  [unwired: 2 in, 1 out]
                      n429 = GPIB Write(0:w791, 1:":SENSe:CHAN 1", 3:w790) -> ()  [unwired: 2 in, 2 out]
                      n430 = Fract/Exp String To Number(string=w794) -> (number=w796:dbl)  [unwired: 3 in, 1 out]
                      n431 = Build Array (concatenate)(w800, w796) -> (w799:dbl[])
                    }
                  }
                  n432 = property on="array for data" class="Arr (strict)"("Value"=w786) -> ()  [unwired: 2 in, 2 out]
                }
                frame #23 {
                  # "check if 1st \nthermometer on \nOxford ITC \n(address 24) \nis measured"
                  n433 = property on="Thermometer 1 (T1)" class="Bool (strict)"() -> ("Value"=w801:bool)  [unwired: 2 in, 2 out]
                  n434 = property on="array for data" class="Arr (strict)"() -> ("Value"=w803:dbl[])  [unwired: 2 in, 2 out]
                  n435 = case shown="True" w801 {
                    tunnel: w803 -> [w804 w813]
                    tunnel: [w804 w812] -> w802
                    frame False {
                      # "we are not measuring temperature on\nthermometer 1 (addr. 24)"
                    }
                    frame True {
                      w805 = 1
                      w810 = "24"
                      # "we are measuring temperature,\nthermometer 1 (addr. 24)"
                      n436 = GPIB Write(0:w810, 1:"R 1", 2:w805) -> (6:w811:errorcluster)  [unwired: 2 in, 1 out]
                      n437 = GPIB Read(0:w810, 1:200, 2:w805, 3:w811) -> (5:w806:string)  [unwired: 1 in, 2 out]
                      n438 = Fract/Exp String To Number(string=w806, offset=w805) -> (number=w808:dbl)  [unwired: 2 in, 1 out]
                      n439 = Build Array (concatenate)(w813, w808) -> (w812:dbl[])
                    }
                  }
                  n440 = property on="array for data" class="Arr (strict)"("Value"=w802) -> ()  [unwired: 2 in, 2 out]
                }
                frame #24 {
                  # "check if 1st \nthermometer on \nOxford ITC \n(address 24) \nis measured"
                  n441 = property on="Magnetic Field (B)" class="Bool (strict)"() -> ("Value"=w814:bool)  [unwired: 2 in, 2 out]
                  n442 = property on="array for data" class="Arr (strict)"() -> ("Value"=w816:dbl[])  [unwired: 2 in, 2 out]
                  n443 = case shown="True" w814 {
                    tunnel: w816 -> [w817 w826]
                    tunnel: [w817 w825] -> w815
                    frame False {
                      # "we are not measuringmagnetic field (addr. 25)"
                    }
                    frame True {
                      w818 = 1
                      w823 = "25"
                      # "we are measuring magnetic field  (addr. 25)"
                      n444 = GPIB Write(0:w823, 1:"R 7", 2:w818) -> (6:w824:errorcluster)  [unwired: 2 in, 1 out]
                      n445 = GPIB Read(0:w823, 1:200, 2:w818, 3:w824) -> (5:w819:string)  [unwired: 1 in, 2 out]
                      n446 = Fract/Exp String To Number(string=w819, offset=w818) -> (number=w821:dbl)  [unwired: 2 in, 1 out]
                      n447 = Build Array (concatenate)(w826, w821) -> (w825:dbl[])
                    }
                  }
                  n448 = property on="array for data" class="Arr (strict)"("Value"=w815) -> ()  [unwired: 2 in, 2 out]
                }
                frame #25 {
                  # "check if capacitance\nand loss (address 28)\nare measured"
                  n449 = property on="Capacitance (C) and Loss (L)" class="Bool (strict)"() -> ("Value"=w827:bool)  [unwired: 2 in, 2 out]
                  n450 = property on="array for data" class="Arr (strict)"() -> ("Value"=w829:dbl[])  [unwired: 2 in, 2 out]
                  n451 = case shown="False" w827 {
                    tunnel: w829 -> [w830 w836]
                    tunnel: [w830 w832] -> w828
                    frame False {
                      # "we are not measuringmagnetic capacitance (addr. 28)"
                    }
                    frame True {
                      # "we are measuring capacitance and loss  (addr. 28)"
                      n452 = stacked-sequence {
                        seq-local: [w838 _ _] -> [_ _ w861]
                        tunnel: [_ _ w855] -> w831
                        tunnel: [_ _ w856] -> w834
                        tunnel: "28" ("data") -> [w837 w841 w850]
                        frame #0 {
                          n453 = GPIB Write(0:w837, 1:"SINGLE" ("data"), 2:i16 0 ("mode (0)")) -> (6:w838:errorcluster)  [unwired: 2 in, 1 out]
                        }
                        frame #1 {
                          n454 = while {
                            tunnel: w841 -> [w842]
                            i -> [w843]
                            stop <- w845 continue-if-true
                            n455 = GPIB Serial Poll(0:w842) -> (2:w847:i16)  [unwired: 1 in, 2 out]
                            n456 = Less?(x=w847, y=i16 128) -> (x < y?=w845:bool)
                            n457 = Wait (ms)(milliseconds to wait=u32 50) -> ()  [unwired: 1 out]
                            "Numeric" <- w843
                          }
                        }
                        frame #2 {
                          w848 = i16 2 ("mode (0)")
                          n458 = GPIB Read(0:w850, 1:200 ("byte count"), 2:i16 2 ("mode (0)"), 3:w861) -> (5:w854:string)  [unwired: 1 in, 2 out]
                          n459 = Match Pattern(string=w854, regular expression="C=") -> (after substring=w853:string)  [unwired: 1 in, 3 out]
                          n460 = Match Pattern(string=w853, regular expression="PF L=") -> (after substring=w851:string)  [unwired: 1 in, 3 out]
                          n461 = Search/Split String(string=w853, search string/char (-)=" ", offset (0)=w848) -> (substring before match=w858:string)  [unwired: 2 out]
                          n462 = Search/Split String(string=w851, search string/char (-)=" ", offset (0)=w848) -> (substring before match=w857:string)  [unwired: 2 out]
                          n463 = Fract/Exp String To Number(string=w857) -> (number=w855:dbl)  [unwired: 3 in, 1 out]
                          n464 = Fract/Exp String To Number(string=w858) -> (number=w856:dbl)  [unwired: 3 in, 1 out]
                        }
                      }
                      n465 = Build Array (concatenate)(w836, w834) -> (w833:dbl[])
                      n466 = Build Array (concatenate)(w833, w831) -> (w832:dbl[])
                    }
                  }
                  n467 = property on="array for data" class="Arr (strict)"("Value"=w828) -> ()  [unwired: 2 in, 2 out]
                }
              }
              n468 = flat-sequence {
                tunnel: w476 -> [_]
                frame #0 {
                  n469 = property on="Delib Time delay" class="DigNum (strict)"() -> ("Value"=w492:i32)  [unwired: 2 in, 2 out]
                  n470 = Wait (ms)(milliseconds to wait=w492) -> ()  [unwired: 1 out]
                }
              }
              n471 = case shown="\"Radio Selection 2\"" "Commute SorceMeter" {
                tunnel: ["13" "14"] -> w477
                frame "Radio Selection 1", Default {
                }
                frame "Radio Selection 2" {
                }
              }
              n472 = GPIB Write(0:w477, 1:":READ?", 3:w475) -> (6:w478:errorcluster)  [unwired: 2 in, 1 out]
              n473 = GPIB Read(0:w477, 1:3200, 3:w478) -> (5:w481:string)  [unwired: 2 in, 2 out]
              n474 = String Subset(string=w481, length (rest)=13) -> (substring=w482:string)  [unwired: 1 in]
              n475 = Fract/Exp String To Number(string=w482) -> (number=w484:dbl)  [unwired: 3 in, 1 out]
              n476 = Multiply(x=w484, y=-1.0) -> (x*y=w489:dbl)
              n477 = Number To Fractional String(number=w489) -> (F-format string=w486:string)  [unwired: 3 in]
              n478 = Concatenate Strings(":INIT:IMM; :SOUR:VOLT:LEV:IMM:AMPL " ("data"), w486) -> (w487:string)
              n479 = GPIB Write(0:w477, 1:w487) -> (6:w476:errorcluster)  [unwired: 3 in, 1 out]
            }
            frame #1 {
              n480 = stacked-sequence {
                tunnel: w880 -> [w883 _ _ _ _ _ _ _ _ _ _ _ _ _ _ _ _ _ _ _ _ _ _ _ _ _]
                tunnel: [w883 _ _ _ _ _ _ _ _ _ _ _ _ _ _ _ _ _ _ _ _ _ _ _ _ _] -> w866
                frame #0 {
                  # "check if oscillator on \nlock-in (address 1)\nis to be measured"
                  n481 = property on="Current is:" class="RadioBtnsControl (strict)"() -> ("Value"=w886:T1)  [unwired: 2 in, 2 out]
                  n482 = property on="array for data" class="Arr (strict)"() -> ("Value"=w885:dbl[])  [unwired: 2 in, 2 out]
                  n483 = Equal?(x=w886, y=1) -> (x = y?=w887:bool)
                  n484 = case shown="False" w887 {
                    tunnel: w885 -> [w889 w897]
                    tunnel: [w889 w896] -> w884
                    frame False {
                      # "we are not measuring oscillator from\nlock-in (address 1)"
                    }
                    frame True {
                      w893 = "1"
                      # "we are  measuring oscillator"
                      n485 = GPIB Write(0:w893, 1:"SLVL?") -> (6:w894:errorcluster)  [unwired: 3 in, 1 out]
                      n486 = GPIB Read(0:w893, 1:3200, 3:w894) -> (5:w891:string)  [unwired: 2 in, 2 out]
                      n487 = Fract/Exp String To Number(string=w891) -> (number=w890:dbl)  [unwired: 3 in, 1 out]
                      n488 = Build Array (concatenate)(w897, w890) -> (w896:dbl[])
                    }
                  }
                  n489 = property on="array for data" class="Arr (strict)"("Value"=w884) -> ()  [unwired: 2 in, 2 out]
                }
                frame #1 {
                  # "check if in-phase\nsignal on lock-in \n(address 1) is to\nbe measured"
                  n490 = property on="array for data" class="Arr (strict)"() -> ("Value"=w900:dbl[])  [unwired: 2 in, 2 out]
                  n491 = property on="Addr 1 lock-in" class="Bool (strict)"() -> ("Value"=w898:bool)  [unwired: 2 in, 2 out]
                  n492 = case shown="True" w898 {
                    tunnel: w900 -> [w901 w909]
                    tunnel: [w901 w908] -> w899
                    frame False {
                      # "we are not measuring in phase signal on lock-in (address 1)"
                    }
                    frame True {
                      w906 = "1"
                      # "we are  measuring lock-in (address 1), in phase"
                      n493 = GPIB Write(0:w906, 1:"OUTP?1") -> (6:w907:errorcluster)  [unwired: 3 in, 1 out]
                      n494 = GPIB Read(0:w906, 1:3200, 3:w907) -> (5:w904:string)  [unwired: 2 in, 2 out]
                      n495 = Fract/Exp String To Number(string=w904) -> (number=w903:dbl)  [unwired: 3 in, 1 out]
                      n496 = Build Array (concatenate)(w909, w903) -> (w908:dbl[])
                    }
                  }
                  n497 = property on="array for data" class="Arr (strict)"("Value"=w899) -> ()  [unwired: 2 in, 2 out]
                }
                frame #2 {
                  # "check if out-of-phase\nsignal on lock-in \n(address 1) is to\nbe measured"
                  n498 = property on="Addr 1 lock-in oop" class="Bool (strict)"() -> ("Value"=w910:bool)  [unwired: 2 in, 2 out]
                  n499 = property on="array for data" class="Arr (strict)"() -> ("Value"=w912:dbl[])  [unwired: 2 in, 2 out]
                  n500 = case shown="True" w910 {
                    tunnel: w912 -> [w913 w921]
                    tunnel: [w913 w920] -> w911
                    frame False {
                      # "we are not measuring out-of-phase signal on lock-in (address 1)"
                    }
                    frame True {
                      w918 = "1"
                      # "we are  measuring lock-in (address 1), out-of-phase signal"
                      n501 = GPIB Write(0:w918, 1:"OUTP?2") -> (6:w919:errorcluster)  [unwired: 3 in, 1 out]
                      n502 = GPIB Read(0:w918, 1:3200, 3:w919) -> (5:w916:string)  [unwired: 2 in, 2 out]
                      n503 = Fract/Exp String To Number(string=w916) -> (number=w915:dbl)  [unwired: 3 in, 1 out]
                      n504 = Build Array (concatenate)(w921, w915) -> (w920:dbl[])
                    }
                  }
                  n505 = property on="array for data" class="Arr (strict)"("Value"=w911) -> ()  [unwired: 2 in, 2 out]
                }
                frame #3 {
                  # "check if in-phase\nsignal on lock-in \n(address 2) is to\nbe measured"
                  n506 = property on="Addr 2 lock-in" class="Bool (strict)"() -> ("Value"=w922:bool)  [unwired: 2 in, 2 out]
                  n507 = property on="array for data" class="Arr (strict)"() -> ("Value"=w924:dbl[])  [unwired: 2 in, 2 out]
                  n508 = case shown="False" w922 {
                    tunnel: w924 -> [w925 w933]
                    tunnel: [w925 w932] -> w923
                    frame False {
                      # "we are not measuring in phase signal on lock-in (address 2)"
                    }
                    frame True {
                      w930 = "2"
                      # "we are  measuring lock-in (address 2), in phase"
                      n509 = GPIB Write(0:w930, 1:"OUTP?1") -> (6:w931:errorcluster)  [unwired: 3 in, 1 out]
                      n510 = GPIB Read(0:w930, 1:3200, 3:w931) -> (5:w928:string)  [unwired: 2 in, 2 out]
                      n511 = Fract/Exp String To Number(string=w928) -> (number=w927:dbl)  [unwired: 3 in, 1 out]
                      n512 = Build Array (concatenate)(w933, w927) -> (w932:dbl[])
                    }
                  }
                  n513 = property on="array for data" class="Arr (strict)"("Value"=w923) -> ()  [unwired: 2 in, 2 out]
                }
                frame #4 {
                  # "check if out-of-phase\nsignal on lock-in \n(address 2) is to\nbe measured"
                  n514 = property on="Addr 2 lock-in oop" class="Bool (strict)"() -> ("Value"=w934:bool)  [unwired: 2 in, 2 out]
                  n515 = property on="array for data" class="Arr (strict)"() -> ("Value"=w936:dbl[])  [unwired: 2 in, 2 out]
                  n516 = case shown="False" w934 {
                    tunnel: w936 -> [w937 w945]
                    tunnel: [w937 w944] -> w935
                    tunnel: w934 -> [_ _]
                    frame False {
                      # "we are not measuring out-of-phase signal on lock-in (address 2)"
                    }
                    frame True {
                      w942 = "2"
                      # "we are  measuring lock-in (address 2), out-of-phase"
                      n517 = GPIB Write(0:w942, 1:"OUTP?2") -> (6:w943:errorcluster)  [unwired: 3 in, 1 out]
                      n518 = GPIB Read(0:w942, 1:3200, 3:w943) -> (5:w940:string)  [unwired: 2 in, 2 out]
                      n519 = Fract/Exp String To Number(string=w940) -> (number=w939:dbl)  [unwired: 3 in, 1 out]
                      n520 = Build Array (concatenate)(w945, w939) -> (w944:dbl[])
                    }
                  }
                  n521 = property on="array for data" class="Arr (strict)"("Value"=w935) -> ()  [unwired: 2 in, 2 out]
                }
                frame #5 {
                  # "check if in-phase\nsignal on lock-in \n(address 3) is to\nbe measured"
                  n522 = property on="Addr 3 lock-in" class="Bool (strict)"() -> ("Value"=w946:bool)  [unwired: 2 in, 2 out]
                  n523 = property on="array for data" class="Arr (strict)"() -> ("Value"=w948:dbl[])  [unwired: 2 in, 2 out]
                  n524 = case shown="True" w946 {
                    tunnel: w948 -> [w949 w957]
                    tunnel: [w949 w956] -> w947
                    frame False {
                      # "we are not measuring in phase signal on lock-in (address 3)"
                    }
                    frame True {
                      w954 = "3"
                      # "we are  measuring lock-in (address 3), in phase"
                      n525 = GPIB Write(0:w954, 1:"OUTP?1") -> (6:w955:errorcluster)  [unwired: 3 in, 1 out]
                      n526 = GPIB Read(0:w954, 1:3200, 3:w955) -> (5:w952:string)  [unwired: 2 in, 2 out]
                      n527 = Fract/Exp String To Number(string=w952) -> (number=w951:dbl)  [unwired: 3 in, 1 out]
                      n528 = Build Array (concatenate)(w957, w951) -> (w956:dbl[])
                    }
                  }
                  n529 = property on="array for data" class="Arr (strict)"("Value"=w947) -> ()  [unwired: 2 in, 2 out]
                }
                frame #6 {
                  # "check if out-of-phase\nsignal on lock-in \n(address 3) is to\nbe measured"
                  n530 = property on="Addr 3 lock-in oop" class="Bool (strict)"() -> ("Value"=w958:bool)  [unwired: 2 in, 2 out]
                  n531 = property on="array for data" class="Arr (strict)"() -> ("Value"=w960:dbl[])  [unwired: 2 in, 2 out]
                  n532 = case shown="True" w958 {
                    tunnel: w960 -> [w961 w969]
                    tunnel: [w961 w968] -> w959
                    frame False {
                      # "we are not measuring out-of-phase signal on lock-in (address 3)"
                    }
                    frame True {
                      w966 = "3"
                      # "we are  measuring lock-in (address 3), out-of-phase"
                      n533 = GPIB Write(0:w966, 1:"OUTP?2") -> (6:w967:errorcluster)  [unwired: 3 in, 1 out]
                      n534 = GPIB Read(0:w966, 1:3200, 3:w967) -> (5:w964:string)  [unwired: 2 in, 2 out]
                      n535 = Fract/Exp String To Number(string=w964) -> (number=w963:dbl)  [unwired: 3 in, 1 out]
                      n536 = Build Array (concatenate)(w969, w963) -> (w968:dbl[])
                    }
                  }
                  n537 = property on="array for data" class="Arr (strict)"("Value"=w959) -> ()  [unwired: 2 in, 2 out]
                }
                frame #7 {
                  # "check if in-phase\nsignal on lock-in \n(address 4) is to\nbe measured"
                  n538 = property on="Addr 4 lock-in" class="Bool (strict)"() -> ("Value"=w970:bool)  [unwired: 2 in, 2 out]
                  n539 = property on="array for data" class="Arr (strict)"() -> ("Value"=w972:dbl[])  [unwired: 2 in, 2 out]
                  n540 = case shown="True" w970 {
                    tunnel: w972 -> [w973 w981]
                    tunnel: [w973 w980] -> w971
                    frame False {
                      # "we are not measuring in phase signal on lock-in (address 4)"
                    }
                    frame True {
                      w978 = "4"
                      # "we are  measuring lock-in (address 4), in phase"
                      n541 = GPIB Write(0:w978, 1:"OUTP?1") -> (6:w979:errorcluster)  [unwired: 3 in, 1 out]
                      n542 = GPIB Read(0:w978, 1:3200, 3:w979) -> (5:w976:string)  [unwired: 2 in, 2 out]
                      n543 = Fract/Exp String To Number(string=w976) -> (number=w975:dbl)  [unwired: 3 in, 1 out]
                      n544 = Build Array (concatenate)(w981, w975) -> (w980:dbl[])
                    }
                  }
                  n545 = property on="array for data" class="Arr (strict)"("Value"=w971) -> ()  [unwired: 2 in, 2 out]
                }
                frame #8 {
                  # "check if out-of-phase\nsignal on lock-in \n(address 4) is to\nbe measured"
                  n546 = property on="Addr 4 lock-in oop" class="Bool (strict)"() -> ("Value"=w982:bool)  [unwired: 2 in, 2 out]
                  n547 = property on="array for data" class="Arr (strict)"() -> ("Value"=w984:dbl[])  [unwired: 2 in, 2 out]
                  n548 = case shown="True" w982 {
                    tunnel: w984 -> [w985 w993]
                    tunnel: [w985 w992] -> w983
                    frame False {
                      # "we are not measuring out-of-phase signal on lock-in (address 4)"
                    }
                    frame True {
                      w990 = "4"
                      # "we are  measuring lock-in (address 4), out-of-phase"
                      n549 = GPIB Write(0:w990, 1:"OUTP?2") -> (6:w991:errorcluster)  [unwired: 3 in, 1 out]
                      n550 = GPIB Read(0:w990, 1:3200, 3:w991) -> (5:w988:string)  [unwired: 2 in, 2 out]
                      n551 = Fract/Exp String To Number(string=w988) -> (number=w987:dbl)  [unwired: 3 in, 1 out]
                      n552 = Build Array (concatenate)(w993, w987) -> (w992:dbl[])
                    }
                  }
                  n553 = property on="array for data" class="Arr (strict)"("Value"=w983) -> ()  [unwired: 2 in, 2 out]
                }
                frame #9 {
                  # "check if in-phase\nsignal on lock-in \n(address 5) is to\nbe measured"
                  n554 = property on="Addr 5 lock-in" class="Bool (strict)"() -> ("Value"=w994:bool)  [unwired: 2 in, 2 out]
                  n555 = property on="array for data" class="Arr (strict)"() -> ("Value"=w996:dbl[])  [unwired: 2 in, 2 out]
                  n556 = case shown="False" w994 {
                    tunnel: w996 -> [w997 w1005]
                    tunnel: [w997 w1004] -> w995
                    frame False {
                      # "we are not measuring in phase signal on lock-in (address 5)"
                    }
                    frame True {
                      w1002 = "5"
                      # "we are  measuring lock-in (address 5), in phase"
                      n557 = GPIB Write(0:w1002, 1:"OUTP?1") -> (6:w1003:errorcluster)  [unwired: 3 in, 1 out]
                      n558 = GPIB Read(0:w1002, 1:3200, 3:w1003) -> (5:w1000:string)  [unwired: 2 in, 2 out]
                      n559 = Fract/Exp String To Number(string=w1000) -> (number=w999:dbl)  [unwired: 3 in, 1 out]
                      n560 = Build Array (concatenate)(w1005, w999) -> (w1004:dbl[])
                    }
                  }
                  n561 = property on="array for data" class="Arr (strict)"("Value"=w995) -> ()  [unwired: 2 in, 2 out]
                }
                frame #10 {
                  # "check if out-of-phase\nsignal on lock-in \n(address 5) is to\nbe measured"
                  n562 = property on="Addr 5 lock-in oop" class="Bool (strict)"() -> ("Value"=w1006:bool)  [unwired: 2 in, 2 out]
                  n563 = property on="array for data" class="Arr (strict)"() -> ("Value"=w1008:dbl[])  [unwired: 2 in, 2 out]
                  n564 = case shown="False" w1006 {
                    tunnel: w1008 -> [w1009 w1017]
                    tunnel: [w1009 w1016] -> w1007
                    frame False {
                      # "we are not measuring out-of-phase signal on lock-in (address 5)"
                    }
                    frame True {
                      w1014 = "5"
                      # "we are  measuring lock-in (address 5), out-of-phase"
                      n565 = GPIB Write(0:w1014, 1:"OUTP?2") -> (6:w1015:errorcluster)  [unwired: 3 in, 1 out]
                      n566 = GPIB Read(0:w1014, 1:3200, 3:w1015) -> (5:w1012:string)  [unwired: 2 in, 2 out]
                      n567 = Fract/Exp String To Number(string=w1012) -> (number=w1011:dbl)  [unwired: 3 in, 1 out]
                      n568 = Build Array (concatenate)(w1017, w1011) -> (w1016:dbl[])
                    }
                  }
                  n569 = property on="array for data" class="Arr (strict)"("Value"=w1007) -> ()  [unwired: 2 in, 2 out]
                }
                frame #11 {
                  # "check if voltage on \nmain Keithley 2400 \n(addr. 12) is to\nbe measured"
                  n570 = property on="Voltage (Vk1)" class="Bool (strict)"() -> ("Value"=w1018:bool)  [unwired: 2 in, 2 out]
                  n571 = property on="array for data" class="Arr (strict)"() -> ("Value"=w1020:dbl[])  [unwired: 2 in, 2 out]
                  n572 = case shown="False" w1018 {
                    tunnel: w1020 -> [w1021 w1031]
                    tunnel: [w1021 w1030] -> w1019
                    frame False {
                      # "we aren't measuring voltage \non main Keithley 2400 (addr. 12)"
                    }
                    frame True {
                      w1028 = "12"
                      # "we are measuring voltage \non main Keithley 2400 (addr. 12)"
                      n573 = GPIB Write(0:w1028, 1:":READ?") -> (6:w1029:errorcluster)  [unwired: 3 in, 1 out]
                      n574 = GPIB Read(0:w1028, 1:3200, 3:w1029) -> (5:w1024:string)  [unwired: 2 in, 2 out]
                      n575 = String Subset(string=w1024, length (rest)=13) -> (substring=w1023:string)  [unwired: 1 in]
                      n576 = Fract/Exp String To Number(string=w1023) -> (number=w1026:dbl)  [unwired: 3 in, 1 out]
                      n577 = Build Array (concatenate)(w1031, w1026) -> (w1030:dbl[])
                    }
                  }
                  n578 = property on="array for data" class="Arr (strict)"("Value"=w1019) -> ()  [unwired: 2 in, 2 out]
                }
                frame #12 {
                  # "check if  current on \nmain Keithley 2400 \n(addr. 12) is to\nbe measured"
                  n579 = property on="Current (Ik1)" class="Bool (strict)"() -> ("Value"=w1032:bool)  [unwired: 2 in, 2 out]
                  n580 = property on="array for data" class="Arr (strict)"() -> ("Value"=w1034:dbl[])  [unwired: 2 in, 2 out]
                  n581 = case shown="True" w1032 {
                    tunnel: w1034 -> [w1035 w1046]
                    tunnel: [w1035 w1045] -> w1033
                    frame False {
                      # "we aren't measuring current \non main Keithley 2400 (addr. 12)"
                    }
                    frame True {
                      w1043 = "12"
                      # "we are measuring current\non main Keithley 2400 (addr. 12)"
                      n582 = GPIB Write(0:w1043, 1:":READ?") -> (6:w1044:errorcluster)  [unwired: 3 in, 1 out]
                      n583 = GPIB Read(0:w1043, 1:3200, 3:w1044) -> (5:w1039:string)  [unwired: 2 in, 2 out]
                      n584 = String Subset(string=w1039, offset (0)=14, length (rest)=13) -> (substring=w1038:string)
                      n585 = Fract/Exp String To Number(string=w1038) -> (number=w1041:dbl)  [unwired: 3 in, 1 out]
                      n586 = Build Array (concatenate)(w1046, w1041) -> (w1045:dbl[])
                    }
                  }
                  n587 = property on="array for data" class="Arr (strict)"("Value"=w1033) -> ()  [unwired: 2 in, 2 out]
                }
                frame #13 {
                  # "check if voltage on \nadd. Keithley 2400 \n(addr. 13) is to\nbe measured"
                  n588 = property on="Voltage (Vk2)" class="Bool (strict)"() -> ("Value"=w1047:bool)  [unwired: 2 in, 2 out]
                  n589 = property on="array for data" class="Arr (strict)"() -> ("Value"=w1049:dbl[])  [unwired: 2 in, 2 out]
                  n590 = case shown="True" w1047 {
                    tunnel: w1049 -> [w1050 w1060]
                    tunnel: [w1050 w1059] -> w1048
                    frame False {
                      # "we aren't measuring voltage \non additional Keithley 2400 (addr. 13)"
                    }
                    frame True {
                      w1057 = "13"
                      # "we are measuring voltage \non additional Keithley 2400 (addr. 13)"
                      n591 = GPIB Write(0:w1057, 1:":READ?") -> (6:w1058:errorcluster)  [unwired: 3 in, 1 out]
                      n592 = GPIB Read(0:w1057, 1:3200, 3:w1058) -> (5:w1053:string)  [unwired: 2 in, 2 out]
                      n593 = String Subset(string=w1053, length (rest)=13) -> (substring=w1052:string)  [unwired: 1 in]
                      n594 = Fract/Exp String To Number(string=w1052) -> (number=w1055:dbl)  [unwired: 3 in, 1 out]
                      n595 = Build Array (concatenate)(w1060, w1055) -> (w1059:dbl[])
                    }
                  }
                  n596 = property on="array for data" class="Arr (strict)"("Value"=w1048) -> ()  [unwired: 2 in, 2 out]
                }
                frame #14 {
                  # "check if  current on \nadd. Keithley 2400 \n(addr. 13) is to\nbe measured"
                  n597 = property on="Current (Ik2)" class="Bool (strict)"() -> ("Value"=w1061:bool)  [unwired: 2 in, 2 out]
                  n598 = property on="array for data" class="Arr (strict)"() -> ("Value"=w1063:dbl[])  [unwired: 2 in, 2 out]
                  n599 = case shown="True" w1061 {
                    tunnel: w1063 -> [w1064 w1075]
                    tunnel: [w1064 w1074] -> w1062
                    frame False {
                      # "we aren't measuring current \non additional Keithley 2400 (addr. 13)"
                    }
                    frame True {
                      w1072 = "13"
                      # "we are measuring current\non additional Keithley 2400 (addr. 13)"
                      n600 = GPIB Write(0:w1072, 1:":READ?") -> (6:w1073:errorcluster)  [unwired: 3 in, 1 out]
                      n601 = GPIB Read(0:w1072, 1:3200, 3:w1073) -> (5:w1068:string)  [unwired: 2 in, 2 out]
                      n602 = String Subset(string=w1068, offset (0)=14, length (rest)=13) -> (substring=w1067:string)
                      n603 = Fract/Exp String To Number(string=w1067) -> (number=w1070:dbl)  [unwired: 3 in, 1 out]
                      n604 = Build Array (concatenate)(w1075, w1070) -> (w1074:dbl[])
                    }
                  }
                  n605 = property on="array for data" class="Arr (strict)"("Value"=w1062) -> ()  [unwired: 2 in, 2 out]
                }
                frame #15 {
                  # "check if voltage on \nadd. Keithley 2400 \n(addr. 14) is to\nbe measured"
                  n606 = property on="Voltage (Vk3)" class="Bool (strict)"() -> ("Value"=w1076:bool)  [unwired: 2 in, 2 out]
                  n607 = property on="array for data" class="Arr (strict)"() -> ("Value"=w1078:dbl[])  [unwired: 2 in, 2 out]
                  n608 = case shown="False" w1076 {
                    tunnel: w1078 -> [w1079 w1089]
                    tunnel: [w1079 w1088] -> w1077
                    frame False {
                      # "we aren't measuring voltage \non additional Keithley 2400 (addr. 14)"
                    }
                    frame True {
                      w1086 = "14"
                      # "we are measuring voltage \non additional Keithley 2400 (addr. 14)"
                      n609 = GPIB Write(0:w1086, 1:":READ?") -> (6:w1087:errorcluster)  [unwired: 3 in, 1 out]
                      n610 = GPIB Read(0:w1086, 1:3200, 3:w1087) -> (5:w1082:string)  [unwired: 2 in, 2 out]
                      n611 = String Subset(string=w1082, length (rest)=13) -> (substring=w1081:string)  [unwired: 1 in]
                      n612 = Fract/Exp String To Number(string=w1081) -> (number=w1084:dbl)  [unwired: 3 in, 1 out]
                      n613 = Build Array (concatenate)(w1089, w1084) -> (w1088:dbl[])
                    }
                  }
                  n614 = property on="array for data" class="Arr (strict)"("Value"=w1077) -> ()  [unwired: 2 in, 2 out]
                }
                frame #16 {
                  # "check if  current on \nadd. Keithley 2400 \n(addr. 14) is to\nbe measured"
                  n615 = property on="Current (Ik3)" class="Bool (strict)"() -> ("Value"=w1090:bool)  [unwired: 2 in, 2 out]
                  n616 = property on="array for data" class="Arr (strict)"() -> ("Value"=w1092:dbl[])  [unwired: 2 in, 2 out]
                  n617 = case shown="True" w1090 {
                    tunnel: w1092 -> [w1093 w1104]
                    tunnel: [w1093 w1103] -> w1091
                    frame False {
                      # "we aren't measuring current \non additional Keithley 2400 (addr. 14)"
                    }
                    frame True {
                      w1101 = "14"
                      # "we are measuring current\non additional Keithley 2400 (addr. 14)"
                      n618 = GPIB Write(0:w1101, 1:":READ?") -> (6:w1102:errorcluster)  [unwired: 3 in, 1 out]
                      n619 = GPIB Read(0:w1101, 1:3200, 3:w1102) -> (5:w1097:string)  [unwired: 2 in, 2 out]
                      n620 = String Subset(string=w1097, offset (0)=14, length (rest)=13) -> (substring=w1096:string)
                      n621 = Fract/Exp String To Number(string=w1096) -> (number=w1099:dbl)  [unwired: 3 in, 1 out]
                      n622 = Build Array (concatenate)(w1104, w1099) -> (w1103:dbl[])
                    }
                  }
                  n623 = property on="array for data" class="Arr (strict)"("Value"=w1091) -> ()  [unwired: 2 in, 2 out]
                }
                frame #17 {
                  # "check if 1st channel\non Keithley 2182 \n(addr. 15) is to\nbe measured"
                  n624 = property on="Channel 1 (Vnano1)" class="Bool (strict)"() -> ("Value"=w1105:bool)  [unwired: 2 in, 2 out]
                  n625 = property on="array for data" class="Arr (strict)"() -> ("Value"=w1107:dbl[])  [unwired: 2 in, 2 out]
                  n626 = case shown="True" w1105 {
                    tunnel: w1107 -> [w1108 w1116]
                    tunnel: [w1108 w1115] -> w1106
                    frame False {
                      # "we are not measuring 1st channel\non Keithley 2182 (addr. 15)"
                    }
                    frame True {
                      w1113 = "15"
                      # "we are measuring 1st channel\non Keithley 2182 (addr. 15)"
                      n627 = GPIB Write(0:w1113, 1:":SENSe:DATA:FRES?") -> (6:w1114:errorcluster)  [unwired: 3 in, 1 out]
                      n628 = GPIB Read(0:w1113, 1:200, 3:w1114) -> (5:w1109:string)  [unwired: 2 in, 2 out]
                      n629 = Fract/Exp String To Number(string=w1109) -> (number=w1111:dbl)  [unwired: 3 in, 1 out]
                      n630 = Build Array (concatenate)(w1116, w1111) -> (w1115:dbl[])
                    }
                  }
                  n631 = property on="array for data" class="Arr (strict)"("Value"=w1106) -> ()  [unwired: 2 in, 2 out]
                }
                frame #18 {
                  # "check if 2nd channel\non Keithley 2182 \n(addr. 15) is to\nbe measured"
                  n632 = property on="Channel 2 (Vnano1b)" class="Bool (strict)"() -> ("Value"=w1117:bool)  [unwired: 2 in, 2 out]
                  n633 = property on="array for data" class="Arr (strict)"() -> ("Value"=w1119:dbl[])  [unwired: 2 in, 2 out]
                  n634 = case shown="False" w1117 {
                    tunnel: w1119 -> [w1120 w1132]
                    tunnel: [w1120 w1131] -> w1118
                    frame False {
                      # "we are not measuring 1st channel\non Keithley 2182 (addr. 15)"
                    }
                    frame True {
                      w1123 = "15"
                      # "switching to channel 2 and then\nback to channel 1"
                      # "we are measuring 2nd channel\non Keithley 2182 (addr. 15)"
                      n635 = GPIB Write(0:w1123, 1:":SENSe:CHAN 2") -> (6:w1124:errorcluster)  [unwired: 3 in, 1 out]
                      n636 = GPIB Write(0:w1123, 1:":SENSe:DATA:FRES?", 3:w1124) -> (6:w1130:errorcluster)  [unwired: 2 in, 1 out]
                      n637 = GPIB Read(0:w1123, 1:200, 3:w1130) -> (5:w1126:string, 7:w1122:errorcluster)  [unwired: 2 in, 1 out]
                      n638 = GPIB Write(0:w1123, 1:":SENSe:CHAN 1", 3:w1122) -> ()  [unwired: 2 in, 2 out]
                      n639 = Fract/Exp String To Number(string=w1126) -> (number=w1128:dbl)  [unwired: 3 in, 1 out]
                      n640 = Build Array (concatenate)(w1132, w1128) -> (w1131:dbl[])
                    }
                  }
                  n641 = property on="array for data" class="Arr (strict)"("Value"=w1118) -> ()  [unwired: 2 in, 2 out]
                }
                frame #19 {
                  # "check if 1st channel\non Keithley 2182 \n(addr. 16) is to\nbe measured"
                  n642 = property on="Channel 1 (Vnano2)" class="Bool (strict)"() -> ("Value"=w1133:bool)  [unwired: 2 in, 2 out]
                  n643 = property on="array for data" class="Arr (strict)"() -> ("Value"=w1135:dbl[])  [unwired: 2 in, 2 out]
                  n644 = case shown="True" w1133 {
                    tunnel: w1135 -> [w1136 w1144]
                    tunnel: [w1136 w1143] -> w1134
                    frame False {
                      # "we are not measuring 1st channel\non Keithley 2182 (addr. 16)"
                    }
                    frame True {
                      w1141 = "16"
                      # "we are measuring 1st channel\non Keithley 2182 (addr. 16)"
                      n645 = GPIB Write(0:w1141, 1:":SENSe:DATA:FRES?") -> (6:w1142:errorcluster)  [unwired: 3 in, 1 out]
                      n646 = GPIB Read(0:w1141, 1:200, 3:w1142) -> (5:w1137:string)  [unwired: 2 in, 2 out]
                      n647 = Fract/Exp String To Number(string=w1137) -> (number=w1139:dbl)  [unwired: 3 in, 1 out]
                      n648 = Build Array (concatenate)(w1144, w1139) -> (w1143:dbl[])
                    }
                  }
                  n649 = property on="array for data" class="Arr (strict)"("Value"=w1134) -> ()  [unwired: 2 in, 2 out]
                }
                frame #20 {
                  # "check if 2nd channel\non Keithley 2182 \n(addr. 16) is to\nbe measured"
                  n650 = property on="Channel 2 (Vnano2b)" class="Bool (strict)"() -> ("Value"=w1145:bool)  [unwired: 2 in, 2 out]
                  n651 = property on="array for data" class="Arr (strict)"() -> ("Value"=w1147:dbl[])  [unwired: 2 in, 2 out]
                  n652 = case shown="True" w1145 {
                    tunnel: w1147 -> [w1148 w1160]
                    tunnel: [w1148 w1159] -> w1146
                    frame False {
                      # "we are not measuring 1st channel\non Keithley 2182 (addr. 16)"
                    }
                    frame True {
                      w1151 = "16"
                      # "switching to channel 2 and then\nback to channel 1"
                      # "we are measuring 2nd channel\non Keithley 2182 (addr. 16)"
                      n653 = GPIB Write(0:w1151, 1:":SENSe:CHAN 2") -> (6:w1152:errorcluster)  [unwired: 3 in, 1 out]
                      n654 = GPIB Write(0:w1151, 1:":SENSe:DATA:FRES?", 3:w1152) -> (6:w1158:errorcluster)  [unwired: 2 in, 1 out]
                      n655 = GPIB Read(0:w1151, 1:200, 3:w1158) -> (5:w1154:string, 7:w1150:errorcluster)  [unwired: 2 in, 1 out]
                      n656 = GPIB Write(0:w1151, 1:":SENSe:CHAN 1", 3:w1150) -> ()  [unwired: 2 in, 2 out]
                      n657 = Fract/Exp String To Number(string=w1154) -> (number=w1156:dbl)  [unwired: 3 in, 1 out]
                      n658 = Build Array (concatenate)(w1160, w1156) -> (w1159:dbl[])
                    }
                  }
                  n659 = property on="array for data" class="Arr (strict)"("Value"=w1146) -> ()  [unwired: 2 in, 2 out]
                }
                frame #21 {
                  # "check if 1st channel\non Keithley 2182 \n(addr. 17) is to\nbe measured"
                  n660 = property on="Channel 1 (Vnano3)" class="Bool (strict)"() -> ("Value"=w1161:bool)  [unwired: 2 in, 2 out]
                  n661 = property on="array for data" class="Arr (strict)"() -> ("Value"=w1163:dbl[])  [unwired: 2 in, 2 out]
                  n662 = case shown="True" w1161 {
                    tunnel: w1163 -> [w1164 w1172]
                    tunnel: [w1164 w1171] -> w1162
                    frame False {
                      # "we are not measuring 1st channel\non Keithley 2182 (addr. 17)"
                    }
                    frame True {
                      w1169 = "17"
                      # "we are measuring 1st channel\non Keithley 2182 (addr. 17)"
                      n663 = GPIB Write(0:w1169, 1:":SENSe:DATA:FRES?") -> (6:w1170:errorcluster)  [unwired: 3 in, 1 out]
                      n664 = GPIB Read(0:w1169, 1:200, 3:w1170) -> (5:w1165:string)  [unwired: 2 in, 2 out]
                      n665 = Fract/Exp String To Number(string=w1165) -> (number=w1167:dbl)  [unwired: 3 in, 1 out]
                      n666 = Build Array (concatenate)(w1172, w1167) -> (w1171:dbl[])
                    }
                  }
                  n667 = property on="array for data" class="Arr (strict)"("Value"=w1162) -> ()  [unwired: 2 in, 2 out]
                }
                frame #22 {
                  # "check if 2nd channel\non Keithley 2182 \n(addr. 17) is to\nbe measured"
                  n668 = property on="Channel 2 (Vnano3b)" class="Bool (strict)"() -> ("Value"=w1173:bool)  [unwired: 2 in, 2 out]
                  n669 = property on="array for data" class="Arr (strict)"() -> ("Value"=w1175:dbl[])  [unwired: 2 in, 2 out]
                  n670 = case shown="True" w1173 {
                    tunnel: w1175 -> [w1176 w1188]
                    tunnel: [w1176 w1187] -> w1174
                    frame False {
                      # "we are not measuring 1st channel\non Keithley 2182 (addr. 17)"
                    }
                    frame True {
                      w1179 = "17"
                      # "switching to channel 2 and then\nback to channel 1"
                      # "we are measuring 2nd channel\non Keithley 2182 (addr. 17)"
                      n671 = GPIB Write(0:w1179, 1:":SENSe:CHAN 2") -> (6:w1180:errorcluster)  [unwired: 3 in, 1 out]
                      n672 = GPIB Write(0:w1179, 1:":SENSe:DATA:FRES?", 3:w1180) -> (6:w1186:errorcluster)  [unwired: 2 in, 1 out]
                      n673 = GPIB Read(0:w1179, 1:200, 3:w1186) -> (5:w1182:string, 7:w1178:errorcluster)  [unwired: 2 in, 1 out]
                      n674 = GPIB Write(0:w1179, 1:":SENSe:CHAN 1", 3:w1178) -> ()  [unwired: 2 in, 2 out]
                      n675 = Fract/Exp String To Number(string=w1182) -> (number=w1184:dbl)  [unwired: 3 in, 1 out]
                      n676 = Build Array (concatenate)(w1188, w1184) -> (w1187:dbl[])
                    }
                  }
                  n677 = property on="array for data" class="Arr (strict)"("Value"=w1174) -> ()  [unwired: 2 in, 2 out]
                }
                frame #23 {
                  # "check if 1st \nthermometer on \nOxford ITC \n(address 24) \nis measured"
                  n678 = property on="Thermometer 1 (T1)" class="Bool (strict)"() -> ("Value"=w1189:bool)  [unwired: 2 in, 2 out]
                  n679 = property on="array for data" class="Arr (strict)"() -> ("Value"=w1191:dbl[])  [unwired: 2 in, 2 out]
                  n680 = case shown="True" w1189 {
                    tunnel: w1191 -> [w1192 w1201]
                    tunnel: [w1192 w1200] -> w1190
                    frame False {
                      # "we are not measuring temperature on\nthermometer 1 (addr. 24)"
                    }
                    frame True {
                      w1193 = 1
                      w1198 = "24"
                      # "we are measuring temperature,\nthermometer 1 (addr. 24)"
                      n681 = GPIB Write(0:w1198, 1:"R 1", 2:w1193) -> (6:w1199:errorcluster)  [unwired: 2 in, 1 out]
                      n682 = GPIB Read(0:w1198, 1:200, 2:w1193, 3:w1199) -> (5:w1194:string)  [unwired: 1 in, 2 out]
                      n683 = Fract/Exp String To Number(string=w1194, offset=w1193) -> (number=w1196:dbl)  [unwired: 2 in, 1 out]
                      n684 = Build Array (concatenate)(w1201, w1196) -> (w1200:dbl[])
                    }
                  }
                  n685 = property on="array for data" class="Arr (strict)"("Value"=w1190) -> ()  [unwired: 2 in, 2 out]
                }
                frame #24 {
                  # "check if 1st \nthermometer on \nOxford ITC \n(address 24) \nis measured"
                  n686 = property on="Magnetic Field (B)" class="Bool (strict)"() -> ("Value"=w1202:bool)  [unwired: 2 in, 2 out]
                  n687 = property on="array for data" class="Arr (strict)"() -> ("Value"=w1204:dbl[])  [unwired: 2 in, 2 out]
                  n688 = case shown="True" w1202 {
                    tunnel: w1204 -> [w1205 w1214]
                    tunnel: [w1205 w1213] -> w1203
                    frame False {
                      # "we are not measuringmagnetic field (addr. 25)"
                    }
                    frame True {
                      w1206 = 1
                      w1211 = "25"
                      # "we are measuring magnetic field  (addr. 25)"
                      n689 = GPIB Write(0:w1211, 1:"R 8", 2:w1206) -> (6:w1212:errorcluster)  [unwired: 2 in, 1 out]
                      n690 = GPIB Read(0:w1211, 1:200, 2:w1206, 3:w1212) -> (5:w1207:string)  [unwired: 1 in, 2 out]
                      n691 = Fract/Exp String To Number(string=w1207, offset=w1206) -> (number=w1209:dbl)  [unwired: 2 in, 1 out]
                      n692 = Build Array (concatenate)(w1214, w1209) -> (w1213:dbl[])
                    }
                  }
                  n693 = property on="array for data" class="Arr (strict)"("Value"=w1203) -> ()  [unwired: 2 in, 2 out]
                }
                frame #25 {
                  # "check if capacitance\nand loss (address 28)\nare measured"
                  n694 = property on="Capacitance (C) and Loss (L)" class="Bool (strict)"() -> ("Value"=w1215:bool)  [unwired: 2 in, 2 out]
                  n695 = property on="array for data" class="Arr (strict)"() -> ("Value"=w1217:dbl[])  [unwired: 2 in, 2 out]
                  n696 = case shown="True" w1215 {
                    tunnel: w1217 -> [w1218 w1224]
                    tunnel: [w1218 w1220] -> w1216
                    frame False {
                      # "we are not measuringmagnetic capacitance (addr. 28)"
                    }
                    frame True {
                      # "we are measuring capacitance and loss  (addr. 28)"
                      n697 = stacked-sequence {
                        seq-local: [w1226 _ _] -> [_ _ w1249]
                        tunnel: [_ _ w1243] -> w1219
                        tunnel: [_ _ w1244] -> w1222
                        tunnel: "28" ("data") -> [w1225 w1229 w1238]
                        frame #0 {
                          n698 = GPIB Write(0:w1225, 1:"SINGLE" ("data"), 2:i16 0 ("mode (0)")) -> (6:w1226:errorcluster)  [unwired: 2 in, 1 out]
                        }
                        frame #1 {
                          n699 = while {
                            tunnel: w1229 -> [w1230]
                            i -> [w1231]
                            stop <- w1233 continue-if-true
                            n700 = GPIB Serial Poll(0:w1230) -> (2:w1235:i16)  [unwired: 1 in, 2 out]
                            n701 = Less?(x=w1235, y=i16 128) -> (x < y?=w1233:bool)
                            n702 = Wait (ms)(milliseconds to wait=u32 50) -> ()  [unwired: 1 out]
                            "Numeric 4" <- w1231
                          }
                        }
                        frame #2 {
                          w1236 = i16 2 ("mode (0)")
                          n703 = GPIB Read(0:w1238, 1:200 ("byte count"), 2:i16 2 ("mode (0)"), 3:w1249) -> (5:w1242:string)  [unwired: 1 in, 2 out]
                          n704 = Match Pattern(string=w1242, regular expression="C=") -> (after substring=w1241:string)  [unwired: 1 in, 3 out]
                          n705 = Match Pattern(string=w1241, regular expression="PF L=") -> (after substring=w1239:string)  [unwired: 1 in, 3 out]
                          n706 = Search/Split String(string=w1241, search string/char (-)=" ", offset (0)=w1236) -> (substring before match=w1246:string)  [unwired: 2 out]
                          n707 = Search/Split String(string=w1239, search string/char (-)=" ", offset (0)=w1236) -> (substring before match=w1245:string)  [unwired: 2 out]
                          n708 = Fract/Exp String To Number(string=w1245) -> (number=w1243:dbl)  [unwired: 3 in, 1 out]
                          n709 = Fract/Exp String To Number(string=w1246) -> (number=w1244:dbl)  [unwired: 3 in, 1 out]
                        }
                      }
                      n710 = Build Array (concatenate)(w1224, w1222) -> (w1221:dbl[])
                      n711 = Build Array (concatenate)(w1221, w1219) -> (w1220:dbl[])
                    }
                  }
                  n712 = property on="array for data" class="Arr (strict)"("Value"=w1216) -> ()  [unwired: 2 in, 2 out]
                }
              }
              n713 = property on="Commute SorceMeter" class="RadioBtnsControl (strict)"() -> ("Value"=w864:enum32{"Radio Selection 1", "Radio Selection 2"})  [unwired: 2 in, 2 out]
              n714 = case shown="\"Radio Selection 1\", Default" w864 {
                tunnel: ["13" "14"] -> w867
                frame "Radio Selection 1", Default {
                }
                frame "Radio Selection 2" {
                }
              }
              n715 = GPIB Write(0:w867, 1:":READ?", 3:w866) -> (6:w868:errorcluster)  [unwired: 2 in, 1 out]
              n716 = GPIB Read(0:w867, 1:3200, 3:w868) -> (5:w871:string)  [unwired: 2 in, 2 out]
              n717 = String Subset(string=w871, length (rest)=13) -> (substring=w872:string)  [unwired: 1 in]
              n718 = Fract/Exp String To Number(string=w872) -> (number=w874:dbl)  [unwired: 3 in, 1 out]
              n719 = Multiply(x=w874, y=-1.0) -> (x*y=w879:dbl)
              n720 = Number To Fractional String(number=w879) -> (F-format string=w876:string)  [unwired: 3 in]
              n721 = Concatenate Strings(":INIT:IMM; :SOUR:VOLT:LEV:IMM:AMPL " ("data"), w876) -> (w877:string)
              n722 = GPIB Write(0:w867, 1:w877) -> (6:w865:errorcluster)  [unwired: 3 in, 1 out]
            }
          }
        }
        frame False {
          # "all measurements are done in this stacked sequence; reading from each device is recorded to \"array for data\""
          n723 = stacked-sequence {
            tunnel: w1252 -> [w1254 _ _ _ _ _ _ _ _ _ _ _ _ _ _ _ _ _ _ _ _ _ _ _ _ _]
            tunnel: [w1254 _ _ _ _ _ _ _ _ _ _ _ _ _ _ _ _ _ _ _ _ _ _ _ _ _] -> w1253
            frame #0 {
              # "check if oscillator on \nlock-in (address 1)\nis to be measured"
              n724 = property on="Current is:" class="RadioBtnsControl (strict)"() -> ("Value"=w1257:T1)  [unwired: 2 in, 2 out]
              n725 = property on="array for data" class="Arr (strict)"() -> ("Value"=w1256:dbl[])  [unwired: 2 in, 2 out]
              n726 = Equal?(x=w1257, y=0) -> (x = y?=w1258:bool)
              n727 = case shown="False" w1258 {
                tunnel: w1256 -> [w1260 w1268]
                tunnel: [w1260 w1267] -> w1255
                frame False {
                  # "we are not measuring oscillator from\nlock-in (address 1)"
                }
                frame True {
                  w1264 = "1"
                  # "we are  measuring oscillator"
                  n728 = GPIB Write(0:w1264, 1:"SLVL?") -> (6:w1265:errorcluster)  [unwired: 3 in, 1 out]
                  n729 = GPIB Read(0:w1264, 1:3200, 3:w1265) -> (5:w1262:string)  [unwired: 2 in, 2 out]
                  n730 = Fract/Exp String To Number(string=w1262) -> (number=w1261:dbl)  [unwired: 3 in, 1 out]
                  n731 = Build Array (concatenate)(w1268, w1261) -> (w1267:dbl[])
                }
              }
              n732 = property on="array for data" class="Arr (strict)"("Value"=w1255) -> ()  [unwired: 2 in, 2 out]
            }
            frame #1 {
              # "check if in-phase\nsignal on lock-in \n(address 1) is to\nbe measured"
              n733 = property on="array for data" class="Arr (strict)"() -> ("Value"=w1271:dbl[])  [unwired: 2 in, 2 out]
              n734 = property on="Addr 1 lock-in" class="Bool (strict)"() -> ("Value"=w1269:bool)  [unwired: 2 in, 2 out]
              n735 = case shown="True" w1269 {
                tunnel: w1271 -> [w1272 w1280]
                tunnel: [w1272 w1279] -> w1270
                frame False {
                  # "we are not measuring in phase signal on lock-in (address 1)"
                }
                frame True {
                  w1277 = "1"
                  # "we are  measuring lock-in (address 1), in phase"
                  n736 = GPIB Write(0:w1277, 1:"OUTP?1") -> (6:w1278:errorcluster)  [unwired: 3 in, 1 out]
                  n737 = GPIB Read(0:w1277, 1:3200, 3:w1278) -> (5:w1275:string)  [unwired: 2 in, 2 out]
                  n738 = Fract/Exp String To Number(string=w1275) -> (number=w1274:dbl)  [unwired: 3 in, 1 out]
                  n739 = Build Array (concatenate)(w1280, w1274) -> (w1279:dbl[])
                }
              }
              n740 = property on="array for data" class="Arr (strict)"("Value"=w1270) -> ()  [unwired: 2 in, 2 out]
            }
            frame #2 {
              # "check if out-of-phase\nsignal on lock-in \n(address 1) is to\nbe measured"
              n741 = property on="Addr 1 lock-in oop" class="Bool (strict)"() -> ("Value"=w1281:bool)  [unwired: 2 in, 2 out]
              n742 = property on="array for data" class="Arr (strict)"() -> ("Value"=w1283:dbl[])  [unwired: 2 in, 2 out]
              n743 = case shown="True" w1281 {
                tunnel: w1283 -> [w1284 w1292]
                tunnel: [w1284 w1291] -> w1282
                frame False {
                  # "we are not measuring out-of-phase signal on lock-in (address 1)"
                }
                frame True {
                  w1289 = "1"
                  # "we are  measuring lock-in (address 1), out-of-phase signal"
                  n744 = GPIB Write(0:w1289, 1:"OUTP?2") -> (6:w1290:errorcluster)  [unwired: 3 in, 1 out]
                  n745 = GPIB Read(0:w1289, 1:3200, 3:w1290) -> (5:w1287:string)  [unwired: 2 in, 2 out]
                  n746 = Fract/Exp String To Number(string=w1287) -> (number=w1286:dbl)  [unwired: 3 in, 1 out]
                  n747 = Build Array (concatenate)(w1292, w1286) -> (w1291:dbl[])
                }
              }
              n748 = property on="array for data" class="Arr (strict)"("Value"=w1282) -> ()  [unwired: 2 in, 2 out]
            }
            frame #3 {
              # "check if in-phase\nsignal on lock-in \n(address 2) is to\nbe measured"
              n749 = property on="Addr 2 lock-in" class="Bool (strict)"() -> ("Value"=w1293:bool)  [unwired: 2 in, 2 out]
              n750 = property on="array for data" class="Arr (strict)"() -> ("Value"=w1295:dbl[])  [unwired: 2 in, 2 out]
              n751 = case shown="False" w1293 {
                tunnel: w1295 -> [w1296 w1304]
                tunnel: [w1296 w1303] -> w1294
                frame False {
                  # "we are not measuring in phase signal on lock-in (address 2)"
                }
                frame True {
                  w1301 = "2"
                  # "we are  measuring lock-in (address 2), in phase"
                  n752 = GPIB Write(0:w1301, 1:"OUTP?1") -> (6:w1302:errorcluster)  [unwired: 3 in, 1 out]
                  n753 = GPIB Read(0:w1301, 1:3200, 3:w1302) -> (5:w1299:string)  [unwired: 2 in, 2 out]
                  n754 = Fract/Exp String To Number(string=w1299) -> (number=w1298:dbl)  [unwired: 3 in, 1 out]
                  n755 = Build Array (concatenate)(w1304, w1298) -> (w1303:dbl[])
                }
              }
              n756 = property on="array for data" class="Arr (strict)"("Value"=w1294) -> ()  [unwired: 2 in, 2 out]
            }
            frame #4 {
              # "check if out-of-phase\nsignal on lock-in \n(address 2) is to\nbe measured"
              n757 = property on="Addr 2 lock-in oop" class="Bool (strict)"() -> ("Value"=w1305:bool)  [unwired: 2 in, 2 out]
              n758 = property on="array for data" class="Arr (strict)"() -> ("Value"=w1307:dbl[])  [unwired: 2 in, 2 out]
              n759 = case shown="False" w1305 {
                tunnel: w1307 -> [w1308 w1316]
                tunnel: [w1308 w1315] -> w1306
                tunnel: w1305 -> [_ _]
                frame False {
                  # "we are not measuring out-of-phase signal on lock-in (address 2)"
                }
                frame True {
                  w1313 = "2"
                  # "we are  measuring lock-in (address 2), out-of-phase"
                  n760 = GPIB Write(0:w1313, 1:"OUTP?2") -> (6:w1314:errorcluster)  [unwired: 3 in, 1 out]
                  n761 = GPIB Read(0:w1313, 1:3200, 3:w1314) -> (5:w1311:string)  [unwired: 2 in, 2 out]
                  n762 = Fract/Exp String To Number(string=w1311) -> (number=w1310:dbl)  [unwired: 3 in, 1 out]
                  n763 = Build Array (concatenate)(w1316, w1310) -> (w1315:dbl[])
                }
              }
              n764 = property on="array for data" class="Arr (strict)"("Value"=w1306) -> ()  [unwired: 2 in, 2 out]
            }
            frame #5 {
              # "check if in-phase\nsignal on lock-in \n(address 3) is to\nbe measured"
              n765 = property on="Addr 3 lock-in" class="Bool (strict)"() -> ("Value"=w1317:bool)  [unwired: 2 in, 2 out]
              n766 = property on="array for data" class="Arr (strict)"() -> ("Value"=w1319:dbl[])  [unwired: 2 in, 2 out]
              n767 = case shown="False" w1317 {
                tunnel: w1319 -> [w1320 w1328]
                tunnel: [w1320 w1327] -> w1318
                frame False {
                  # "we are not measuring in phase signal on lock-in (address 3)"
                }
                frame True {
                  w1325 = "3"
                  # "we are  measuring lock-in (address 3), in phase"
                  n768 = GPIB Write(0:w1325, 1:"OUTP?1") -> (6:w1326:errorcluster)  [unwired: 3 in, 1 out]
                  n769 = GPIB Read(0:w1325, 1:3200, 3:w1326) -> (5:w1323:string)  [unwired: 2 in, 2 out]
                  n770 = Fract/Exp String To Number(string=w1323) -> (number=w1322:dbl)  [unwired: 3 in, 1 out]
                  n771 = Build Array (concatenate)(w1328, w1322) -> (w1327:dbl[])
                }
              }
              n772 = property on="array for data" class="Arr (strict)"("Value"=w1318) -> ()  [unwired: 2 in, 2 out]
            }
            frame #6 {
              # "check if out-of-phase\nsignal on lock-in \n(address 3) is to\nbe measured"
              n773 = property on="Addr 3 lock-in oop" class="Bool (strict)"() -> ("Value"=w1329:bool)  [unwired: 2 in, 2 out]
              n774 = property on="array for data" class="Arr (strict)"() -> ("Value"=w1331:dbl[])  [unwired: 2 in, 2 out]
              n775 = case shown="False" w1329 {
                tunnel: w1331 -> [w1332 w1340]
                tunnel: [w1332 w1339] -> w1330
                frame False {
                  # "we are not measuring out-of-phase signal on lock-in (address 3)"
                }
                frame True {
                  w1337 = "3"
                  # "we are  measuring lock-in (address 3), out-of-phase"
                  n776 = GPIB Write(0:w1337, 1:"OUTP?2") -> (6:w1338:errorcluster)  [unwired: 3 in, 1 out]
                  n777 = GPIB Read(0:w1337, 1:3200, 3:w1338) -> (5:w1335:string)  [unwired: 2 in, 2 out]
                  n778 = Fract/Exp String To Number(string=w1335) -> (number=w1334:dbl)  [unwired: 3 in, 1 out]
                  n779 = Build Array (concatenate)(w1340, w1334) -> (w1339:dbl[])
                }
              }
              n780 = property on="array for data" class="Arr (strict)"("Value"=w1330) -> ()  [unwired: 2 in, 2 out]
            }
            frame #7 {
              # "check if in-phase\nsignal on lock-in \n(address 4) is to\nbe measured"
              n781 = property on="Addr 4 lock-in" class="Bool (strict)"() -> ("Value"=w1341:bool)  [unwired: 2 in, 2 out]
              n782 = property on="array for data" class="Arr (strict)"() -> ("Value"=w1343:dbl[])  [unwired: 2 in, 2 out]
              n783 = case shown="False" w1341 {
                tunnel: w1343 -> [w1344 w1352]
                tunnel: [w1344 w1351] -> w1342
                frame False {
                  # "we are not measuring in phase signal on lock-in (address 4)"
                }
                frame True {
                  w1349 = "4"
                  # "we are  measuring lock-in (address 4), in phase"
                  n784 = GPIB Write(0:w1349, 1:"OUTP?1") -> (6:w1350:errorcluster)  [unwired: 3 in, 1 out]
                  n785 = GPIB Read(0:w1349, 1:3200, 3:w1350) -> (5:w1347:string)  [unwired: 2 in, 2 out]
                  n786 = Fract/Exp String To Number(string=w1347) -> (number=w1346:dbl)  [unwired: 3 in, 1 out]
                  n787 = Build Array (concatenate)(w1352, w1346) -> (w1351:dbl[])
                }
              }
              n788 = property on="array for data" class="Arr (strict)"("Value"=w1342) -> ()  [unwired: 2 in, 2 out]
            }
            frame #8 {
              # "check if out-of-phase\nsignal on lock-in \n(address 4) is to\nbe measured"
              n789 = property on="Addr 4 lock-in oop" class="Bool (strict)"() -> ("Value"=w1353:bool)  [unwired: 2 in, 2 out]
              n790 = property on="array for data" class="Arr (strict)"() -> ("Value"=w1355:dbl[])  [unwired: 2 in, 2 out]
              n791 = case shown="False" w1353 {
                tunnel: w1355 -> [w1356 w1364]
                tunnel: [w1356 w1363] -> w1354
                frame False {
                  # "we are not measuring out-of-phase signal on lock-in (address 4)"
                }
                frame True {
                  w1361 = "4"
                  # "we are  measuring lock-in (address 4), out-of-phase"
                  n792 = GPIB Write(0:w1361, 1:"OUTP?2") -> (6:w1362:errorcluster)  [unwired: 3 in, 1 out]
                  n793 = GPIB Read(0:w1361, 1:3200, 3:w1362) -> (5:w1359:string)  [unwired: 2 in, 2 out]
                  n794 = Fract/Exp String To Number(string=w1359) -> (number=w1358:dbl)  [unwired: 3 in, 1 out]
                  n795 = Build Array (concatenate)(w1364, w1358) -> (w1363:dbl[])
                }
              }
              n796 = property on="array for data" class="Arr (strict)"("Value"=w1354) -> ()  [unwired: 2 in, 2 out]
            }
            frame #9 {
              # "check if in-phase\nsignal on lock-in \n(address 5) is to\nbe measured"
              n797 = property on="Addr 5 lock-in" class="Bool (strict)"() -> ("Value"=w1365:bool)  [unwired: 2 in, 2 out]
              n798 = property on="array for data" class="Arr (strict)"() -> ("Value"=w1367:dbl[])  [unwired: 2 in, 2 out]
              n799 = case shown="False" w1365 {
                tunnel: w1367 -> [w1368 w1376]
                tunnel: [w1368 w1375] -> w1366
                frame False {
                  # "we are not measuring in phase signal on lock-in (address 5)"
                }
                frame True {
                  w1373 = "5"
                  # "we are  measuring lock-in (address 5), in phase"
                  n800 = GPIB Write(0:w1373, 1:"OUTP?1") -> (6:w1374:errorcluster)  [unwired: 3 in, 1 out]
                  n801 = GPIB Read(0:w1373, 1:3200, 3:w1374) -> (5:w1371:string)  [unwired: 2 in, 2 out]
                  n802 = Fract/Exp String To Number(string=w1371) -> (number=w1370:dbl)  [unwired: 3 in, 1 out]
                  n803 = Build Array (concatenate)(w1376, w1370) -> (w1375:dbl[])
                }
              }
              n804 = property on="array for data" class="Arr (strict)"("Value"=w1366) -> ()  [unwired: 2 in, 2 out]
            }
            frame #10 {
              # "check if out-of-phase\nsignal on lock-in \n(address 5) is to\nbe measured"
              n805 = property on="Addr 5 lock-in oop" class="Bool (strict)"() -> ("Value"=w1377:bool)  [unwired: 2 in, 2 out]
              n806 = property on="array for data" class="Arr (strict)"() -> ("Value"=w1379:dbl[])  [unwired: 2 in, 2 out]
              n807 = case shown="False" w1377 {
                tunnel: w1379 -> [w1380 w1388]
                tunnel: [w1380 w1387] -> w1378
                frame False {
                  # "we are not measuring out-of-phase signal on lock-in (address 5)"
                }
                frame True {
                  w1385 = "5"
                  # "we are  measuring lock-in (address 5), out-of-phase"
                  n808 = GPIB Write(0:w1385, 1:"OUTP?2") -> (6:w1386:errorcluster)  [unwired: 3 in, 1 out]
                  n809 = GPIB Read(0:w1385, 1:3200, 3:w1386) -> (5:w1383:string)  [unwired: 2 in, 2 out]
                  n810 = Fract/Exp String To Number(string=w1383) -> (number=w1382:dbl)  [unwired: 3 in, 1 out]
                  n811 = Build Array (concatenate)(w1388, w1382) -> (w1387:dbl[])
                }
              }
              n812 = property on="array for data" class="Arr (strict)"("Value"=w1378) -> ()  [unwired: 2 in, 2 out]
            }
            frame #11 {
              # "check if voltage on \nChannel A of main\nKeithley 2614B \n(addr. 12) is to\nbe measured"
              n813 = property on="Voltage (Vk1)" class="Bool (strict)"() -> ("Value"=w1389:bool)  [unwired: 2 in, 2 out]
              n814 = property on="array for data" class="Arr (strict)"() -> ("Value"=w1391:dbl[])  [unwired: 2 in, 2 out]
              n815 = case shown="False" w1389 {
                tunnel: w1391 -> [w1392 w1400]
                tunnel: [w1392 w1399] -> w1390
                frame False {
                  # "we aren't measuring voltage \non main Keithley 2614B Channel A (addr. 12)"
                }
                frame True {
                  (unwired) 13
                  w1397 = "12"
                  # "we are measuring voltage of Channel A \non the main Keithley 2614B (addr. 12)"
                  n816 = GPIB Write(0:w1397, 1:"print(smua.measure.v())") -> (6:w1398:errorcluster)  [unwired: 3 in, 1 out]
                  n817 = GPIB Read(0:w1397, 1:3200, 3:w1398) -> (5:w1393:string)  [unwired: 2 in, 2 out]
                  n818 = Fract/Exp String To Number(string=w1393) -> (number=w1395:dbl)  [unwired: 3 in, 1 out]
                  n819 = Build Array (concatenate)(w1400, w1395) -> (w1399:dbl[])
                }
              }
              n820 = property on="array for data" class="Arr (strict)"("Value"=w1390) -> ()  [unwired: 2 in, 2 out]
            }
            frame #12 {
              # "check if current on \nChannel A of main\nKeithley 2614B \n(addr. 12) is to\nbe measured"
              n821 = property on="Current (Ik1)" class="Bool (strict)"() -> ("Value"=w1401:bool)  [unwired: 2 in, 2 out]
              n822 = property on="array for data" class="Arr (strict)"() -> ("Value"=w1403:dbl[])  [unwired: 2 in, 2 out]
              n823 = case shown="True" w1401 {
                tunnel: w1403 -> [w1404 w1406]
                tunnel: [w1404 w1405] -> w1402
                frame False {
                  # "we aren't measuring current \non main Keithley 2400 (addr. 12)"
                }
                frame True {
                  w1411 = "12"
                  # "we are measuring current of Channel A \non the main Keithley 2614B (addr. 12)"
                  n824 = GPIB Write(0:w1411, 1:"print(smua.measure.i())") -> (6:w1412:errorcluster)  [unwired: 3 in, 1 out]
                  n825 = GPIB Read(0:w1411, 1:3200, 3:w1412) -> (5:w1407:string)  [unwired: 2 in, 2 out]
                  n826 = Fract/Exp String To Number(string=w1407) -> (number=w1409:dbl)  [unwired: 3 in, 1 out]
                  n827 = Build Array (concatenate)(w1406, w1409) -> (w1405:dbl[])
                }
              }
              n828 = property on="array for data" class="Arr (strict)"("Value"=w1402) -> ()  [unwired: 2 in, 2 out]
            }
            frame #13 {
              # "check if voltage on \nChannel B of main\nKeithley 2614B \n(addr. 12) is to\nbe measured"
              n829 = property on="Voltage (Vk2)" class="Bool (strict)"() -> ("Value"=w1413:bool)  [unwired: 2 in, 2 out]
              n830 = property on="array for data" class="Arr (strict)"() -> ("Value"=w1415:dbl[])  [unwired: 2 in, 2 out]
              n831 = case shown="False" w1413 {
                tunnel: w1415 -> [w1416 w1418]
                tunnel: [w1416 w1417] -> w1414
                frame False {
                  # "we aren't measuring voltage \non additional Keithley 2400 (addr. 13)"
                }
                frame True {
                  w1423 = "12"
                  # "we are measuring voltage of Channel B \non the main Keithley 2614B (addr. 12)"
                  n832 = GPIB Write(0:w1423, 1:"print(smub.measure.v())") -> (6:w1424:errorcluster)  [unwired: 3 in, 1 out]
                  n833 = GPIB Read(0:w1423, 1:3200, 3:w1424) -> (5:w1419:string)  [unwired: 2 in, 2 out]
                  n834 = Fract/Exp String To Number(string=w1419) -> (number=w1421:dbl)  [unwired: 3 in, 1 out]
                  n835 = Build Array (concatenate)(w1418, w1421) -> (w1417:dbl[])
                }
              }
              n836 = property on="array for data" class="Arr (strict)"("Value"=w1414) -> ()  [unwired: 2 in, 2 out]
            }
            frame #14 {
              # "check if current on \nChannel B of main\nKeithley 2614B \n(addr. 12) is to\nbe measured"
              n837 = property on="Current (Ik2)" class="Bool (strict)"() -> ("Value"=w1425:bool)  [unwired: 2 in, 2 out]
              n838 = property on="array for data" class="Arr (strict)"() -> ("Value"=w1427:dbl[])  [unwired: 2 in, 2 out]
              n839 = case shown="False" w1425 {
                tunnel: w1427 -> [w1428 w1430]
                tunnel: [w1428 w1429] -> w1426
                frame False {
                  # "we aren't measuring current \non additional Keithley 2400 (addr. 13)"
                }
                frame True {
                  w1435 = "12"
                  # "we are measuring current of Channel B \non the main Keithley 2614B (addr. 12)"
                  n840 = GPIB Write(0:w1435, 1:"print(smub.measure.i())") -> (6:w1436:errorcluster)  [unwired: 3 in, 1 out]
                  n841 = GPIB Read(0:w1435, 1:3200, 3:w1436) -> (5:w1431:string)  [unwired: 2 in, 2 out]
                  n842 = Fract/Exp String To Number(string=w1431) -> (number=w1433:dbl)  [unwired: 3 in, 1 out]
                  n843 = Build Array (concatenate)(w1430, w1433) -> (w1429:dbl[])
                }
              }
              n844 = property on="array for data" class="Arr (strict)"("Value"=w1426) -> ()  [unwired: 2 in, 2 out]
            }
            frame #15 {
              # "check if voltage on \nadd. Keithley 2400 \n(addr. 14) is to\nbe measured"
              n845 = property on="Voltage (Vk3)" class="Bool (strict)"() -> ("Value"=w1437:bool)  [unwired: 2 in, 2 out]
              n846 = property on="array for data" class="Arr (strict)"() -> ("Value"=w1439:dbl[])  [unwired: 2 in, 2 out]
              n847 = case shown="False" w1437 {
                tunnel: w1439 -> [w1440 w1450]
                tunnel: [w1440 w1449] -> w1438
                frame False {
                  # "we aren't measuring voltage \non additional Keithley 2400 (addr. 14)"
                }
                frame True {
                  w1447 = "14"
                  # "we are measuring voltage \non additional Keithley 2400 (addr. 14)"
                  n848 = GPIB Write(0:w1447, 1:":READ?") -> (6:w1448:errorcluster)  [unwired: 3 in, 1 out]
                  n849 = GPIB Read(0:w1447, 1:3200, 3:w1448) -> (5:w1443:string)  [unwired: 2 in, 2 out]
                  n850 = String Subset(string=w1443, length (rest)=13) -> (substring=w1442:string)  [unwired: 1 in]
                  n851 = Fract/Exp String To Number(string=w1442) -> (number=w1445:dbl)  [unwired: 3 in, 1 out]
                  n852 = Build Array (concatenate)(w1450, w1445) -> (w1449:dbl[])
                }
              }
              n853 = property on="array for data" class="Arr (strict)"("Value"=w1438) -> ()  [unwired: 2 in, 2 out]
            }
            frame #16 {
              # "check if  current on \nadd. Keithley 2400 \n(addr. 14) is to\nbe measured"
              n854 = property on="Current (Ik3)" class="Bool (strict)"() -> ("Value"=w1451:bool)  [unwired: 2 in, 2 out]
              n855 = property on="array for data" class="Arr (strict)"() -> ("Value"=w1453:dbl[])  [unwired: 2 in, 2 out]
              n856 = case shown="False" w1451 {
                tunnel: w1453 -> [w1454 w1465]
                tunnel: [w1454 w1464] -> w1452
                frame False {
                  # "we aren't measuring current \non additional Keithley 2400 (addr. 14)"
                }
                frame True {
                  w1462 = "14"
                  # "we are measuring current\non additional Keithley 2400 (addr. 14)"
                  n857 = GPIB Write(0:w1462, 1:":READ?") -> (6:w1463:errorcluster)  [unwired: 3 in, 1 out]
                  n858 = GPIB Read(0:w1462, 1:3200, 3:w1463) -> (5:w1458:string)  [unwired: 2 in, 2 out]
                  n859 = String Subset(string=w1458, offset (0)=14, length (rest)=13) -> (substring=w1457:string)
                  n860 = Fract/Exp String To Number(string=w1457) -> (number=w1460:dbl)  [unwired: 3 in, 1 out]
                  n861 = Build Array (concatenate)(w1465, w1460) -> (w1464:dbl[])
                }
              }
              n862 = property on="array for data" class="Arr (strict)"("Value"=w1452) -> ()  [unwired: 2 in, 2 out]
            }
            frame #17 {
              # "check if 1st channel\non Keithley 2182 \n(addr. 15) is to\nbe measured"
              n863 = property on="Channel 1 (Vnano1)" class="Bool (strict)"() -> ("Value"=w1466:bool)  [unwired: 2 in, 2 out]
              n864 = property on="array for data" class="Arr (strict)"() -> ("Value"=w1468:dbl[])  [unwired: 2 in, 2 out]
              n865 = case shown="True" w1466 {
                tunnel: w1468 -> [w1469 w1477]
                tunnel: [w1469 w1476] -> w1467
                frame False {
                  # "we are not measuring 1st channel\non Keithley 2182 (addr. 15)"
                }
                frame True {
                  w1474 = "15"
                  # "we are measuring 1st channel\non Keithley 2182 (addr. 15)"
                  n866 = GPIB Write(0:w1474, 1:":SENSe:DATA:FRES?") -> (6:w1475:errorcluster)  [unwired: 3 in, 1 out]
                  n867 = GPIB Read(0:w1474, 1:200, 3:w1475) -> (5:w1470:string)  [unwired: 2 in, 2 out]
                  n868 = Fract/Exp String To Number(string=w1470) -> (number=w1472:dbl)  [unwired: 3 in, 1 out]
                  n869 = Build Array (concatenate)(w1477, w1472) -> (w1476:dbl[])
                }
              }
              n870 = property on="array for data" class="Arr (strict)"("Value"=w1467) -> ()  [unwired: 2 in, 2 out]
            }
            frame #18 {
              # "check if 2nd channel\non Keithley 2182 \n(addr. 15) is to\nbe measured"
              n871 = property on="Channel 2 (Vnano1b)" class="Bool (strict)"() -> ("Value"=w1478:bool)  [unwired: 2 in, 2 out]
              n872 = property on="array for data" class="Arr (strict)"() -> ("Value"=w1480:dbl[])  [unwired: 2 in, 2 out]
              n873 = case shown="False" w1478 {
                tunnel: w1480 -> [w1481 w1493]
                tunnel: [w1481 w1492] -> w1479
                frame False {
                  # "we are not measuring 1st channel\non Keithley 2182 (addr. 15)"
                }
                frame True {
                  w1484 = "15"
                  # "switching to channel 2 and then\nback to channel 1"
                  # "we are measuring 2nd channel\non Keithley 2182 (addr. 15)"
                  n874 = GPIB Write(0:w1484, 1:":SENSe:CHAN 2") -> (6:w1485:errorcluster)  [unwired: 3 in, 1 out]
                  n875 = GPIB Write(0:w1484, 1:":SENSe:DATA:FRES?", 3:w1485) -> (6:w1491:errorcluster)  [unwired: 2 in, 1 out]
                  n876 = GPIB Read(0:w1484, 1:200, 3:w1491) -> (5:w1487:string, 7:w1483:errorcluster)  [unwired: 2 in, 1 out]
                  n877 = GPIB Write(0:w1484, 1:":SENSe:CHAN 1", 3:w1483) -> ()  [unwired: 2 in, 2 out]
                  n878 = Fract/Exp String To Number(string=w1487) -> (number=w1489:dbl)  [unwired: 3 in, 1 out]
                  n879 = Build Array (concatenate)(w1493, w1489) -> (w1492:dbl[])
                }
              }
              n880 = property on="array for data" class="Arr (strict)"("Value"=w1479) -> ()  [unwired: 2 in, 2 out]
            }
            frame #19 {
              # "check if 1st channel\non Keithley 2182 \n(addr. 16) is to\nbe measured"
              n881 = property on="Channel 1 (Vnano2)" class="Bool (strict)"() -> ("Value"=w1494:bool)  [unwired: 2 in, 2 out]
              n882 = property on="array for data" class="Arr (strict)"() -> ("Value"=w1496:dbl[])  [unwired: 2 in, 2 out]
              n883 = case shown="True" w1494 {
                tunnel: w1496 -> [w1497 w1505]
                tunnel: [w1497 w1504] -> w1495
                frame False {
                  # "we are not measuring 1st channel\non Keithley 2182 (addr. 16)"
                }
                frame True {
                  w1502 = "16"
                  # "we are measuring 1st channel\non Keithley 2182 (addr. 16)"
                  n884 = GPIB Write(0:w1502, 1:":SENSe:DATA:FRES?") -> (6:w1503:errorcluster)  [unwired: 3 in, 1 out]
                  n885 = GPIB Read(0:w1502, 1:200, 3:w1503) -> (5:w1498:string)  [unwired: 2 in, 2 out]
                  n886 = Fract/Exp String To Number(string=w1498) -> (number=w1500:dbl)  [unwired: 3 in, 1 out]
                  n887 = Build Array (concatenate)(w1505, w1500) -> (w1504:dbl[])
                }
              }
              n888 = property on="array for data" class="Arr (strict)"("Value"=w1495) -> ()  [unwired: 2 in, 2 out]
            }
            frame #20 {
              # "check if 2nd channel\non Keithley 2182 \n(addr. 16) is to\nbe measured"
              n889 = property on="Channel 2 (Vnano2b)" class="Bool (strict)"() -> ("Value"=w1506:bool)  [unwired: 2 in, 2 out]
              n890 = property on="array for data" class="Arr (strict)"() -> ("Value"=w1508:dbl[])  [unwired: 2 in, 2 out]
              n891 = case shown="False" w1506 {
                tunnel: w1508 -> [w1509 w1521]
                tunnel: [w1509 w1520] -> w1507
                frame False {
                  # "we are not measuring 1st channel\non Keithley 2182 (addr. 16)"
                }
                frame True {
                  w1512 = "16"
                  # "switching to channel 2 and then\nback to channel 1"
                  # "we are measuring 2nd channel\non Keithley 2182 (addr. 16)"
                  n892 = GPIB Write(0:w1512, 1:":SENSe:CHAN 2") -> (6:w1513:errorcluster)  [unwired: 3 in, 1 out]
                  n893 = GPIB Write(0:w1512, 1:":SENSe:DATA:FRES?", 3:w1513) -> (6:w1519:errorcluster)  [unwired: 2 in, 1 out]
                  n894 = GPIB Read(0:w1512, 1:200, 3:w1519) -> (5:w1515:string, 7:w1511:errorcluster)  [unwired: 2 in, 1 out]
                  n895 = GPIB Write(0:w1512, 1:":SENSe:CHAN 1", 3:w1511) -> ()  [unwired: 2 in, 2 out]
                  n896 = Fract/Exp String To Number(string=w1515) -> (number=w1517:dbl)  [unwired: 3 in, 1 out]
                  n897 = Build Array (concatenate)(w1521, w1517) -> (w1520:dbl[])
                }
              }
              n898 = property on="array for data" class="Arr (strict)"("Value"=w1507) -> ()  [unwired: 2 in, 2 out]
            }
            frame #21 {
              # "check if 1st channel\non Keithley 2182 \n(addr. 17) is to\nbe measured"
              n899 = property on="Channel 1 (Vnano3)" class="Bool (strict)"() -> ("Value"=w1522:bool)  [unwired: 2 in, 2 out]
              n900 = property on="array for data" class="Arr (strict)"() -> ("Value"=w1524:dbl[])  [unwired: 2 in, 2 out]
              n901 = case shown="False" w1522 {
                tunnel: w1524 -> [w1525 w1533]
                tunnel: [w1525 w1532] -> w1523
                frame False {
                  # "we are not measuring 1st channel\non Keithley 2182 (addr. 17)"
                }
                frame True {
                  w1530 = "17"
                  # "we are measuring 1st channel\non Keithley 2182 (addr. 17)"
                  n902 = GPIB Write(0:w1530, 1:":SENSe:DATA:FRES?") -> (6:w1531:errorcluster)  [unwired: 3 in, 1 out]
                  n903 = GPIB Read(0:w1530, 1:200, 3:w1531) -> (5:w1526:string)  [unwired: 2 in, 2 out]
                  n904 = Fract/Exp String To Number(string=w1526) -> (number=w1528:dbl)  [unwired: 3 in, 1 out]
                  n905 = Build Array (concatenate)(w1533, w1528) -> (w1532:dbl[])
                }
              }
              n906 = property on="array for data" class="Arr (strict)"("Value"=w1523) -> ()  [unwired: 2 in, 2 out]
            }
            frame #22 {
              # "check if 2nd channel\non Keithley 2182 \n(addr. 17) is to\nbe measured"
              n907 = property on="Channel 2 (Vnano3b)" class="Bool (strict)"() -> ("Value"=w1534:bool)  [unwired: 2 in, 2 out]
              n908 = property on="array for data" class="Arr (strict)"() -> ("Value"=w1536:dbl[])  [unwired: 2 in, 2 out]
              n909 = case shown="False" w1534 {
                tunnel: w1536 -> [w1537 w1549]
                tunnel: [w1537 w1548] -> w1535
                frame False {
                  # "we are not measuring 1st channel\non Keithley 2182 (addr. 17)"
                }
                frame True {
                  w1540 = "17"
                  # "switching to channel 2 and then\nback to channel 1"
                  # "we are measuring 2nd channel\non Keithley 2182 (addr. 17)"
                  n910 = GPIB Write(0:w1540, 1:":SENSe:CHAN 2") -> (6:w1541:errorcluster)  [unwired: 3 in, 1 out]
                  n911 = GPIB Write(0:w1540, 1:":SENSe:DATA:FRES?", 3:w1541) -> (6:w1547:errorcluster)  [unwired: 2 in, 1 out]
                  n912 = GPIB Read(0:w1540, 1:200, 3:w1547) -> (5:w1543:string, 7:w1539:errorcluster)  [unwired: 2 in, 1 out]
                  n913 = GPIB Write(0:w1540, 1:":SENSe:CHAN 1", 3:w1539) -> ()  [unwired: 2 in, 2 out]
                  n914 = Fract/Exp String To Number(string=w1543) -> (number=w1545:dbl)  [unwired: 3 in, 1 out]
                  n915 = Build Array (concatenate)(w1549, w1545) -> (w1548:dbl[])
                }
              }
              n916 = property on="array for data" class="Arr (strict)"("Value"=w1535) -> ()  [unwired: 2 in, 2 out]
            }
            frame #23 {
              # "check if 1st \nthermometer on \nOxford ITC \n(address 24) \nis measured"
              n917 = property on="Thermometer 1 (T1)" class="Bool (strict)"() -> ("Value"=w1550:bool)  [unwired: 2 in, 2 out]
              n918 = property on="array for data" class="Arr (strict)"() -> ("Value"=w1552:dbl[])  [unwired: 2 in, 2 out]
              n919 = case shown="True" w1550 {
                tunnel: w1552 -> [w1553 w1565]
                tunnel: [w1553 w1564] -> w1551
                frame False {
                  # "we are not measuring temperature on\nthermometer 1 (addr. 24)"
                }
                frame True {
                  (unwired) "\r"
                  w1558 = refnum<visa-resource-name> "TCPIP0::192.168.128.2::7020::SOCKET" ("VISA resource name")
                  # "we are measuring temperature,\nthermometer 1 (addr. 24)"
                  n920 = Concatenate Strings("READ:DEV:MB1.T1:TEMP:SIG:TEMP" ("string"), "\n") -> (w1557:string)
                  n921 = VISA Write(VISA resource name=w1558, write buffer=w1557) -> (error out=w1563:errorcluster)  [unwired: 1 in, 2 out]
                  n922 = String Length(string=w1557) -> (length=w1554:i32)
                  n923 = VISA Read(VISA resource name=w1558, byte count=1024, error in (no error)=w1563) -> (read buffer=w1561:string)  [unwired: 3 out]
                  n924 = String Subset(string=w1561, offset (0)=w1554) -> (substring=w1560:string)  [unwired: 1 in]
                  n925 = Fract/Exp String To Number(string=w1560) -> (number=w1556:dbl)  [unwired: 3 in, 1 out]
                  n926 = Build Array (concatenate)(w1565, w1556) -> (w1564:dbl[])
                }
              }
              n927 = property on="array for data" class="Arr (strict)"("Value"=w1551) -> ()  [unwired: 2 in, 2 out]
            }
            frame #24 {
              # "check if 1st \nthermometer on \nOxford ITC \n(address 24) \nis measured"
              n928 = property on="Magnetic Field (B)" class="Bool (strict)"() -> ("Value"=w1566:bool)  [unwired: 2 in, 2 out]
              n929 = property on="array for data" class="Arr (strict)"() -> ("Value"=w1568:dbl[])  [unwired: 2 in, 2 out]
              n930 = case shown="True" w1566 {
                tunnel: w1568 -> [w1569 w1581]
                tunnel: [w1569 w1580] -> w1567
                frame False {
                  # "we are not measuringmagnetic field (addr. 25)"
                }
                frame True {
                  (unwired) "\r"
                  w1574 = refnum<visa-resource-name> "TCPIP0::192.168.128.3::7020::SOCKET" ("VISA resource name")
                  # "we are measuring magnetic field  (addr. 25)"
                  n931 = Concatenate Strings("READ:DEV:GRPZ:PSU:SIG:PFLD" ("string"), "\n") -> (w1573:string)
                  n932 = VISA Write(VISA resource name=w1574, write buffer=w1573) -> (error out=w1579:errorcluster)  [unwired: 1 in, 2 out]
                  n933 = String Length(string=w1573) -> (length=w1570:i32)
                  n934 = VISA Read(VISA resource name=w1574, byte count=1024, error in (no error)=w1579) -> (read buffer=w1577:string)  [unwired: 3 out]
                  n935 = String Subset(string=w1577, offset (0)=w1570) -> (substring=w1576:string)  [unwired: 1 in]
                  n936 = Fract/Exp String To Number(string=w1576) -> (number=w1572:dbl)  [unwired: 3 in, 1 out]
                  n937 = Build Array (concatenate)(w1581, w1572) -> (w1580:dbl[])
                }
              }
              n938 = property on="array for data" class="Arr (strict)"("Value"=w1567) -> ()  [unwired: 2 in, 2 out]
            }
            frame #25 {
              # "check if capacitance\nand loss (address 28)\nare measured"
              n939 = property on="Capacitance (C) and Loss (L)" class="Bool (strict)"() -> ("Value"=w1582:bool)  [unwired: 2 in, 2 out]
              n940 = property on="array for data" class="Arr (strict)"() -> ("Value"=w1584:dbl[])  [unwired: 2 in, 2 out]
              n941 = case shown="False" w1582 {
                tunnel: w1584 -> [w1585 w1591]
                tunnel: [w1585 w1587] -> w1583
                frame False {
                  # "we are not measuringmagnetic capacitance (addr. 28)"
                }
                frame True {
                  # "we are measuring capacitance and loss  (addr. 28)"
                  n942 = stacked-sequence {
                    seq-local: [w1593 _ _] -> [_ _ w1616]
                    tunnel: [_ _ w1610] -> w1586
                    tunnel: [_ _ w1611] -> w1589
                    tunnel: "28" ("data") -> [w1592 w1596 w1605]
                    frame #0 {
                      n943 = GPIB Write(0:w1592, 1:"SINGLE" ("data"), 2:i16 0 ("mode (0)")) -> (6:w1593:errorcluster)  [unwired: 2 in, 1 out]
                    }
                    frame #1 {
                      n944 = while {
                        tunnel: w1596 -> [w1597]
                        i -> [w1598]
                        stop <- w1600 continue-if-true
                        n945 = GPIB Serial Poll(0:w1597) -> (2:w1602:i16)  [unwired: 1 in, 2 out]
                        n946 = Less?(x=w1602, y=i16 128) -> (x < y?=w1600:bool)
                        n947 = Wait (ms)(milliseconds to wait=u32 50) -> ()  [unwired: 1 out]
                        "Numeric 3" <- w1598
                      }
                    }
                    frame #2 {
                      w1603 = i16 2 ("mode (0)")
                      n948 = GPIB Read(0:w1605, 1:200 ("byte count"), 2:i16 2 ("mode (0)"), 3:w1616) -> (5:w1609:string)  [unwired: 1 in, 2 out]
                      n949 = Match Pattern(string=w1609, regular expression="C=") -> (after substring=w1608:string)  [unwired: 1 in, 3 out]
                      n950 = Match Pattern(string=w1608, regular expression="PF L=") -> (after substring=w1606:string)  [unwired: 1 in, 3 out]
                      n951 = Search/Split String(string=w1608, search string/char (-)=" ", offset (0)=w1603) -> (substring before match=w1613:string)  [unwired: 2 out]
                      n952 = Search/Split String(string=w1606, search string/char (-)=" ", offset (0)=w1603) -> (substring before match=w1612:string)  [unwired: 2 out]
                      n953 = Fract/Exp String To Number(string=w1612) -> (number=w1610:dbl)  [unwired: 3 in, 1 out]
                      n954 = Fract/Exp String To Number(string=w1613) -> (number=w1611:dbl)  [unwired: 3 in, 1 out]
                    }
                  }
                  n955 = Build Array (concatenate)(w1591, w1589) -> (w1588:dbl[])
                  n956 = Build Array (concatenate)(w1588, w1586) -> (w1587:dbl[])
                }
              }
              n957 = property on="array for data" class="Arr (strict)"("Value"=w1583) -> ()  [unwired: 2 in, 2 out]
            }
          }
        }
      }
      n958 = property on="array for data" class="Arr (strict)"(error in=w447) -> ("Value"=w425:dbl[])  [unwired: 1 in, 2 out]
      n959 = while {
        shift-right: [w1633] -> w421
        shift-left: w425 -> [w1635]
        i -> [w1634]
        stop <- w1638 stop-if-true
        # "loop goes through the list of all measured parameters\nif some columns are identified as current or resistance\nthey are recalculated according to selected or entered parameters"
        n960 = Increment(x=w1634) -> (x+1=w1639:i32)
        n961 = property on="Ring" class="Ring (strict)"() -> ("Strings []"=w1637:string[])  [unwired: 2 in, 2 out]
        n962 = Index Array(array=w1637, index=w1634) -> (element=w1636:string)
        n963 = property on="Ring" class="Ring (strict)"() -> ("NumItems"=w1640:u32)  [unwired: 2 in, 2 out]
        n964 = case shown="\"R1\", \"R1oop\", \"R2\", \"R2oop\", \"R3\", \"R3oop\", \"R4\", \"R4oop\", \"R5\", \"R5oop\"" w1636 {
          tunnel: w1635 -> [w1646 w1656 w1666 w1673]
          tunnel: w1634 -> [w1644 w1653 w1664 _]
          tunnel: [w1645 w1654 w1665 w1673] -> w1633
          frame "I" {
            n965 = property on="Current is:" class="RadioBtnsControl (strict)"() -> ("Value"=w1642:T1)  [unwired: 2 in, 2 out]
            n966 = case shown="\"Radio Selection 1\"" w1642 {
              tunnel: ["Ring 3" "Ring 2"] -> w1641
              frame "Radio Selection 3", Default {
              }
              frame "Radio Selection 1" {
              }
            }
            n967 = Index Array(array=w1646, index=w1644) -> (element=w1647:dbl)
            n968 = Power Of 10(x=w1641) -> (10^x=w1650:dbl)
            n969 = Multiply(x=1000.0, y=w1650) -> (x*y=w1648:dbl)
            n970 = Divide(x=w1647, y=w1648) -> (x/y=w1643:dbl)
            "Numeric Current" <- w1643
            n971 = Replace Array Subset(array=w1646, new element=w1643, index=w1644) -> (w1645:dbl[])
          }
          frame "Ioop" {
            n972 = property on="Ring 3" class="Ring (strict)"() -> ("Value"=w1655:u16)  [unwired: 2 in, 2 out]
            n973 = Index Array(array=w1656, index=w1653) -> (element=w1658:dbl)
            n974 = Power Of 10(x=w1655) -> (10^x=w1661:dbl)
            n975 = Multiply(x=1000.0, y=w1661) -> (x*y=w1659:dbl)
            n976 = Divide(x=w1658, y=w1659) -> (x/y=w1657:dbl)
            n977 = Replace Array Subset(array=w1656, new element=w1657, index=w1653) -> (w1654:dbl[])
          }
          frame "R1", "R1oop", "R2", "R2oop", "R3", "R3oop", "R4", "R4oop", "R5", "R5oop" {
            n978 = property on="Current is:" class="RadioBtnsControl (strict)"() -> ("Value"=w1663:T1)  [unwired: 2 in, 2 out]
            n979 = case shown="\"Radio Selection 2\", Default" w1663 {
              tunnel: [w1669 w1670] -> w1662
              frame "Radio Selection 1" {
                n980 = property on="Numeric Current" class="DigNum (strict)"() -> ("Value"=w1669:dbl)  [unwired: 2 in, 2 out]
              }
              frame "Radio Selection 2", Default {
                n981 = Divide(x="Fixed Current mkA", y=1000000.0) -> (x/y=w1670:dbl)
              }
            }
            n982 = Index Array(array=w1666, index=w1664) -> (element=w1668:dbl)
            n983 = Divide(x=w1668, y=w1662) -> (x/y=w1667:dbl)
            n984 = Replace Array Subset(array=w1666, new element=w1667, index=w1664) -> (w1665:dbl[])
          }
          frame "False", Default {
          }
        }
        n985 = Less?(x=w1640, y=w1639) -> (x < y?=w1638:bool)
      }
      n986 = Subtract(x="Target Field, T", y=w431) -> (x-y=w434:dbl)
      n987 = Divide(x="Sweep rate, T/min", y=60.0) -> (x/y=w443:dbl)
      n988 = Multiply(x=w443, y="Time btw \npoints, sec") -> (x*y=w426:dbl)
      n989 = Sign(1:w434) -> (0:w427:dbl)
      n990 = Multiply(x=w427, y=w426) -> (x*y=w412:dbl)
      n991 = property on="Commutator" class="Bool (strict)"() -> ("Value"=w414:bool)  [unwired: 2 in, 2 out]
      n992 = property on="Data file:" class="Path"() -> ("Value"=w423:path)  [unwired: 2 in, 2 out]
      n993 = Divide(x=w434, y=w412) -> (x/y=w441:dbl)
      n994 = case shown="False" w414 {
        tunnel: w428 -> [w461 w472]
        tunnel: w416 -> [w456 w469]
        tunnel: [w448 w465] -> w413
        frame True {
          # "calculate deliberate time delay for the next step"
          n995 = Subtract(x=w461, y=w456) -> (x-y=w454:u32)
          n996 = property on="Delib Time delay" class="DigNum (strict)"() -> ("Value"=w455:i32)  [unwired: 2 in, 2 out]
          n997 = property on="Time btw \npoints, sec" class="DigNum (strict)"() -> ("Value"=w460:dbl)  [unwired: 2 in, 2 out]
          n998 = Subtract(x=w454, y=w455) -> (x-y=w453:u32)
          n999 = Multiply(x=w460, y=1000.0) -> (x*y=w458:dbl)
          n1000 = To Long Integer(number=w458) -> (32bit integer=w457:i32)
          n1001 = Greater?(x=w457, y=w453) -> (0:w450:bool)
          n1002 = Subtract(x=w457, y=w453) -> (x-y=w452:u32)
          n1003 = Divide(x=w452, y=2) -> (x/y=w449:dbl)
          n1004 = case shown="False" w450 {
            tunnel: w449 -> [_ w464]
            tunnel: [0 w463] -> w448
            frame False {
            }
            frame True {
              n1005 = To Long Integer(number=w464) -> (32bit integer=w463:i32)
            }
          }
        }
        frame False {
          n1006 = property on="Time btw \npoints, sec" class="DigNum (strict)"() -> ("Value"=w467:dbl)  [unwired: 2 in, 2 out]
          n1007 = Multiply(x=w467, y=1000.0) -> (x*y=w468:dbl)
          n1008 = Subtract(x=w472, y=w469) -> (x-y=w470:u32)
          n1009 = Greater?(x=w468, y=w470) -> ()  [unwired: 1 out]
          n1010 = Subtract(x=w468, y=w470) -> (x-y=w466:dbl)
          n1011 = To Long Integer(number=w466) -> (32bit integer=w465:i32)
        }
      }
      "Delib Time delay" <- w413
      n1012 = Decrement(x=w441) -> (x-1=w440:dbl)
      n1013 = Absolute Value(x=w434) -> (abs(x)=w436:dbl)
      n1014 = Build Array (concatenate)(w446, w421) -> (w420:dbl[][])
      n1015 = Greater Than 0?(x=w440) -> (x > 0?=w439:bool)
      n1016 = property on="array for data" class="Arr (strict)"("Value"=w421) -> ()  [unwired: 2 in, 2 out]
      n1017 = call-poly <vilib>:"Write To Spreadsheet File.vi"("format (%.3f)"="%#g", "append to file? (new file:F)"=TRUE, "1D data"=w421, "file path (dialog if empty)"=w423) -> ()  [unwired: 4 in, 1 out]
      n1018 = Less?(x=w436, y=1e-06) -> (x < y?=w433:bool)
      n1019 = flat-sequence {
        tunnel: [w1632] -> w428
        tunnel: w420 -> [w1626]
        frame #0 {
          # "time is mesured at the end of the cycle\nto adjust a delay time"
          # "this part plots selected measurements"
          n1020 = Tick Count (ms)() -> (millisecond timer value=w1632:u32)
          n1021 = Index Array(array=w1626, index (col)="Ring") -> (element=w1631:dbl[])  [unwired: 1 in]
          n1022 = Index Array(array=w1626, index (col)=0) -> (element=w1629:dbl[])  [unwired: 1 in]
          n1023 = Bundle(w1629, w1631) -> (→"XY Graph":cluster{dbl[], dbl[]})  [unwired: 1 in]
        }
      }
      n1024 = case shown="False" w439 {
        tunnel: w431 -> [_ w1677]
        tunnel: w412 -> [_ w1676]
        tunnel: [w1674 w1675] -> w438
        frame False {
          # "if next step is too long\nuse target voltage"
          n1025 = property on="Target Field, T" class="DigNum (strict)"() -> ("Value"=w1674:dbl)  [unwired: 2 in, 2 out]
        }
        frame True {
          # "add increment to\nthe current Vg"
          n1026 = Add(x=w1676, y=w1677) -> (x+y=w1675:dbl)
        }
      }
    }
  }
  n1027 = Concatenate Strings(w9, w5, w6, w5, w6, w4, w5, w6) -> (w18:string)
  "String" <- w18
  n1028 = Write to Text File(file (use dialog)=w19, text=w18) -> ()  [unwired: 2 in, 3 out]
  n1029 = property on="Time btw \npoints, sec" class="DigNum (strict)" props=["Value"]() -> ()  [unwired: 2 in, 3 out]
  n1030 = flat-sequence {
    tunnel: w16 -> [w1680]
    frame #0 {
      (unwired) FALSE
      (unwired) i32[][] []
      n1031 = To Time Stamp(1:0) -> (0:w1678:timestamp)
      n1032 = property on="Time Stamp" class="AbsTime (strict)"("Value"=w1678) -> ()  [unwired: 2 in, 2 out]
      "Array 2" <- w1680
    }
  }
